vi "Sievert_auto_RLC-2.vi"() -> ()   [LabVIEW 2011]
uses:
  <vilib>/Utility/error.llb/DialogType.ctl
  <vilib>/DAQmx/write.llb/DAQmx Write (Digital Bool 1Line 1Point).vi
  <vilib>/DAQmx/create/channels.llb/DAQmx Create Channel (DO-Digital Output).vi
  <vilib>/DAQmx/miscellaneous.llb/DAQmx Fill In Error Info.vi
  <vilib>/Analysis/Matrix/Numeric/Conversions/Array To Matrix - RA.vi
  <vilib>/Analysis/Matrix/Numeric/Conversions/Matrix To Array - RM.vi
  <vilib>/Analysis/NI_AALPro.lvlib
  <vilib>/Analysis/Matrix/NI_Matrix.lvlib
  <vilib>/Analysis/NI_AALBase.lvlib
panel:
  out "Boolean 4":bool
  out "tempo carga":dbl[](array[numeric])
  out "PCh1":dbl[](array[numeric])
  out "output array 2":u32[](array[numeric])
  out "MEASURE C [F ]":dbl
  out "Automatico 2":dynamicdata(graph)
  out "termopar K 2":dbl format="%.3g"
  out "termopar K":string
  out "output NTC":dbl
  out "termopar K":dbl format="%.3g"
  out "path RLC_mean":path
  out "estagio 5":i32
  out "FIM":bool=TRUE
  out "limpo":i32
  in  "N fit":i32=5
  in  "ATM wait":u32
  in  "SET":i32
  in  "time subarray":dbl[](array[numeric])
  out "P cinetica mean 2":dbl format="%0.2f"
  out "T cinetica mean 3":dbl format="%0.2f"
  out "Time cinetica":dbl format="%0.2f"
  in  "T subarray 3":dbl[](array[numeric])
  in  "P T  index 2":i32
  in  "P subarray 2":dbl[](array[numeric])
  in  "Numeric":dbl=4.0
  in  "T subarray 2":dbl[](array[numeric])
  out "T cinetica mean 2":dbl format="%0.2f"
  out "P cinetica mean":dbl format="%0.2f"
  in  "P subarray":dbl[](array[numeric])
  in  "P T  index":i32
  out "T string":string
  out "P string":string
  out "path 2_cinetica":path
  out "Polynomial Coefficients 2":dbl[](array[numeric])
  out "Polynomial Coefficients":dbl[](array[numeric])
  in  "Count SET":i32=-1
  out "Set atual":i32
  out "mean pressure":dbl format="%.4p"
  out "Set number":i32
  in  "Tab Control":T1(tab)
  out "T":bool
  out "ZPf2":bool
  out "Pf2":bool
  out "Pit":bool
  out "ZPit":bool
  out "Camara":dbl(slide) scale=0.0..59.5 scale format="%#_3g"
  in  "Save manual":bool
  in  "Open Button":bool
  out "String 2":string
  in  "ATM":bool
  in  "Câmara":bool
  in  "Vácuo":bool
  in  "Entrada Gás":bool
  in  "Manual Ctrl":bool
  in  "stop":bool
  out "P-manual":dynamicdata(graph)
  in  "Clear":bool
  out "path":path
  in  "Nota":string
  in  "Sample name":string
  in  "File name":string
  out "Linear Model Graph":dbl[][](graph)
  out "Linear Model Graph 2":dbl[][](graph)
  in  "N to fit":i32=60
  out "N":i32
  out "Vácuo":bool
  out "Atm":bool
  out "Câmara":bool
  out "String_cinetica":string
  out "Vol Ref":dbl(slide) scale=0.0..60.0 scale format="%#_4f"
  out "Entrada gás":bool
  in  "Guardar\nCinetica":bool
  out "p fit":dbl format="%#_4g"
  out "T fit":dbl format="%#_4g"
  in  "Open Button 2":bool
  out "x >= y?":bool
  in  "seconds":dbl
  out "Elapsed Time (sec)":dbl format="%.1f"
  out "bar/N":dbl format="%#_4p"
  in  "correção NTC":dbl
  out "mean H2 sensor (V)":dbl format="%#_4p"
  out "Boolean 3":bool
  out "String 3":string
  out "T 2":bool
  out "ZPit 2":bool
  out "Pit 2":bool
  out "Pf2 2":bool
  out "ZPf2 2":bool
  out "Camara 2":dbl(slide) scale=0.0..20.0 scale format="%#_3g"
  out "Vácuo 2":bool
  out "Atm 2":bool
  out "Câmara 2":bool
  out "Vol Ref 3":dbl(slide) scale=0.0..25.0 scale format="%#_4f"
  out "Entrada gás 2":bool
  in  "Auto Ctrl":bool
  in  "Play Button":bool
  out "time stamp":timestamp format="%<%.2X>T"
  out "Time (sec)":dbl format="%.1f"
  in  "clear":bool
  out "Automatico":dynamicdata(graph)
  out "Linear P":T2(graph)
  out "Linear T":T2(graph)
  out "Contador":i32
  in  "STOP (bar/s)":dbl format="%#_5p"
  out "P (bar/s)":dbl format="%#_5p"
  out "bar/s":dbl format="%#_4p"
  out "P fit":dbl format="%#_4g"
  out "T fit":dbl format="%#_4g"
  out "x = y?":bool
  out "teste slope":i32
  in  "Set P auto":dbl
  in  "Step P":dbl=2.0
  in  "P_max":dbl=2.0
  in  "P_max camara":dbl=2.0
  out "Carga":bool=TRUE
  out "Descarga":bool
  out "String":string
  in  "P_min descarga":dbl
  in  "Boolean":bool
  in  "Array":dbl[](array[numeric])
  out "Boolean 2":bool
  out "Desc SET":i32
  in  "ZPf2 time":dbl=24.0
  in  "Ciclos":dbl
  out "Efetuados":dbl
  in  "patamar milliseconds to wait":u32=500
  in  "N fit patamar":i32=100
  in  "Step ZPit":dbl
  out "Read ZPit":bool
  in  "Estagio auto":i32
  out "mean H2 sensor":dbl format="%#_4p"
  in  "Ntest":i32=5
  in  "N fit 2":i32=100
  out "String 4":string
  in  "Combo Box":string(combo)
  in  "Refresh Button":bool
  in  "Close RLC 2":bool
  in  "RLC on/off":bool
  out "mean 16":dbl format="%.3p"
  out "mean 15":dbl format="%.3p"
  out "mean 14":dbl format="%.3p"
  out "mean 13":dbl format="%.3p"
  out "mean 12":dbl format="%.3p"
  out "mean 11":dbl format="%.3p"
  out "mean 10":dbl format="%.3p"
  out "mean 9":dbl format="%.3p"
  out "mean 8":dbl format="%.3p"
  out "mean 7":dbl format="%.3p"
  out "mean 6":dbl format="%.3p"
  out "mean 5":dbl format="%.3p"
  out "mean 4":dbl format="%.3p"
  out "mean 3":dbl format="%.3p"
  out "mean 2":dbl format="%.3p"
  out "mean":dbl format="%.3p"
  out "SET 2":dbl format="%#_3g"
  out "C-50-L":bool
  out "MEASURE B":dbl
  out "MEASURE A":dbl
  out "C-50-N":bool
  out "MEASURE B 2":dbl
  out "MEASURE A 2":dbl
  out "C-100-L":bool
  out "MEASURE B 3":dbl
  out "MEASURE A 3":dbl
  out "C-100-N":bool
  out "MEASURE B 4":dbl
  out "MEASURE A 4":dbl
  out "C-1K-L":bool
  out "MEASURE B 5":dbl
  out "MEASURE A 5":dbl
  out "C-1K-N":bool
  out "MEASURE B 6":dbl
  out "MEASURE A 6":dbl
  out "C-10K-L":bool
  out "MEASURE B 7":dbl
  out "MEASURE A 7":dbl
  out "C-10K-N":bool
  out "MEASURE B 8":dbl
  out "MEASURE A 8":dbl
  out "Z-50-L":bool
  out "MEASURE B 9":dbl
  out "MEASURE A 9":dbl
  out "Z-50-N":bool
  out "MEASURE B 10":dbl
  out "MEASURE A 10":dbl
  out "Z-100-L":bool
  out "MEASURE B 11":dbl
  out "MEASURE A 11":dbl
  out "Z-100-N":bool
  out "MEASURE B 12":dbl
  out "MEASURE A 12":dbl
  out "Z-1K-L":bool
  out "MEASURE B 13":dbl
  out "MEASURE A 13":dbl
  out "Z-1K-N":bool
  out "MEASURE B 14":dbl
  out "MEASURE A 14":dbl
  out "Z-10K-L":bool
  out "MEASURE B 15":dbl
  out "MEASURE A 15":dbl
  out "Z-10K-N":bool
  out "MEASURE B 16":dbl
  out "MEASURE A 16":dbl
  out "RLC300 - digimess":string
  in  "Time RLC":u32=5000
  in  "Ligar RLC":bool
  out "path RLC_completo":path
  out "Waveform Chart P 2":dbl[][](graph)
  out "Waveform Chart":dynamicdata(graph)
  in  "graph RLC":bool
  in  "Refresh Button 2":bool
  out "Waveform Chart 2":dynamicdata(graph)
  out "XY Graph 2":cluster{"Value":dbl[], "Value":dbl[]}[](graph)
  in  "t-sivert01(s)":dbl
  out "dP/dt (bar/s)":dbl format="%#_5p"
  in  "read - Sievert 01":bool
  # "P vol ref"
  # "P Câmara"
  # "P vol ref"
  # "P Câmara"
  # "C ( F )"
  # "R ( Ohm )"
  # "Z ( Ohm )"
  # "Phase ( deg)"
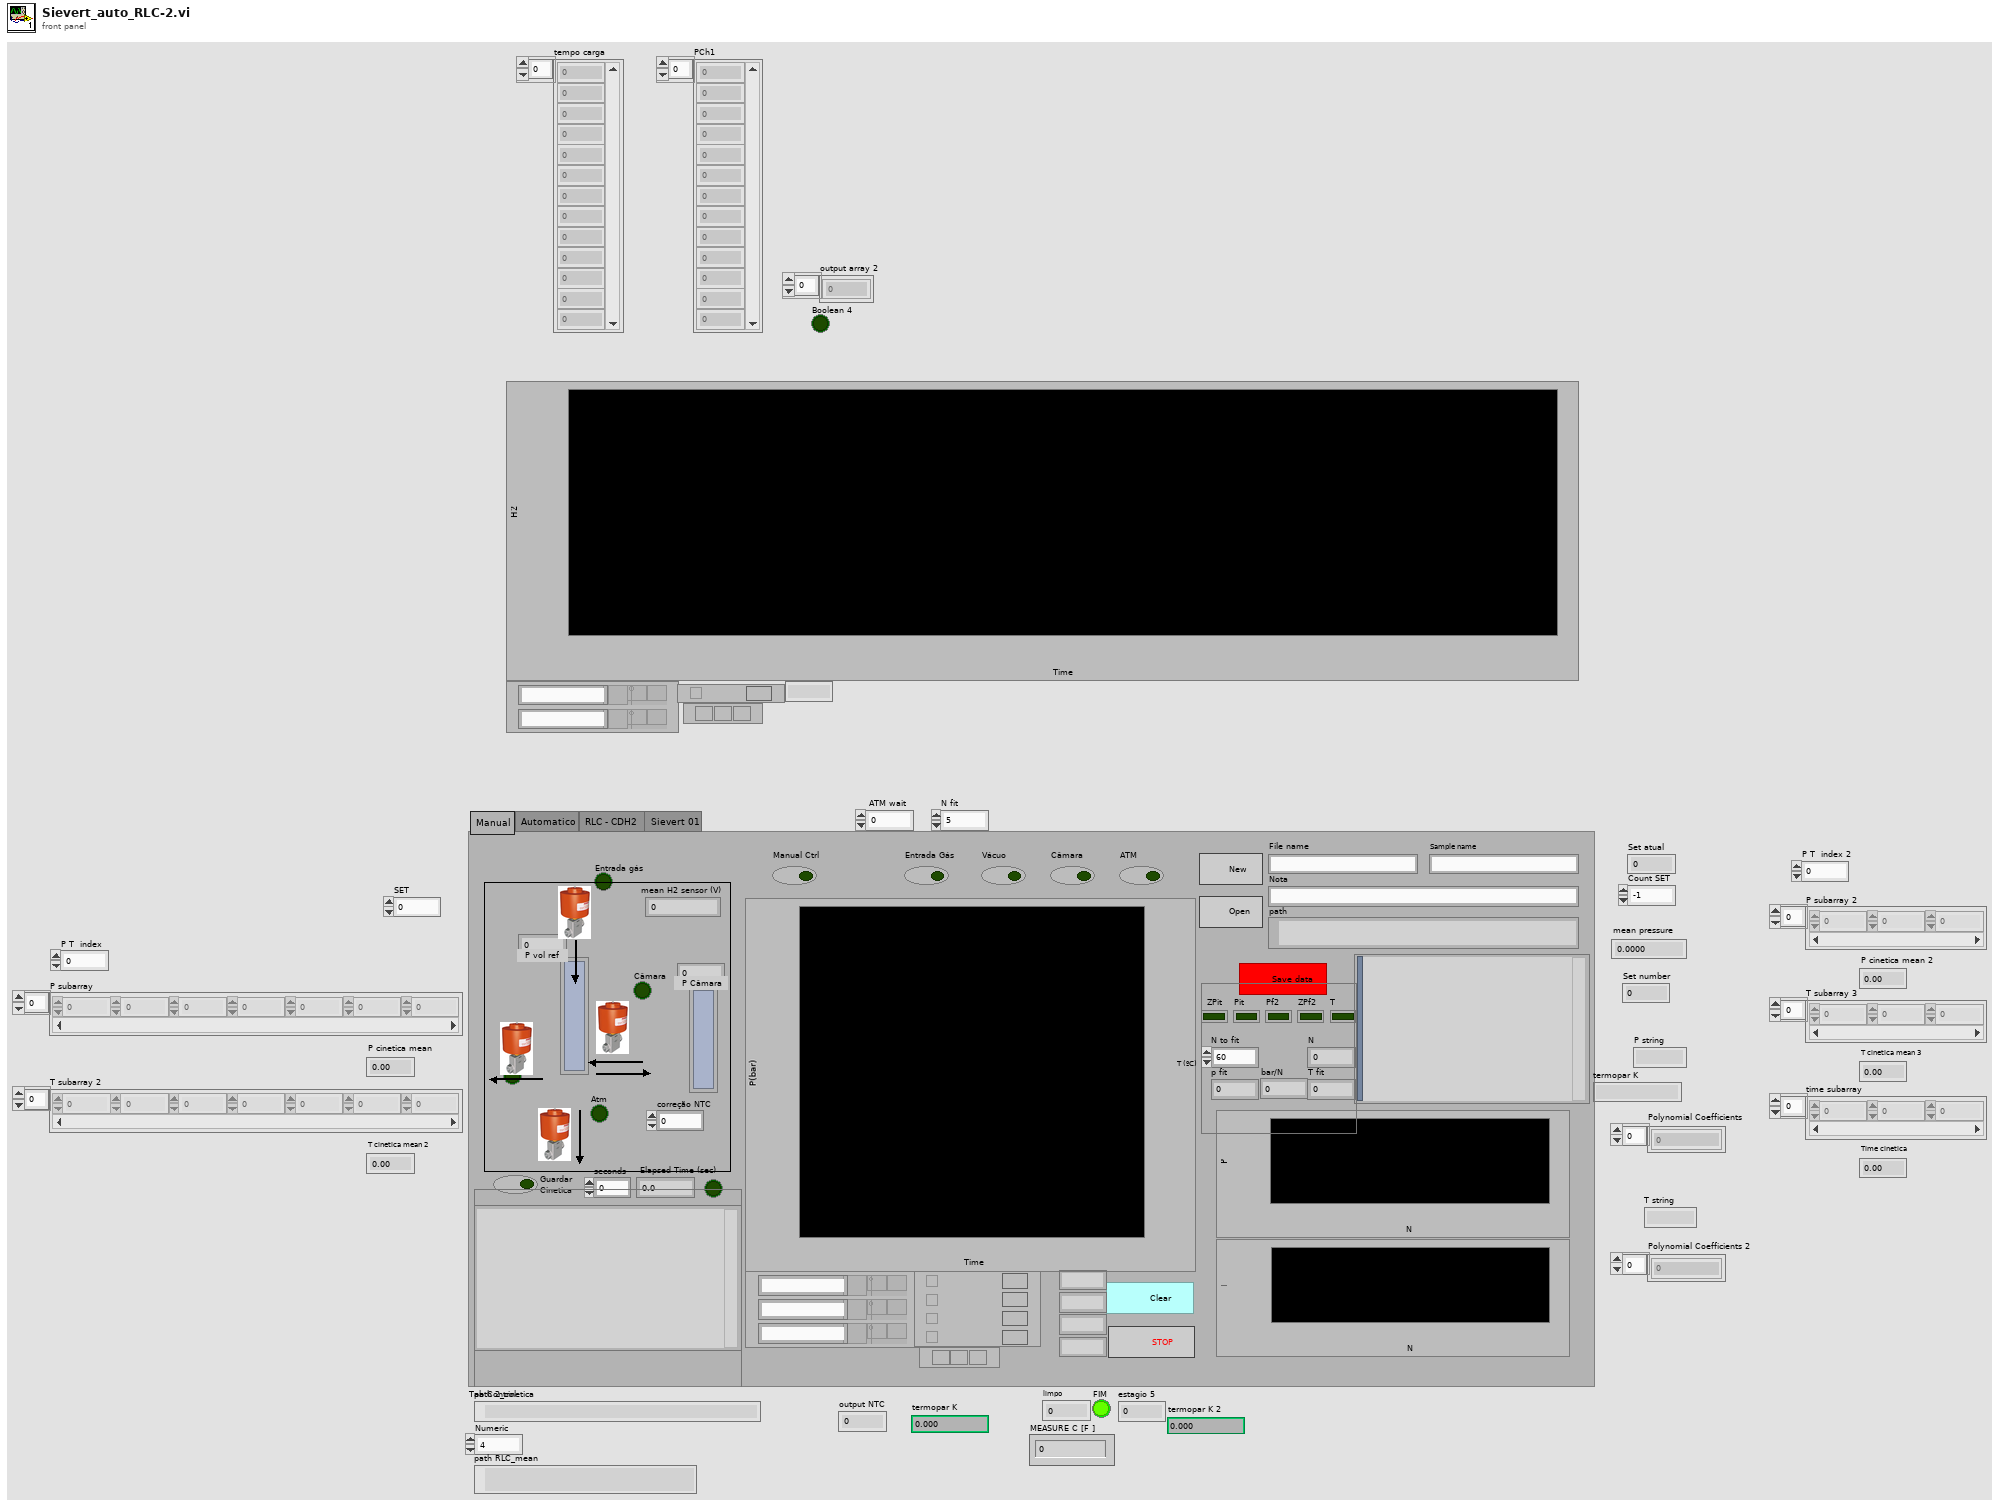
[diagram p1: front panel]
types:
  T1 = enum32{"Manual", "Automatico", "RLC - CDH2", "Sievert 01"}
  T2 = cluster{"Real 2D Array":dbl[], "Best Linear Fit":dbl[]}[]
  T3 = enum16{"open", "replace", "create", "open or create", "replace or create", "replace or create with confirmation"}
  T4 = cluster{"Value":dbl[], "Best Linear Fit":dbl[]}[]
  T5 = typedef "NI_Matrix.lvlib/RealMatrix.ctl" = dbl[][]
  T6 = cluster{"Real 2D Array":dbl[], "Real 2D Array":dbl[]}
  T7 = typedef "DialogType.ctl" = u16
  T8 = cluster{"Real 2D Array":dbl[], "Best Linear Fit":dbl[]}
  T9 = cluster{"Real 2D Array":dbl[], "Best Polynomial Fit":dbl[]}
  T10 = cluster{"Real 2D Array":dbl[], "Best Polynomial Fit":dbl[]}[]
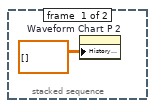
[diagram p5: hidden frame]
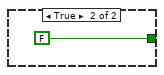
[diagram p10: hidden frame]
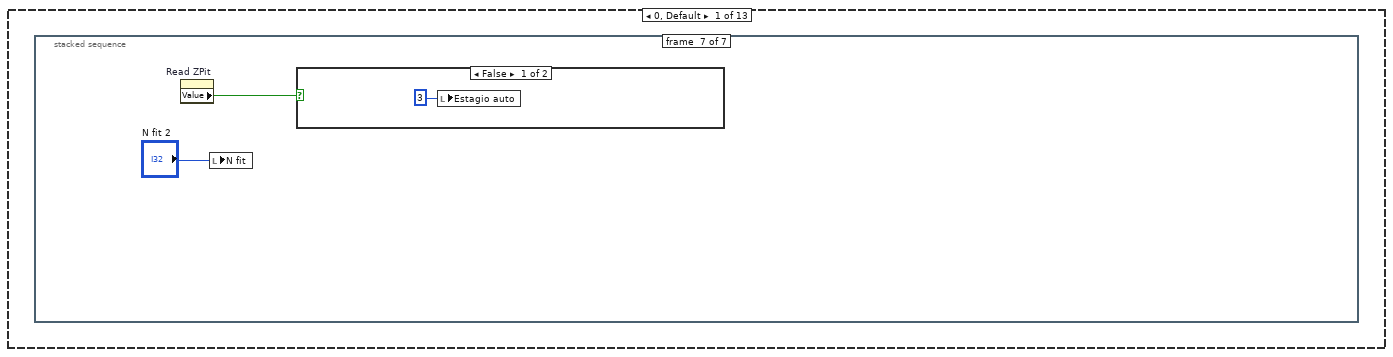
[diagram p15: hidden frame]
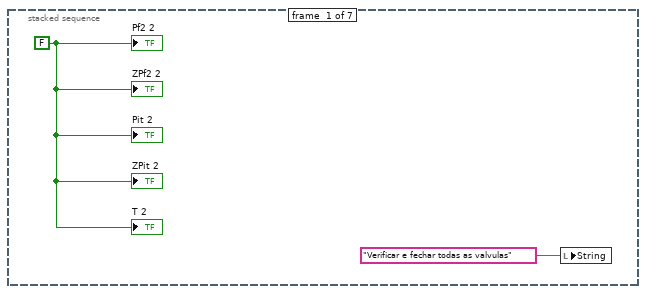
[diagram p16: hidden frame]
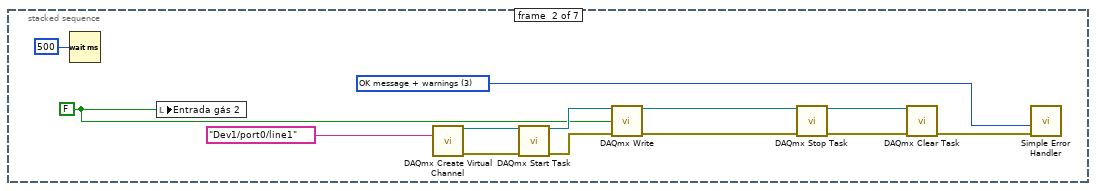
[diagram p17: hidden frame]
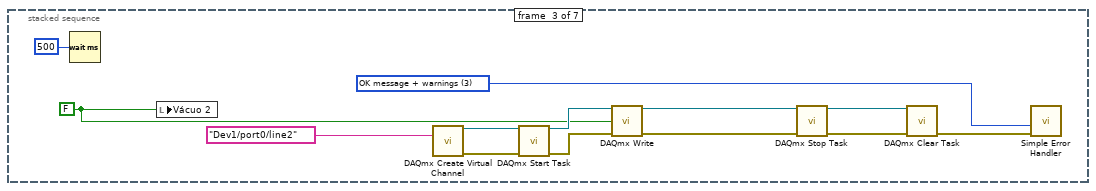
[diagram p18: hidden frame]
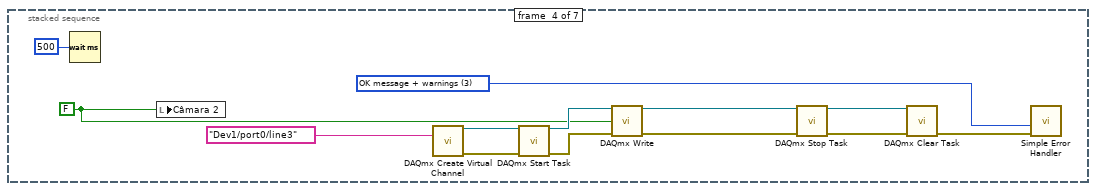
[diagram p19: hidden frame]
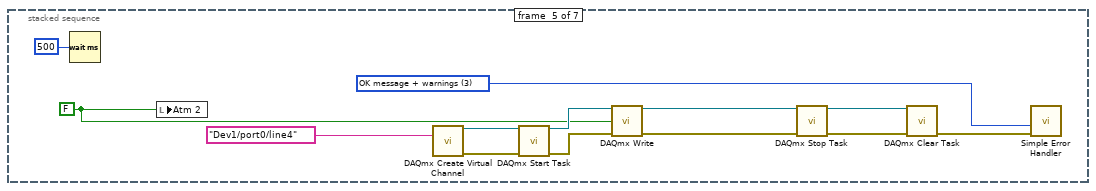
[diagram p20: hidden frame]
diagram:
  (unwired) dbl[] [0.5, 1.0, 2.0, 3.0, 4.0, 5.0, 6.0, 7.0, 8.0, 9.0, 10.0, 11.0, 12.0, 13.0, 14.0, 15.0, 16.0, 17.0, 18.0, 19.0, 20.0, 30.0, 40.0, 50.0, 60.0, 70.0] ("Array")
  n1 = local write "N to fit"(5 ("Numeric")) -> ()
  n2 = local write "correção NTC"(0.5 ("correção NTC")) -> ()
  n3 = local write "Step ZPit"(5.0 ("Step ZPit")) -> ()
  n4 = local write "Time RLC"(u32 5 ("Time RLC")) -> ()
  n5 = local write "Ciclos"(0.0 ("Ciclos")) -> ()
  n6 = local write "Desc SET"(0 ("Desc SET")) -> ()
  n7 = local write "Efetuados"(0.0 ("Efetuados")) -> ()
  n8 = local write "estagio 5"(0 ("estagio 5")) -> ()
  n9 = local write "teste slope"(0 ("teste slope")) -> ()
  n10 = local write "SET"(0 ("SET auto")) -> ()
  n11 = local write "limpo"(0 ("limpo")) -> ()
  n12 = local write "N fit"(5 ("N fit")) -> ()
  n13 = local write "ATM wait"(u32 4 ("ATM wait")) -> ()
  n14 = local write "Estagio auto"(0 ("Estagio auto")) -> ()
  n15 = local write "P T  index"(0 ("index")) -> ()
  n16 = local write "seconds"(2.0 ("seconds")) -> ()
  n17 = local write "Read ZPit"(TRUE ("Read ZPit")) -> ()
  n18 = local write "Descarga"(FALSE ("Descarga")) -> ()
  n19 = local write "Carga"(TRUE ("Carga")) -> ()
  n20 = local write "FIM"(FALSE ("FIM")) -> ()
  n21 = local write "P_max"(50.0 ("P_max")) -> ()
  n22 = local write "P_max camara"(25.0 ("P_max camara")) -> ()
  n23 = local write "Set P auto"(0.5 ("Set P auto")) -> ()
  n24 = local write "P_min descarga"(0.025 ("P_min descarga")) -> ()
  n25 = local write "P subarray"(dbl[] [0.0, 1.0] ("subarray")) -> ()
  n26 = local write "T subarray 2"(dbl[] [0.0, 1.0] ("subarray")) -> ()
  n27 = local write "Combo Box"("rlc_read_cCN.py" ("Combo Box")) -> ()
  n28 = local write "t-sivert01(s)"(10.0 ("t-sivert01(s)")) -> ()
  n29 = while {
    tunnel: path "C:/H2_Painel/painel_auto/RLC_CDH" ("Path") -> [w36]
    stop <- w48 stop-if-true
    n30 = property on="FIM" class="Bool (strict)"() -> ("Value"=w46:bool)  [unwired: 2 in, 2 out]
    n31 = property on="path" class="Path"() -> ("Value"=w43:path)  [unwired: 2 in, 2 out]
    n32 = case shown="True" "Ligar RLC" {
      tunnel: w36 -> [_ w223]
      frame False {
      }
      frame True {
        n33 = call "RLC_open.vi"("Path"=w223) -> ("String 2"=w224:string)  [unwired: 9 in, 1 out]
        n34 = local write "RLC300 - digimess"(w224) -> ()
      }
    }
    n35 = case shown="True" "Auto Ctrl" {
      tunnel: w36 -> [_ w229]
      tunnel: "RLC on/off" -> [_ w228]
      tunnel: [_ w227] -> w39
      frame False {
      }
      frame True {
        n36 = local write "P T  index 2"(0 ("P T  index")) -> ()
        n37 = for {
          N: "N fit" -> [w256]
          tunnel: w229 -> [w247]
          tunnel: w228 -> [w246]
          tunnel: [w245] -> w227
          i -> [w258]
          w262 = 0 ("polynomial order")
          w253 = 0 ("polynomial order")
          n38 = case shown="True" "clear" {
            frame False {
            }
            frame True {
              n39 = property on="Automatico 2" class="WFChart (strict)"("History Data"=dynamicdata[] []) -> ()  [unwired: 2 in, 2 out]
              n40 = property on="Linear P" class="XYGraph (strict)"("Value"=T2 [] ("Linear P")) -> ()  [unwired: 2 in, 2 out]
              n41 = property on="Linear T" class="XYGraph (strict)"("Value"=T2 [] ("Linear T")) -> ()  [unwired: 2 in, 2 out]
              n42 = property on="Automatico" class="WFChart (strict)"("History Data"=dynamicdata[] []) -> ()  [unwired: 2 in, 2 out]
            }
          }
          n43 = property on="path 2_cinetica" class="Path"() -> ("Value"=w250:path)  [unwired: 2 in, 2 out]
          n44 = call "Read P T.vi"("correção NTC"="correção NTC") -> ("Sievert01"=w237:dbl, "mean H2 sensor"=w242:dbl, "termopar K"=w239:dbl, "output NTC"=w240:dbl, "P Set 2 Output 2"=w241:dbl)  [unwired: 3 in, 7 out]
          "termopar K 2" <- w239
          "mean H2 sensor" <- w242
          n45 = Increment(x=w258) -> (x+1=w257:i32)
          n46 = Equal?(x=w257, y=w256) -> (x = y?=w259:bool)
          "x = y?" <- w259
          n47 = Merge Signals(w242) -> (→"Automatico 2":dynamicdata)
          n48 = Multiply(x=w241, y=10.0) -> (x*y=w252:dbl)
          n49 = Multiply(x=w237, y=10.0) -> (x*y=w236:dbl)
          n50 = case shown="True" "read - Sievert 01" {
            tunnel: w236 -> [_ w285]
            frame False {
            }
            frame True {
              n51 = Merge Signals(w285) -> (→"Waveform Chart 2":dynamicdata)
              n52 = flat-sequence {
                tunnel: w285 -> [w302]
                tunnel: [w300] -> w287
                frame #0 {
                  n53 = property on="Boolean 4" class="Bool (strict)"() -> ("Value"=w288:bool)  [unwired: 2 in, 2 out]
                  n54 = case shown="True" w288 {
                    frame False {
                    }
                    frame True {
                      n55 = local write "PCh1"(dbl[] [] ("PCh1")) -> ()
                      n56 = local write "tempo carga"(dbl[] [] ("tempo carga")) -> ()
                      n57 = local write "output array 2"(u32[] [] ("output array 2")) -> ()
                    }
                  }
                }
                frame #1 {
                  n58 = Tick Count (ms)() -> (millisecond timer value=w313:u32)
                  n59 = property on="output array 2" class="Arr (strict)"() -> ("Value"=w314:u32[])  [unwired: 2 in, 2 out]
                  n60 = Build Array(w313) -> (w307:u32[])
                  n61 = Insert Into Array(array=w314, new element=w307) -> (w308:u32[])  [unwired: 1 in]
                  "output array 2" <- w308
                  n62 = Array Max & Min(array=w308) -> (max value=w312:u32, min value=w311:u32)  [unwired: 2 out]
                  n63 = Subtract(x=w312, y=w311) -> (x-y=w309:u32)
                  n64 = Divide(x=w309, y=1000.0) -> (x/y=w299:dbl)
                  n65 = property on="PCh1" class="Arr (strict)"() -> ("Value"=w304:dbl[])  [unwired: 2 in, 2 out]
                  n66 = property on="tempo carga" class="Arr (strict)"() -> ("Value"=w305:dbl[])  [unwired: 2 in, 2 out]
                  n67 = Greater?(x=w299, y="t-sivert01(s)") -> (0:w300:bool)
                  n68 = Build Array(w299) -> (w306:dbl[])
                  n69 = Build Array(w302) -> (w303:dbl[])
                  n70 = Insert Into Array(array=w305, new element=w306) -> (w294:dbl[])  [unwired: 1 in]
                  "tempo carga" <- w294
                  n71 = Insert Into Array(array=w304, new element=w303) -> (w293:dbl[])  [unwired: 1 in]
                  "PCh1" <- w293
                  n72 = call <vilib>:"Linear Fit.vi"("Y"=w293, "X"=w294) -> ("Best Linear Fit"=w292:dbl[], "slope"=→"dP/dt (bar/s)":dbl)  [unwired: 9 in, 3 out]
                  n73 = Bundle("Value"=w294, "Value"=w293) -> (w297:cluster{"Value":dbl[], "Value":dbl[]})  [unwired: 1 in]
                  n74 = Bundle("Value"=w294, "Best Linear Fit"=w292) -> (w296:cluster{"Value":dbl[], "Best Linear Fit":dbl[]})  [unwired: 1 in]
                  n75 = Build Array(w297, w296) -> (→"XY Graph 2":T4)
                }
              }
              "Boolean 4" <- w287
            }
          }
          n76 = local write "Vol Ref 3"(w252) -> ()
          n77 = Merge Signals(w252, w240, w239, w236) -> (→"Automatico":dynamicdata)
          n78 = call "Elapsed Time2"("Reset"=w259) -> ("Elapsed Time (s)"=w273:dbl)  [unwired: 11 in, 7 out]
          "Time (sec)" <- w273
          n79 = stacked-sequence {
            tunnel: w252 -> [w1623 _]
            tunnel: w240 -> [w1609 _]
            tunnel: [w1590 _] -> w271
            tunnel: [w1606 _] -> w270
            tunnel: w273 -> [w1593 _]
            tunnel: [w1591 _] -> w267
            tunnel: [w1589 _] -> w249
            tunnel: [w1588 _] -> w248
            frame #0 {
              w1592 = 2 ("y")
              n80 = property on="P subarray 2" class="Arr (strict)"() -> ("Value"=w1625:dbl[])  [unwired: 2 in, 2 out]
              n81 = property on="T subarray 3" class="Arr (strict)"() -> ("Value"=w1615:dbl[])  [unwired: 2 in, 2 out]
              n82 = property on="time subarray" class="Arr (strict)"() -> ("Value"=w1602:dbl[])  [unwired: 2 in, 2 out]
              n83 = property on="P T  index 2" class="DigNum (strict)"() -> ("Value"=w1594:i32)  [unwired: 2 in, 2 out]
              n84 = Replace Array Subset(array=w1602, new element=w1593, index=w1594) -> (w1595:dbl[])
              n85 = Replace Array Subset(array=w1625, new element=w1623, index=w1594) -> (w1608:dbl[])
              n86 = Replace Array Subset(array=w1615, new element=w1609, index=w1594) -> (w1607:dbl[])
              n87 = call-poly <vilib>:"Array To Matrix.vi"("Real 1D Array"=w1595) -> ("Real Matrix (Column Vector)"=w1605:T5)
              n88 = call-poly <vilib>:"Array To Matrix.vi"("Real 1D Array"=w1608) -> ("Real Matrix (Column Vector)"=w1628:T5)
              n89 = call-poly <vilib>:"Array To Matrix.vi"("Real 1D Array"=w1607) -> ("Real Matrix (Column Vector)"=w1618:T5)
              n90 = Matrix Size(0:w1605) -> (1:w1604:i32, 2:w1603:i32)
              n91 = Matrix Size(0:w1628) -> (1:w1627:i32, 2:w1626:i32)
              n92 = Matrix Size(0:w1618) -> (1:w1617:i32, 2:w1616:i32)
              n93 = Increment(x=w1604) -> (x+1=w1596:i32)
              n94 = Increment(x=w1627) -> (x+1=w1619:i32)
              n95 = Increment(x=w1617) -> (x+1=w1610:i32)
              n96 = Subtract(x=w1596, y=w1592) -> (x-y=w1597:i32)
              n97 = Subtract(x=w1619, y=w1592) -> (x-y=w1620:i32)
              n98 = Subtract(x=w1610, y=w1592) -> (x-y=w1611:i32)
              n99 = Resize Matrix(1:w1603, 2:w1596, 4:w1605) -> (0:w1601:T5)
              n100 = Resize Matrix(1:w1626, 2:w1619, 4:w1628) -> (0:w1624:T5)
              n101 = Resize Matrix(1:w1616, 2:w1610, 4:w1618) -> (0:w1614:T5)
              n102 = call-poly <vilib>:"Matrix To Array.vi"("Real Matrix"=w1601) -> ("Real 2D Array"=w1599:dbl[][])
              n103 = call-poly <vilib>:"Matrix To Array.vi"("Real Matrix"=w1624) -> ("Real 2D Array"=w1622:dbl[][])
              n104 = call-poly <vilib>:"Matrix To Array.vi"("Real Matrix"=w1614) -> ("Real 2D Array"=w1613:dbl[][])
              n105 = Reshape Array(w1599, w1596) -> (w1598:dbl[])
              n106 = Reshape Array(w1622, w1619) -> (w1621:dbl[])
              n107 = Reshape Array(w1613, w1610) -> (w1612:dbl[])
              n108 = local write "time subarray"(w1598) -> ()
              n109 = local write "P subarray 2"(w1621) -> ()
              n110 = local write "T subarray 3"(w1612) -> ()
              n111 = Reshape Array(w1598, w1597) -> (w1591:dbl[])
              n112 = Reshape Array(w1621, w1620) -> (w1590:dbl[])
              n113 = Reshape Array(w1612, w1611) -> (w1606:dbl[])
              n114 = call <vilib>:"Mean.vi"("X"=w1591) -> ("mean"=→"Time cinetica":dbl)  [unwired: 1 out]
              n115 = call <vilib>:"Mean.vi"("X"=w1590) -> ("mean"=w1589:dbl)  [unwired: 1 out]
              "P cinetica mean 2" <- w1589
              n116 = call <vilib>:"Mean.vi"("X"=w1606) -> ("mean"=w1588:dbl)  [unwired: 1 out]
              "T cinetica mean 3" <- w1588
            }
            frame #1 {
              n117 = property on="P T  index 2" class="DigNum (strict)"() -> ("Value"=w1630:i32)  [unwired: 2 in, 2 out]
              n118 = Increment(x=w1630) -> (x+1=w1629:i32)
              n119 = local write "P T  index 2"(w1629) -> ()
            }
          }
          n120 = To Time Stamp(1:w273) -> (0:→"time stamp":timestamp)
          n121 = call <vilib>:"Linear Fit.vi"("Y"=w270, "X"=w267) -> ("Best Linear Fit"=w279:dbl[])  [unwired: 9 in, 4 out]
          n122 = Bundle("Real 2D Array"=w267, "Real 2D Array"=w270) -> (w277:T6)  [unwired: 1 in]
          n123 = Bundle("Real 2D Array"=w267, "Real 2D Array"=w271) -> (w276:T6)  [unwired: 1 in]
          n124 = call <vilib>:"General Polynomial Fit.vi"("Y"=w270, "polynomial order"=w253, "X"=w267) -> ("Best Polynomial Fit"=w268:dbl[], "Polynomial Coefficients"=w263:dbl[])  [unwired: 9 in, 2 out]
          n125 = call <vilib>:"General Polynomial Fit.vi"("Y"=w271, "polynomial order"=w253, "X"=w267) -> ("Best Polynomial Fit"=w269:dbl[], "Polynomial Coefficients"=w264:dbl[])  [unwired: 9 in, 2 out]
          n126 = call <vilib>:"Linear Fit.vi"("Y"=w271, "X"=w267) -> ("Best Linear Fit"=w274:dbl[], "slope"=w254:dbl)  [unwired: 9 in, 3 out]
          "bar/s" <- w254
          n127 = property on="path" class="Path"() -> ("Value"=w251:path)  [unwired: 2 in, 2 out]
          n128 = case shown="True" "Play Button" {
            tunnel: w251 -> [_ w323]
            tunnel: w252 -> [_ w322]
            tunnel: w250 -> [_ w321]
            tunnel: w249 -> [_ w320]
            tunnel: w248 -> [_ w319]
            tunnel: w247 -> [_ w318]
            tunnel: w246 -> [_ w317]
            tunnel: [_ w316] -> w245
            tunnel: w239 -> [_ w315]
            frame False {
            }
            frame True {
              n129 = case shown="12" "Estagio auto" {
                tunnel: w323 -> [_ _ _ w415 _ _ w568 _ w717 _ _ w1429 w1498]
                tunnel: w322 -> [_ w389 _ _ w464 w515 _ _ _ w1347 _ _ _]
                tunnel: w321 -> [_ _ _ _ _ _ _ w607 _ _ _ _ _]
                tunnel: w320 -> [_ _ _ _ _ _ _ w606 _ _ _ _ _]
                tunnel: w319 -> [_ _ _ _ _ _ _ w605 _ _ _ _ _]
                tunnel: w318 -> [_ _ _ _ _ _ _ _ w696 _ _ _ _]
                tunnel: w317 -> [_ _ _ _ _ _ _ _ w713 _ _ _ _]
                tunnel: [_ _ _ _ _ _ _ _ w695 _ _ _ _] -> w316
                tunnel: w315 -> [_ _ _ _ _ _ _ _ _ _ _ w1425 _]
                frame 0, Default {
                  n130 = stacked-sequence {
                    frame #0 {
                      w325 = FALSE ("Pit")
                      n131 = local write "String"("Verificar e fechar todas as valvulas" ("String")) -> ()
                      "ZPf2 2" <- w325
                      "Pf2 2" <- w325
                      "Pit 2" <- w325
                      "ZPit 2" <- w325
                      "T 2" <- w325
                    }
                    frame #1 {
                      w328 = FALSE ("Boolean 4")
                      w333 = T7 3 items=["no dialog", "OK message", "continue or stop message", "OK message + warnings", "continue/stop + warnings"] ("type of dialog (OK msg:1)")
                      n132 = Wait (ms)(milliseconds to wait=u32 500) -> ()  [unwired: 1 out]
                      n133 = local write "Entrada gás 2"(w328) -> ()
                      n134 = call-poly <vilib>:"DAQmx Create Virtual Channel.vi"("lines"=tag "Dev1/port0/line1") -> ("task out"=w331:refnum<k21>, "error out"=w332:errorcluster)  [unwired: 13 in]
                      n135 = call <vilib>:"DAQmx Start Task.vi"("task/channels in"=w331, "error in"=w332) -> ("task out"=w334:refnum<k21>, "error out"=w335:errorcluster)  [unwired: 12 in]
                      n136 = call-poly <vilib>:"DAQmx Write.vi"("task/channels in"=w334, "data"=w328, "error in"=w335) -> ("task out"=w339:refnum<k21>, "error out"=w336:errorcluster)  [unwired: 10 in, 1 out]
                      n137 = call <vilib>:"DAQmx Stop Task.vi"("task/channels in"=w339, "error in"=w336) -> ("task out"=w338:refnum<k21>, "error out"=w337:errorcluster)  [unwired: 12 in]
                      n138 = call <vilib>:"DAQmx Clear Task.vi"("task in"=w338, "error in"=w337) -> ("error out"=w330:errorcluster)  [unwired: 13 in]
                      n139 = call <vilib>:"Simple Error Handler.vi"("type of dialog (OK msg:1)"=w333, "error in (no error)"=w330) -> ()  [unwired: 3 in, 5 out]
                    }
                    frame #2 {
                      w341 = FALSE ("Boolean 4")
                      w346 = T7 3 items=["no dialog", "OK message", "continue or stop message", "OK message + warnings", "continue/stop + warnings"] ("type of dialog (OK msg:1)")
                      n140 = Wait (ms)(milliseconds to wait=u32 500) -> ()  [unwired: 1 out]
                      n141 = local write "Vácuo 2"(w341) -> ()
                      n142 = call-poly <vilib>:"DAQmx Create Virtual Channel.vi"("lines"=tag "Dev1/port0/line2") -> ("task out"=w344:refnum<k21>, "error out"=w345:errorcluster)  [unwired: 13 in]
                      n143 = call <vilib>:"DAQmx Start Task.vi"("task/channels in"=w344, "error in"=w345) -> ("task out"=w347:refnum<k21>, "error out"=w348:errorcluster)  [unwired: 12 in]
                      n144 = call-poly <vilib>:"DAQmx Write.vi"("task/channels in"=w347, "data"=w341, "error in"=w348) -> ("task out"=w352:refnum<k21>, "error out"=w349:errorcluster)  [unwired: 10 in, 1 out]
                      n145 = call <vilib>:"DAQmx Stop Task.vi"("task/channels in"=w352, "error in"=w349) -> ("task out"=w351:refnum<k21>, "error out"=w350:errorcluster)  [unwired: 12 in]
                      n146 = call <vilib>:"DAQmx Clear Task.vi"("task in"=w351, "error in"=w350) -> ("error out"=w343:errorcluster)  [unwired: 13 in]
                      n147 = call <vilib>:"Simple Error Handler.vi"("type of dialog (OK msg:1)"=w346, "error in (no error)"=w343) -> ()  [unwired: 3 in, 5 out]
                    }
                    frame #3 {
                      w354 = FALSE ("Boolean 4")
                      w359 = T7 3 items=["no dialog", "OK message", "continue or stop message", "OK message + warnings", "continue/stop + warnings"] ("type of dialog (OK msg:1)")
                      n148 = Wait (ms)(milliseconds to wait=u32 500) -> ()  [unwired: 1 out]
                      n149 = local write "Câmara 2"(w354) -> ()
                      n150 = call-poly <vilib>:"DAQmx Create Virtual Channel.vi"("lines"=tag "Dev1/port0/line3") -> ("task out"=w357:refnum<k21>, "error out"=w358:errorcluster)  [unwired: 13 in]
                      n151 = call <vilib>:"DAQmx Start Task.vi"("task/channels in"=w357, "error in"=w358) -> ("task out"=w360:refnum<k21>, "error out"=w361:errorcluster)  [unwired: 12 in]
                      n152 = call-poly <vilib>:"DAQmx Write.vi"("task/channels in"=w360, "data"=w354, "error in"=w361) -> ("task out"=w365:refnum<k21>, "error out"=w362:errorcluster)  [unwired: 10 in, 1 out]
                      n153 = call <vilib>:"DAQmx Stop Task.vi"("task/channels in"=w365, "error in"=w362) -> ("task out"=w364:refnum<k21>, "error out"=w363:errorcluster)  [unwired: 12 in]
                      n154 = call <vilib>:"DAQmx Clear Task.vi"("task in"=w364, "error in"=w363) -> ("error out"=w356:errorcluster)  [unwired: 13 in]
                      n155 = call <vilib>:"Simple Error Handler.vi"("type of dialog (OK msg:1)"=w359, "error in (no error)"=w356) -> ()  [unwired: 3 in, 5 out]
                    }
                    frame #4 {
                      w367 = FALSE ("Boolean 4")
                      w372 = T7 3 items=["no dialog", "OK message", "continue or stop message", "OK message + warnings", "continue/stop + warnings"] ("type of dialog (OK msg:1)")
                      n156 = Wait (ms)(milliseconds to wait=u32 500) -> ()  [unwired: 1 out]
                      n157 = local write "Atm 2"(w367) -> ()
                      n158 = call-poly <vilib>:"DAQmx Create Virtual Channel.vi"("lines"=tag "Dev1/port0/line4") -> ("task out"=w370:refnum<k21>, "error out"=w371:errorcluster)  [unwired: 13 in]
                      n159 = call <vilib>:"DAQmx Start Task.vi"("task/channels in"=w370, "error in"=w371) -> ("task out"=w373:refnum<k21>, "error out"=w374:errorcluster)  [unwired: 12 in]
                      n160 = call-poly <vilib>:"DAQmx Write.vi"("task/channels in"=w373, "data"=w367, "error in"=w374) -> ("task out"=w378:refnum<k21>, "error out"=w375:errorcluster)  [unwired: 10 in, 1 out]
                      n161 = call <vilib>:"DAQmx Stop Task.vi"("task/channels in"=w378, "error in"=w375) -> ("task out"=w377:refnum<k21>, "error out"=w376:errorcluster)  [unwired: 12 in]
                      n162 = call <vilib>:"DAQmx Clear Task.vi"("task in"=w377, "error in"=w376) -> ("error out"=w369:errorcluster)  [unwired: 13 in]
                      n163 = call <vilib>:"Simple Error Handler.vi"("type of dialog (OK msg:1)"=w372, "error in (no error)"=w369) -> ()  [unwired: 3 in, 5 out]
                    }
                    frame #5 {
                      n164 = Wait (ms)(milliseconds to wait=u32 500) -> ()  [unwired: 1 out]
                    }
                    frame #6 {
                      n165 = property on="Read ZPit" class="Bool (strict)"() -> ("Value"=w381:bool)  [unwired: 2 in, 2 out]
                      n166 = local write "N fit"("N fit 2") -> ()
                      n167 = case shown="False" w381 {
                        frame False {
                          n168 = local write "Estagio auto"(3 ("Estagio auto")) -> ()
                        }
                        frame True {
                          n169 = local write "Estagio auto"(1 ("Estagio auto")) -> ()
                        }
                      }
                    }
                  }
                }
                frame 1 {
                  n170 = Greater?(x=w389, y=1.0) -> (0:w388:bool)
                  n171 = case shown="True" w388 {
                    tunnel: [FALSE ("Boolean") TRUE ("Boolean")] -> w385
                    frame False {
                      w401 = TRUE ("Boolean")
                      n172 = local write "Vácuo 2"(w401) -> ()
                      n173 = call "Controle_vacuo.vi"("time (s) to wait vacuo"=u32 5, "Boolean"=w401) -> ("Vacuo"=w402:bool)  [unwired: 9 in]
                      n174 = local write "Vácuo 2"(w402) -> ()
                      n175 = local write "String"("Limpar volume referencia" ("String")) -> ()
                    }
                    frame True {
                      n176 = call "Controle_ATM.vi"("seconds to wait"="ATM wait") -> ("String 2"=w406:string, "Atm"=w405:bool)  [unwired: 9 in]
                      n177 = local write "Atm 2"(w405) -> ()
                      n178 = local write "String"(w406) -> ()
                    }
                  }
                  n179 = for {
                    N: 1 -> [_]
                    tunnel: [w391] -> w386
                    tunnel: w385 -> [w391]
                    n180 = Wait (ms)(milliseconds to wait=u32 500 ("x")) -> ()  [unwired: 1 out]
                  }
                  n181 = case shown="True" w386 {
                    frame False {
                      n182 = local write "Estagio auto"(2 ("Estagio auto")) -> ()
                    }
                    frame True {
                      w396 = TRUE ("Boolean")
                      n183 = local write "Estagio auto"(2 ("Estagio auto")) -> ()
                      n184 = local write "Vácuo 2"(w396) -> ()
                      n185 = call "Controle_vacuo.vi"("time (s) to wait vacuo"=u32 5, "Boolean"=w396) -> ("Vacuo"=w397:bool)  [unwired: 9 in]
                      n186 = local write "Vácuo 2"(w397) -> ()
                      n187 = local write "String"("Limpar volume referencia" ("String")) -> ()
                    }
                  }
                }
                frame 2 {
                  n188 = property on="Contador" class="DigNum (strict)"() -> ("Value"=w410:i32)  [unwired: 2 in, 2 out]
                  n189 = local write "String"("Ler ZPit" ("String")) -> ()
                  n190 = Increment(x=w410) -> (x+1=w409:i32)
                  n191 = property on="N fit 2" class="DigNum (strict)"() -> ("Value"=w407:i32)  [unwired: 2 in, 2 out]
                  n192 = Equal?(x=w409, y=w407) -> (x = y?=w408:bool)
                  n193 = case shown="True" w408 {
                    frame False {
                    }
                    frame True {
                      n194 = local write "Estagio auto"(3 ("Estagio auto")) -> ()
                    }
                  }
                }
                frame 3 {
                  w418 = "\t"
                  n195 = property on="SET" class="DigNum (strict)"() -> ("Value"=w414:i32)  [unwired: 2 in, 2 out]
                  n196 = property on="Read ZPit" class="Bool (strict)"() -> ("Value"=w413:bool)  [unwired: 2 in, 2 out]
                  n197 = case shown="False" w413 {
                    tunnel: ["  ==>" w425] -> w419
                    frame False {
                    }
                    frame True {
                      n198 = property on="P fit" class="DigNum (strict)"() -> ("Value"=w424:dbl)  [unwired: 2 in, 2 out]
                      n199 = Number To Fractional String(number=w424, precision (6)=i16 3) -> (F-format string=w425:string)  [unwired: 2 in]
                    }
                  }
                  n200 = Number To Decimal String(number=w414) -> (decimal integer string=w417:string)  [unwired: 1 in]
                  n201 = Concatenate Strings(w417, w418, w419, w418) -> (w416:string)
                  n202 = flat-sequence {
                    tunnel: [w429] -> w421
                    tunnel: [w428] -> w420
                    tunnel: w416 -> [w427]
                    tunnel: w415 -> [w426]
                    tunnel: w421 -> [w445]
                    tunnel: w420 -> [w444]
                    frame #0 {
                      n203 = Open/Create/Replace File(file path (use dialog)=w426, operation (0:open)=T3."open") -> (refnum out=w435:refnum<file>, error out=w436:errorcluster)  [unwired: 2 in, 3 out]
                      n204 = Set File Position(refnum=w435, from (0:start)=enum16{"start", "end", "current"}."end", error in=w436) -> (refnum out=w433:refnum<file>, error out=w432:errorcluster)  [unwired: 1 in]
                      n205 = Write to Text File(file (use dialog)=w433, text=w427, error in=w432) -> (refnum out=w437:refnum<file>, error out=w438:errorcluster)  [unwired: 2 out]
                      n206 = Close File(refnum=w437, error in=w438) -> (path=w429:path, error out=w430:errorcluster)
                      n207 = call <vilib>:"Simple Error Handler.vi"("error in (no error)"=w430) -> ("error out"=w428:errorcluster)  [unwired: 1 in, 7 out]
                    }
                    frame #1 {
                      w439 = 0 ("limpo")
                      n208 = local write "Estagio auto"(4 ("Estagio auto")) -> ()
                      n209 = local write "ZPit 2"(TRUE ("ZPit")) -> ()
                      n210 = Wait (ms)(milliseconds to wait=u32 500) -> ()  [unwired: 1 out]
                      n211 = local write "limpo"(w439) -> ()
                      n212 = Read from Text File(file (use dialog)=w445, count=-1 ("Count  3"), error in=w444) -> (refnum out=w446:refnum<file>, text=w450:string, error out=w447:errorcluster)  [unwired: 1 in, 1 out]
                      n213 = local write "String 3"(w450) -> ()
                      n214 = local write "estagio 5"(w439) -> ()
                      n215 = Close File(refnum=w446, error in=w447) -> (error out=w448:errorcluster)  [unwired: 1 out]
                      n216 = call <vilib>:"Simple Error Handler.vi"("error in (no error)"=w448) -> ()  [unwired: 1 in, 8 out]
                      n217 = local write "String"("abrir valvula entrada gas" ("String")) -> ()
                    }
                    frame #2 {
                      w451 = T7 3 items=["no dialog", "OK message", "continue or stop message", "OK message + warnings", "continue/stop + warnings"] ("type of dialog (OK msg:1)")
                      w457 = TRUE ("Boolean 4")
                      n218 = local write "Entrada gás 2"(w457) -> ()
                      n219 = call-poly <vilib>:"DAQmx Create Virtual Channel.vi"("lines"=tag "Dev1/port0/line1") -> ("task out"=w459:refnum<k21>, "error out"=w460:errorcluster)  [unwired: 13 in]
                      n220 = call <vilib>:"DAQmx Start Task.vi"("task/channels in"=w459, "error in"=w460) -> ("task out"=w461:refnum<k21>, "error out"=w462:errorcluster)  [unwired: 12 in]
                      n221 = call-poly <vilib>:"DAQmx Write.vi"("task/channels in"=w461, "data"=w457, "error in"=w462) -> ("task out"=w454:refnum<k21>, "error out"=w453:errorcluster)  [unwired: 10 in, 1 out]
                      n222 = call <vilib>:"DAQmx Stop Task.vi"("task/channels in"=w454, "error in"=w453) -> ("task out"=w455:refnum<k21>, "error out"=w456:errorcluster)  [unwired: 12 in]
                      n223 = call <vilib>:"DAQmx Clear Task.vi"("task in"=w455, "error in"=w456) -> ("error out"=w452:errorcluster)  [unwired: 13 in]
                      n224 = call <vilib>:"Simple Error Handler.vi"("type of dialog (OK msg:1)"=w451, "error in (no error)"=w452) -> ()  [unwired: 3 in, 5 out]
                    }
                  }
                }
                frame 4 {
                  n225 = Greater Or Equal?(x=w464, y="Set P auto") -> (x >= y?=w465:bool)
                  n226 = case shown="True" w465 {
                    tunnel: "Set P auto" -> [_ w480]
                    frame False {
                      w473 = T7 3 items=["no dialog", "OK message", "continue or stop message", "OK message + warnings", "continue/stop + warnings"] ("type of dialog (OK msg:1)")
                      w479 = TRUE ("data")
                      n227 = local write "Estagio auto"(5 ("Estagio auto")) -> ()
                      n228 = Wait (ms)(milliseconds to wait=u32 500) -> ()  [unwired: 1 out]
                      n229 = local write "Entrada gás 2"(w479) -> ()
                      n230 = call-poly <vilib>:"DAQmx Create Virtual Channel.vi"("lines"=tag "Dev1/port0/line1") -> ("task out"=w470:refnum<k21>, "error out"=w469:errorcluster)  [unwired: 13 in]
                      n231 = call <vilib>:"DAQmx Start Task.vi"("task/channels in"=w470, "error in"=w469) -> ("task out"=w468:refnum<k21>, "error out"=w467:errorcluster)  [unwired: 12 in]
                      n232 = call-poly <vilib>:"DAQmx Write.vi"("task/channels in"=w468, "data"=w479, "error in"=w467) -> ("task out"=w476:refnum<k21>, "error out"=w475:errorcluster)  [unwired: 10 in, 1 out]
                      n233 = call <vilib>:"DAQmx Stop Task.vi"("task/channels in"=w476, "error in"=w475) -> ("task out"=w478:refnum<k21>, "error out"=w477:errorcluster)  [unwired: 12 in]
                      n234 = call <vilib>:"DAQmx Clear Task.vi"("task in"=w478, "error in"=w477) -> ("error out"=w474:errorcluster)  [unwired: 13 in]
                      n235 = call <vilib>:"Simple Error Handler.vi"("type of dialog (OK msg:1)"=w473, "error in (no error)"=w474) -> ()  [unwired: 3 in, 5 out]
                    }
                    frame True {
                      n236 = flat-sequence {
                        tunnel: [w483] -> w481
                        tunnel: w480 -> [w483]
                        tunnel: [w498] -> w482
                        tunnel: w481 -> [w497]
                        tunnel: w482 -> [w512]
                        frame #0 {
                          w489 = T7 3 items=["no dialog", "OK message", "continue or stop message", "OK message + warnings", "continue/stop + warnings"] ("type of dialog (OK msg:1)")
                          w496 = FALSE ("data")
                          n237 = Wait (ms)(milliseconds to wait=u32 500) -> ()  [unwired: 1 out]
                          n238 = local write "Entrada gás 2"(w496) -> ()
                          n239 = call-poly <vilib>:"DAQmx Create Virtual Channel.vi"("lines"=tag "Dev1/port0/line1") -> ("task out"=w487:refnum<k21>, "error out"=w488:errorcluster)  [unwired: 13 in]
                          n240 = call <vilib>:"DAQmx Start Task.vi"("task/channels in"=w487, "error in"=w488) -> ("task out"=w485:refnum<k21>, "error out"=w484:errorcluster)  [unwired: 12 in]
                          n241 = call-poly <vilib>:"DAQmx Write.vi"("task/channels in"=w485, "data"=w496, "error in"=w484) -> ("task out"=w493:refnum<k21>, "error out"=w492:errorcluster)  [unwired: 10 in, 1 out]
                          n242 = call <vilib>:"DAQmx Stop Task.vi"("task/channels in"=w493, "error in"=w492) -> ("task out"=w495:refnum<k21>, "error out"=w494:errorcluster)  [unwired: 12 in]
                          n243 = call <vilib>:"DAQmx Clear Task.vi"("task in"=w495, "error in"=w494) -> ("error out"=w490:errorcluster)  [unwired: 13 in]
                          n244 = call <vilib>:"Simple Error Handler.vi"("type of dialog (OK msg:1)"=w489, "error in (no error)"=w490) -> ()  [unwired: 3 in, 5 out]
                        }
                        frame #1 {
                          n245 = stacked-sequence {
                            tunnel: [_ _ _ w509] -> w498
                            tunnel: w497 -> [_ _ w502 _]
                            frame #0 {
                              n246 = call "Controle_ATM.vi"("seconds to wait"=2.0) -> ("Atm"=w500:bool)  [unwired: 9 in, 1 out]
                              n247 = local write "Atm 2"(w500) -> ()
                            }
                            frame #1 {
                              n248 = Wait (ms)(milliseconds to wait=u32 1000) -> ()  [unwired: 1 out]
                            }
                            frame #2 {
                              n249 = Less Or Equal?(x=w502, y=1.5) -> (x <= y?=w504:bool)
                              n250 = case shown="True" w504 {
                                frame False {
                                n251 = call "Controle_ATM.vi"("seconds to wait"=2.0) -> ()  [unwired: 9 in, 2 out]
                                }
                                frame True {
                                w507 = TRUE ("Vácuo")
                                n252 = local write "Vácuo 2"(w507) -> ()
                                n253 = call "Controle_vacuo.vi"("time (s) to wait vacuo"=3.0, "Boolean"=w507) -> ("Vacuo"=w508:bool)  [unwired: 9 in]
                                n254 = local write "Vácuo 2"(w508) -> ()
                                }
                              }
                            }
                            frame #3 {
                              n255 = property on="limpo" class="DigNum (strict)"() -> ("Value"=w510:i32)  [unwired: 2 in, 2 out]
                              n256 = Wait (ms)(milliseconds to wait=u32 1000) -> ()  [unwired: 1 out]
                              n257 = Increment(x=w510) -> (x+1=w509:i32)
                            }
                          }
                        }
                        frame #2 {
                          "limpo" <- w512
                        }
                      }
                    }
                  }
                }
                frame 5 {
                  n258 = property on="Set P auto" class="DigNum (strict)"() -> ("Value"=w514:dbl)  [unwired: 2 in, 2 out]
                  n259 = Greater Or Equal?(x=w515, y=w514) -> (x >= y?=w513:bool)
                  n260 = case shown="True" w513 {
                    selector: w513 -> [_ w537]
                    frame False {
                      n261 = flat-sequence {
                        tunnel: [w517] -> w516
                        tunnel: w516 -> [w533]
                        frame #0 {
                          w520 = T7 3 items=["no dialog", "OK message", "continue or stop message", "OK message + warnings", "continue/stop + warnings"] ("type of dialog (OK msg:1)")
                          w530 = TRUE ("Boolean 4")
                          n262 = property on="estagio 5" class="DigNum (strict)"() -> ("Value"=w518:i32)  [unwired: 2 in, 2 out]
                          n263 = local write "Entrada gás 2"(w530) -> ()
                          n264 = Increment(x=w518) -> (x+1=w517:i32)
                          n265 = call-poly <vilib>:"DAQmx Create Virtual Channel.vi"("lines"=tag "Dev1/port0/line1") -> ("task out"=w524:refnum<k21>, "error out"=w523:errorcluster)  [unwired: 13 in]
                          n266 = call <vilib>:"DAQmx Start Task.vi"("task/channels in"=w524, "error in"=w523) -> ("task out"=w522:refnum<k21>, "error out"=w521:errorcluster)  [unwired: 12 in]
                          n267 = call-poly <vilib>:"DAQmx Write.vi"("task/channels in"=w522, "data"=w530, "error in"=w521) -> ("task out"=w527:refnum<k21>, "error out"=w526:errorcluster)  [unwired: 10 in, 1 out]
                          n268 = call <vilib>:"DAQmx Stop Task.vi"("task/channels in"=w527, "error in"=w526) -> ("task out"=w528:refnum<k21>, "error out"=w529:errorcluster)  [unwired: 12 in]
                          n269 = call <vilib>:"DAQmx Clear Task.vi"("task in"=w528, "error in"=w529) -> ("error out"=w519:errorcluster)  [unwired: 13 in]
                          n270 = call <vilib>:"Simple Error Handler.vi"("type of dialog (OK msg:1)"=w520, "error in (no error)"=w519) -> ()  [unwired: 3 in, 5 out]
                        }
                        frame #1 {
                          n271 = Less?(x=w533, y=6) -> (x < y?=w531:bool)
                          n272 = case shown="False" w531 {
                            frame False {
                              n273 = local write "Estagio auto"(5 ("Estagio auto")) -> ()
                            }
                            frame True {
                              n274 = local write "Estagio auto"(4 ("Estagio auto")) -> ()
                            }
                          }
                          "estagio 5" <- w533
                        }
                      }
                    }
                    frame True {
                      n275 = flat-sequence {
                        tunnel: w537 -> [w538]
                        tunnel: [w538] -> w536
                        tunnel: w536 -> [w554]
                        frame #0 {
                          w539 = FALSE ("Boolean 4")
                          w544 = T7 3 items=["no dialog", "OK message", "continue or stop message", "OK message + warnings", "continue/stop + warnings"] ("type of dialog (OK msg:1)")
                          n276 = local write "Entrada gás 2"(w539) -> ()
                          n277 = call-poly <vilib>:"DAQmx Create Virtual Channel.vi"("lines"=tag "Dev1/port0/line1") -> ("task out"=w542:refnum<k21>, "error out"=w543:errorcluster)  [unwired: 13 in]
                          n278 = call <vilib>:"DAQmx Start Task.vi"("task/channels in"=w542, "error in"=w543) -> ("task out"=w545:refnum<k21>, "error out"=w546:errorcluster)  [unwired: 12 in]
                          n279 = call-poly <vilib>:"DAQmx Write.vi"("task/channels in"=w545, "data"=w539, "error in"=w546) -> ("task out"=w550:refnum<k21>, "error out"=w547:errorcluster)  [unwired: 10 in, 1 out]
                          n280 = call <vilib>:"DAQmx Stop Task.vi"("task/channels in"=w550, "error in"=w547) -> ("task out"=w549:refnum<k21>, "error out"=w548:errorcluster)  [unwired: 12 in]
                          n281 = call <vilib>:"DAQmx Clear Task.vi"("task in"=w549, "error in"=w548) -> ("error out"=w541:errorcluster)  [unwired: 13 in]
                          n282 = call <vilib>:"Simple Error Handler.vi"("type of dialog (OK msg:1)"=w544, "error in (no error)"=w541) -> ()  [unwired: 3 in, 5 out]
                        }
                        frame #1 {
                          n283 = property on="estagio 5" class="DigNum (strict)"() -> ("Value"=w552:i32)  [unwired: 2 in, 2 out]
                          n284 = Greater?(x=w552, y=5) -> (0:w555:bool)
                          n285 = And(x=w554, y=w555) -> (x .and. y?=w553:bool)
                          n286 = case shown="True" w553 {
                            frame False {
                              n287 = local write "Estagio auto"(4 ("Estagio auto")) -> ()
                              n288 = Wait (ms)(milliseconds to wait=u32 500) -> ()  [unwired: 1 out]
                            }
                            frame True {
                              n289 = property on="Contador" class="DigNum (strict)"() -> ("Value"=w559:i32)  [unwired: 2 in, 2 out]
                              n290 = local write "String"("Ler Pit" ("String")) -> ()
                              n291 = Increment(x=w559) -> (x+1=w561:i32)
                              n292 = property on="N fit 2" class="DigNum (strict)"() -> ("Value"=w558:i32)  [unwired: 2 in, 2 out]
                              n293 = Equal?(x=w561, y=w558) -> (x = y?=w560:bool)
                              n294 = case shown="True" w560 {
                                frame False {
                                }
                                frame True {
                                n295 = local write "Estagio auto"(6 ("Estagio auto")) -> ()
                                }
                              }
                            }
                          }
                        }
                      }
                    }
                  }
                }
                frame 6 {
                  n296 = property on="Contador" class="DigNum (strict)"() -> ("Value"=w565:i32)  [unwired: 2 in, 2 out]
                  n297 = Increment(x=w565) -> (x+1=w567:i32)
                  n298 = property on="N fit 2" class="DigNum (strict)"() -> ("Value"=w564:i32)  [unwired: 2 in, 2 out]
                  n299 = Equal?(x=w567, y=w564) -> (x = y?=w566:bool)
                  n300 = case shown="True" w566 {
                    tunnel: w568 -> [_ w569]
                    frame False {
                    }
                    frame True {
                      n301 = property on="P fit" class="DigNum (strict)"() -> ("Value"=w570:dbl)  [unwired: 2 in, 2 out]
                      n302 = Number To Fractional String(number=w570, precision (6)=i16 3) -> (F-format string=w574:string)  [unwired: 2 in]
                      n303 = Concatenate Strings(w574, "\t") -> (w572:string)
                      n304 = flat-sequence {
                        tunnel: [w580] -> w576
                        tunnel: [w579] -> w575
                        tunnel: w572 -> [w578]
                        tunnel: w569 -> [w577]
                        tunnel: w576 -> [w596]
                        tunnel: w575 -> [w595]
                        frame #0 {
                          n305 = Open/Create/Replace File(file path (use dialog)=w577, operation (0:open)=T3."open") -> (refnum out=w586:refnum<file>, error out=w587:errorcluster)  [unwired: 2 in, 3 out]
                          n306 = Set File Position(refnum=w586, from (0:start)=enum16{"start", "end", "current"}."end", error in=w587) -> (refnum out=w584:refnum<file>, error out=w583:errorcluster)  [unwired: 1 in]
                          n307 = Write to Text File(file (use dialog)=w584, text=w578, error in=w583) -> (refnum out=w588:refnum<file>, error out=w589:errorcluster)  [unwired: 2 out]
                          n308 = Close File(refnum=w588, error in=w589) -> (path=w580:path, error out=w581:errorcluster)
                          n309 = call <vilib>:"Simple Error Handler.vi"("error in (no error)"=w581) -> ("error out"=w579:errorcluster)  [unwired: 1 in, 7 out]
                        }
                        frame #1 {
                          n310 = local write "Estagio auto"(7 ("Estagio auto")) -> ()
                          n311 = local write "teste slope"(0 ("teste slope")) -> ()
                          n312 = local write "Pit 2"(TRUE ("ZPit")) -> ()
                          n313 = Wait (ms)(milliseconds to wait=u32 500) -> ()  [unwired: 1 out]
                          n314 = Read from Text File(file (use dialog)=w596, count=-1 ("Count  3"), error in=w595) -> (refnum out=w597:refnum<file>, text=w601:string, error out=w598:errorcluster)  [unwired: 1 in, 1 out]
                          n315 = local write "String 3"(w601) -> ()
                          n316 = Close File(refnum=w597, error in=w598) -> (error out=w599:errorcluster)  [unwired: 1 out]
                          n317 = call <vilib>:"Simple Error Handler.vi"("error in (no error)"=w599) -> ()  [unwired: 1 in, 8 out]
                          n318 = local write "String"("abrir valvula entrada camara" ("String")) -> ()
                        }
                      }
                    }
                  }
                }
                frame 7 {
                  n319 = flat-sequence {
                    tunnel: w605 -> [w609]
                    tunnel: w606 -> [w610]
                    tunnel: w607 -> [w611]
                    tunnel: [w611] -> w604
                    tunnel: [w610] -> w603
                    tunnel: [w609] -> w602
                    tunnel: w604 -> [w615]
                    tunnel: w603 -> [w614]
                    tunnel: w602 -> [w613]
                    frame #0 {
                      n320 = local write "N fit"("N fit patamar") -> ()
                    }
                    frame #1 {
                      n321 = flat-sequence {
                        tunnel: w615 -> [w627]
                        tunnel: w614 -> [w626]
                        tunnel: w613 -> [w625]
                        frame #0 {
                          w640 = "\t"
                          w646 = i16 4 ("precision (6)")
                          n322 = Number To Fractional String(number=w626, precision (6)=w646) -> (F-format string=w641:string)  [unwired: 2 in]
                          n323 = Number To Fractional String(number=w625, precision (6)=w646) -> (F-format string=w639:string)  [unwired: 2 in]
                          n324 = Open/Create/Replace File(file path (use dialog)=w627, operation (0:open)=T3."open") -> (refnum out=w635:refnum<file>, error out=w628:errorcluster)  [unwired: 2 in, 3 out]
                          n325 = Get Date/Time String(date format (0)=enum16{"short", "long", "abbreviated"}."short", want seconds? (F)=TRUE) -> (date string=w643:string, time string=w642:string)  [unwired: 1 in]
                          n326 = Set File Position(refnum=w635, from (0:start)=enum16{"start", "end", "current"}."end", error in=w628) -> (refnum out=w633:refnum<file>, error out=w632:errorcluster)  [unwired: 1 in]
                          n327 = Concatenate Strings(w643, w640, w642, w640, w641, w640, w639, "\r\n") -> (w629:string)
                          n328 = Write to Text File(file (use dialog)=w633, text=w629, error in=w632) -> (refnum out=w636:refnum<file>, error out=w637:errorcluster)  [unwired: 2 out]
                          n329 = Close File(refnum=w636, error in=w637) -> (error out=w630:errorcluster)  [unwired: 1 out]
                          n330 = call <vilib>:"Simple Error Handler.vi"("error in (no error)"=w630) -> ()  [unwired: 1 in, 8 out]
                        }
                      }
                      n331 = property on="Contador" class="DigNum (strict)"() -> ("Value"=w623:i32)  [unwired: 2 in, 2 out]
                      n332 = Increment(x=w623) -> (x+1=w622:i32)
                      n333 = property on="N fit patamar" class="DigNum (strict)"() -> ("Value"=w612:i32)  [unwired: 2 in, 2 out]
                      n334 = Equal?(x=w622, y=w612) -> (x = y?=w624:bool)
                      n335 = case shown="True" w624 {
                        tunnel: [FALSE w651] -> w621
                        tunnel: [_ w650] -> w620
                        frame False {
                        }
                        frame True {
                          n336 = property on="P (bar/s)" class="DigNum (strict)"() -> ("Value"=w653:dbl)  [unwired: 2 in, 2 out]
                          n337 = Absolute Value(x=w653) -> (abs(x)=w652:dbl)
                          n338 = Less Or Equal?(x=w652, y="STOP (bar/s)") -> (x <= y?=w651:bool)
                          n339 = case shown="True" w651 {
                            tunnel: [_ w655] -> w650
                            frame False {
                            }
                            frame True {
                              n340 = property on="teste slope" class="DigNum (strict)"() -> ("Value"=w656:i32)  [unwired: 2 in, 2 out]
                              n341 = local write "Estagio auto"(7 ("Estagio auto")) -> ()
                              n342 = Increment(x=w656) -> (x+1=w655:i32)
                              "teste slope" <- w655
                            }
                          }
                        }
                      }
                      n343 = Greater Or Equal?(x=w620, y="Ntest") -> (x >= y?=w618:bool)
                      n344 = And(x=w624, y=w618) -> (x .and. y?=w617:bool)
                      n345 = case shown="True" w617 {
                        frame False {
                        }
                        frame True {
                          n346 = flat-sequence {
                            frame #0 {
                              n347 = property on="N fit 2" class="DigNum (strict)"() -> ("Value"=w686:i32)  [unwired: 2 in, 2 out]
                              n348 = Wait (ms)(milliseconds to wait=u32 500) -> ()  [unwired: 1 out]
                              n349 = local write "N fit"(w686) -> ()
                            }
                            frame #1 {
                              n350 = local write "Estagio auto"(8 ("Estagio auto")) -> ()
                            }
                          }
                        }
                      }
                      n351 = case shown="True" w617 {
                        tunnel: [TRUE ("Boolean") FALSE ("Boolean")] -> w616
                        frame False {
                        }
                        frame True {
                        }
                      }
                      n352 = case shown="True" w621 {
                        tunnel: w616 -> [_ w672]
                        frame False {
                          w670 = T7 3 items=["no dialog", "OK message", "continue or stop message", "OK message + warnings", "continue/stop + warnings"] ("type of dialog (OK msg:1)")
                          w666 = TRUE ("Boolean")
                          n353 = case shown="True" w666 {
                            frame False {
                            }
                            frame True {
                              n354 = property on="Vol Ref 3" class="Slide (strict)"() -> ("Value"=w671:dbl)  [unwired: 2 in, 2 out]
                              n355 = local write "Camara 2"(w671) -> ()
                            }
                          }
                          n356 = local write "Câmara 2"(w666) -> ()
                          n357 = call-poly <vilib>:"DAQmx Create Virtual Channel.vi"("lines"=tag "Dev1/port0/line3") -> ("task out"=w659:refnum<k21>, "error out"=w660:errorcluster)  [unwired: 13 in]
                          n358 = Wait (ms)(milliseconds to wait="patamar milliseconds to wait") -> ()  [unwired: 1 out]
                          n359 = call <vilib>:"DAQmx Start Task.vi"("task/channels in"=w659, "error in"=w660) -> ("task out"=w661:refnum<k21>, "error out"=w662:errorcluster)  [unwired: 12 in]
                          n360 = call-poly <vilib>:"DAQmx Write.vi"("task/channels in"=w661, "data"=w666, "error in"=w662) -> ("task out"=w667:refnum<k21>, "error out"=w668:errorcluster)  [unwired: 10 in, 1 out]
                          n361 = call <vilib>:"DAQmx Stop Task.vi"("task/channels in"=w667, "error in"=w668) -> ("task out"=w664:refnum<k21>, "error out"=w663:errorcluster)  [unwired: 12 in]
                          n362 = call <vilib>:"DAQmx Clear Task.vi"("task in"=w664, "error in"=w663) -> ("error out"=w669:errorcluster)  [unwired: 13 in]
                          n363 = call <vilib>:"Simple Error Handler.vi"("type of dialog (OK msg:1)"=w670, "error in (no error)"=w669) -> ()  [unwired: 3 in, 5 out]
                        }
                        frame True {
                          n364 = flat-sequence {
                            tunnel: w672 -> [w673]
                            frame #0 {
                              w675 = T7 3 items=["no dialog", "OK message", "continue or stop message", "OK message + warnings", "continue/stop + warnings"] ("type of dialog (OK msg:1)")
                              n365 = local write "Câmara 2"(w673) -> ()
                              n366 = call-poly <vilib>:"DAQmx Create Virtual Channel.vi"("lines"=tag "Dev1/port0/line3") -> ("task out"=w684:refnum<k21>, "error out"=w683:errorcluster)  [unwired: 13 in]
                              n367 = call <vilib>:"DAQmx Start Task.vi"("task/channels in"=w684, "error in"=w683) -> ("task out"=w682:refnum<k21>, "error out"=w681:errorcluster)  [unwired: 12 in]
                              n368 = call-poly <vilib>:"DAQmx Write.vi"("task/channels in"=w682, "data"=w673, "error in"=w681) -> ("task out"=w677:refnum<k21>, "error out"=w676:errorcluster)  [unwired: 10 in, 1 out]
                              n369 = call <vilib>:"DAQmx Stop Task.vi"("task/channels in"=w677, "error in"=w676) -> ("task out"=w679:refnum<k21>, "error out"=w680:errorcluster)  [unwired: 12 in]
                              n370 = call <vilib>:"DAQmx Clear Task.vi"("task in"=w679, "error in"=w680) -> ("error out"=w674:errorcluster)  [unwired: 13 in]
                              n371 = call <vilib>:"Simple Error Handler.vi"("type of dialog (OK msg:1)"=w675, "error in (no error)"=w674) -> ()  [unwired: 3 in, 5 out]
                            }
                            frame #1 {
                              n372 = Wait (ms)(milliseconds to wait=u32 2000) -> ()  [unwired: 1 out]
                            }
                          }
                        }
                      }
                    }
                  }
                }
                frame 8 {
                  n373 = property on="Contador" class="DigNum (strict)"() -> ("Value"=w715:i32)  [unwired: 2 in, 2 out]
                  n374 = Increment(x=w715) -> (x+1=w716:i32)
                  n375 = property on="N fit 2" class="DigNum (strict)"() -> ("Value"=w689:i32)  [unwired: 2 in, 2 out]
                  n376 = Equal?(x=w716, y=w689) -> (x = y?=w714:bool)
                  n377 = case shown="False" w713 {
                    tunnel: [FALSE ("Save manual") w1310] -> w693
                    tunnel: w714 -> [_ w1310]
                    frame False {
                    }
                    frame True {
                    }
                  }
                  n378 = case shown="False" w714 {
                    tunnel: w717 -> [_ w1311]
                    frame False {
                    }
                    frame True {
                      n379 = property on="P fit" class="DigNum (strict)"() -> ("Value"=w1312:dbl)  [unwired: 2 in, 2 out]
                      n380 = Number To Fractional String(number=w1312, precision (6)=i16 3) -> (F-format string=w1316:string)  [unwired: 2 in]
                      n381 = Concatenate Strings(w1316, "\t") -> (w1314:string)
                      n382 = flat-sequence {
                        tunnel: [w1323] -> w1318
                        tunnel: [w1322] -> w1317
                        tunnel: w1314 -> [w1321]
                        tunnel: w1311 -> [w1320]
                        tunnel: w1318 -> [w1338]
                        tunnel: w1317 -> [w1337]
                        frame #0 {
                          n383 = Wait (ms)(milliseconds to wait=u32 500) -> ()  [unwired: 1 out]
                          n384 = Open/Create/Replace File(file path (use dialog)=w1320, operation (0:open)=T3."open") -> (refnum out=w1329:refnum<file>, error out=w1330:errorcluster)  [unwired: 2 in, 3 out]
                          n385 = Set File Position(refnum=w1329, from (0:start)=enum16{"start", "end", "current"}."end", error in=w1330) -> (refnum out=w1327:refnum<file>, error out=w1326:errorcluster)  [unwired: 1 in]
                          n386 = Write to Text File(file (use dialog)=w1327, text=w1321, error in=w1326) -> (refnum out=w1331:refnum<file>, error out=w1332:errorcluster)  [unwired: 2 out]
                          n387 = Close File(refnum=w1331, error in=w1332) -> (path=w1323:path, error out=w1324:errorcluster)
                          n388 = call <vilib>:"Simple Error Handler.vi"("error in (no error)"=w1324) -> ("error out"=w1322:errorcluster)  [unwired: 1 in, 7 out]
                        }
                        frame #1 {
                          n389 = local write "Estagio auto"(9 ("Estagio auto")) -> ()
                          n390 = local write "Pf2 2"(TRUE ("ZPit")) -> ()
                          n391 = Wait (ms)(milliseconds to wait=u32 500) -> ()  [unwired: 1 out]
                          n392 = Read from Text File(file (use dialog)=w1338, count=-1 ("Count  3"), error in=w1337) -> (refnum out=w1339:refnum<file>, text=w1343:string, error out=w1340:errorcluster)  [unwired: 1 in, 1 out]
                          n393 = local write "String 3"(w1343) -> ()
                          n394 = Close File(refnum=w1339, error in=w1340) -> (error out=w1341:errorcluster)  [unwired: 1 out]
                          n395 = local write "String"("abrir valvula vacuo" ("String")) -> ()
                          n396 = call <vilib>:"Simple Error Handler.vi"("error in (no error)"=w1341) -> ()  [unwired: 1 in, 8 out]
                        }
                      }
                    }
                  }
                  n397 = flat-sequence {
                    tunnel: w693 -> [w719]
                    tunnel: w696 -> [w720]
                    tunnel: [w720] -> w691
                    tunnel: [w719] -> w690
                    tunnel: [w722] -> w712
                    tunnel: [w724] -> w711
                    tunnel: [w725] -> w710
                    tunnel: [w726] -> w709
                    tunnel: [w727] -> w708
                    tunnel: [w728] -> w707
                    tunnel: [w729] -> w706
                    tunnel: [w730] -> w705
                    tunnel: [w731] -> w704
                    tunnel: [w732] -> w703
                    tunnel: [w733] -> w702
                    tunnel: [w734] -> w701
                    tunnel: [w735] -> w700
                    tunnel: [w736] -> w699
                    tunnel: [w737] -> w698
                    tunnel: [w723] -> w697
                    tunnel: [w721] -> w694
                    tunnel: w691 -> [w739]
                    tunnel: w690 -> [w738]
                    tunnel: w712 -> [w1260]
                    tunnel: w711 -> [w1259]
                    tunnel: w710 -> [w1258]
                    tunnel: w709 -> [w1257]
                    tunnel: w708 -> [w1256]
                    tunnel: w707 -> [w1255]
                    tunnel: w706 -> [w1254]
                    tunnel: w705 -> [w1253]
                    tunnel: w704 -> [w1252]
                    tunnel: w703 -> [w1251]
                    tunnel: w702 -> [w1250]
                    tunnel: w701 -> [w1249]
                    tunnel: w700 -> [w1248]
                    tunnel: w699 -> [w1247]
                    tunnel: w698 -> [w1246]
                    tunnel: w697 -> [w1245]
                    tunnel: [w1243] -> w695
                    tunnel: w694 -> [w1243]
                    tunnel: [TRUE ("graph RLC")] -> w692
                    frame #0 {
                      n398 = local write "graph RLC"(FALSE) -> ()
                    }
                    frame #1 {
                      n399 = case shown="False" w738 {
                        tunnel: [FALSE w776] -> w721
                        tunnel: w739 -> [_ w758]
                        tunnel: [_ w756] -> w722
                        tunnel: [_ w755] -> w723
                        tunnel: [_ w754] -> w724
                        tunnel: [_ w753] -> w725
                        tunnel: [_ w752] -> w726
                        tunnel: [_ w751] -> w727
                        tunnel: [_ w750] -> w728
                        tunnel: [_ w749] -> w729
                        tunnel: [_ w748] -> w730
                        tunnel: [_ w747] -> w731
                        tunnel: [_ w746] -> w732
                        tunnel: [_ w745] -> w733
                        tunnel: [_ w744] -> w734
                        tunnel: [_ w743] -> w735
                        tunnel: [_ w742] -> w736
                        tunnel: [_ w741] -> w737
                        frame False {
                        }
                        frame True {
                          n400 = property on="path RLC_completo" class="Path"() -> ("Value"=w757:path)  [unwired: 2 in, 2 out]
                          n401 = for {
                            N: 5 -> [_]
                            tunnel: TRUE -> [w799]
                            tunnel: FALSE -> [w798]
                            tunnel: [w797] -> w776
                            tunnel: [w796] -> w774 mode=indexing
                            tunnel: [w795] -> w773 mode=indexing
                            tunnel: [w794] -> w772 mode=indexing
                            tunnel: [w793] -> w771 mode=indexing
                            tunnel: [w792] -> w770 mode=indexing
                            tunnel: [w791] -> w769 mode=indexing
                            tunnel: [w790] -> w768 mode=indexing
                            tunnel: [w789] -> w767 mode=indexing
                            tunnel: [w788] -> w766 mode=indexing
                            tunnel: [w787] -> w765 mode=indexing
                            tunnel: [w786] -> w764 mode=indexing
                            tunnel: [w785] -> w763 mode=indexing
                            tunnel: [w784] -> w762 mode=indexing
                            tunnel: [w783] -> w761 mode=indexing
                            tunnel: [w782] -> w760 mode=indexing
                            tunnel: [w781] -> w759 mode=indexing
                            tunnel: w758 -> [w780]
                            tunnel: w757 -> [w779]
                            n402 = stacked-sequence {
                              tunnel: w799 -> [_ w847 w873 w900 w925 w952 w977 w1004 w1030 w1055 w1081 w1107 w1133 w1159 w1185 w1211 w1238 _]
                              tunnel: w798 -> [w821 _ _ _ _ _ _ _ _ _ _ _ _ _ _ _ _ w1242]
                              tunnel: [_ _ _ _ _ _ _ _ _ _ _ _ _ _ _ _ _ TRUE] -> w797
                              tunnel: [_ w827 _ _ _ _ _ _ _ _ _ _ _ _ _ _ _ _] -> w796
                              tunnel: [_ _ w853 _ _ _ _ _ _ _ _ _ _ _ _ _ _ _] -> w795
                              tunnel: [_ _ _ w879 _ _ _ _ _ _ _ _ _ _ _ _ _ _] -> w794
                              tunnel: [_ _ _ _ w905 _ _ _ _ _ _ _ _ _ _ _ _ _] -> w793
                              tunnel: [_ _ _ _ _ w931 _ _ _ _ _ _ _ _ _ _ _ _] -> w792
                              tunnel: [_ _ _ _ _ _ w957 _ _ _ _ _ _ _ _ _ _ _] -> w791
                              tunnel: [_ _ _ _ _ _ _ w983 _ _ _ _ _ _ _ _ _ _] -> w790
                              tunnel: [_ _ _ _ _ _ _ _ w1009 _ _ _ _ _ _ _ _ _] -> w789
                              tunnel: [_ _ _ _ _ _ _ _ _ w1035 _ _ _ _ _ _ _ _] -> w788
                              tunnel: [_ _ _ _ _ _ _ _ _ _ w1061 _ _ _ _ _ _ _] -> w787
                              tunnel: [_ _ _ _ _ _ _ _ _ _ _ w1087 _ _ _ _ _ _] -> w786
                              tunnel: [_ _ _ _ _ _ _ _ _ _ _ _ w1113 _ _ _ _ _] -> w785
                              tunnel: [_ _ _ _ _ _ _ _ _ _ _ _ _ w1139 _ _ _ _] -> w784
                              tunnel: [_ _ _ _ _ _ _ _ _ _ _ _ _ _ w1165 _ _ _] -> w783
                              tunnel: [_ _ _ _ _ _ _ _ _ _ _ _ _ _ _ w1191 _ _] -> w782
                              tunnel: [_ _ _ _ _ _ _ _ _ _ _ _ _ _ _ _ w1217 _] -> w781
                              tunnel: w780 -> [_ w826 w852 w878 w904 w930 w956 w982 w1008 w1034 w1060 w1086 w1112 w1138 w1164 w1190 w1216 _]
                              tunnel: w779 -> [w800 w822 w850 w876 w902 w928 w954 w980 w1006 w1032 w1058 w1084 w1110 w1136 w1162 w1188 w1214 _]
                              frame #0 {
                                w801 = "\t"
                                n403 = local write "C-50-L"(w821) -> ()
                                n404 = local write "C-50-N"(w821) -> ()
                                n405 = local write "Z-50-L"(w821) -> ()
                                n406 = local write "C-1K-N"(w821) -> ()
                                n407 = local write "C-1K-L"(w821) -> ()
                                n408 = local write "Z-50-N"(w821) -> ()
                                n409 = local write "Z-1K-N"(w821) -> ()
                                n410 = local write "Z-1K-L"(w821) -> ()
                                n411 = local write "C-10K-L"(w821) -> ()
                                n412 = local write "C-100-N"(w821) -> ()
                                n413 = local write "C-10K-N"(w821) -> ()
                                n414 = local write "Z-100-L"(w821) -> ()
                                n415 = local write "Z-10K-L"(w821) -> ()
                                n416 = local write "Z-100-N"(w821) -> ()
                                n417 = local write "Z-10K-N"(w821) -> ()
                                n418 = local write "C-100-L"(w821) -> ()
                                n419 = Open/Create/Replace File(file path (use dialog)=w800, operation (0:open)=T3."open") -> (refnum out=w815:refnum<file>, error out=w814:errorcluster)  [unwired: 2 in, 3 out]
                                n420 = Get Date/Time String(date format (0)=enum16{"short", "long", "abbreviated"}."short", want seconds? (F)=TRUE) -> (date string=w807:string, time string=w806:string)  [unwired: 1 in]
                                n421 = feedback #1() -> (w805:dbl)  [unwired: 1 in]
                                "SET 2" <- w805
                                n422 = Set File Position(refnum=w815, from (0:start)=enum16{"start", "end", "current"}."end", error in=w814) -> (refnum out=w817:refnum<file>, error out=w818:errorcluster)  [unwired: 1 in]
                                n423 = Number To Fractional String(number=w805, precision (6)=i16 2) -> (F-format string=w804:string)  [unwired: 2 in]
                                n424 = Add(x=w805, y=0.2) -> (x+y=w811:dbl)
                                n425 = feedback-in #1(w811) -> ()
                                n426 = Concatenate Strings(w804, w801, w807, w801, w806, w801) -> (w803:string)
                                n427 = Write to Text File(file (use dialog)=w817, text=w803, error in=w818) -> (refnum out=w813:refnum<file>, error out=w812:errorcluster)  [unwired: 1 in, 1 out]
                                n428 = Close File(refnum=w813, error in=w812) -> (error out=w820:errorcluster)  [unwired: 1 out]
                                n429 = call <vilib>:"Simple Error Handler.vi"("error in (no error)"=w820) -> ()  [unwired: 1 in, 8 out]
                              }
                              frame #1 {
                                w828 = "\t"
                                w846 = i16 4 ("width (-)")
                                n430 = Open/Create/Replace File(file path (use dialog)=w822, operation (0:open)=T3."open") -> (refnum out=w837:refnum<file>, error out=w836:errorcluster)  [unwired: 2 in, 3 out]
                                n431 = Multiply(x="Time RLC", y=u32 1000) -> (x*y=w825:u32)
                                n432 = Wait (ms)(milliseconds to wait=w825) -> ()  [unwired: 1 out]
                                n433 = Set File Position(refnum=w837, from (0:start)=enum16{"start", "end", "current"}."end", error in=w836) -> (refnum out=w839:refnum<file>, error out=w840:errorcluster)  [unwired: 1 in]
                                n434 = call "RLC_read.vi"("Path"=w826, "String"="cmd /c rlc_read_cAL.py") -> ("MEASURE A"=w827:dbl, "MEASURE V [V]"=w844:dbl, "concatenated string"=w848:string, "MEASURE B"=w845:dbl, "MEASURE I [A]"=w843:dbl)  [unwired: 1 out]
                                "MEASURE A" <- w827
                                "MEASURE B" <- w845
                                n435 = Number To Engineering String(2:w846, 4:w843) -> (0:w829:string)  [unwired: 2 in]
                                n436 = local write "RLC300 - digimess"(w848) -> ()
                                n437 = Number To Engineering String(2:w846, 4:w844) -> (0:w830:string)  [unwired: 2 in]
                                n438 = Number To Engineering String(2:w846, 4:w827) -> (0:w832:string)  [unwired: 2 in]
                                n439 = Number To Engineering String(2:w846, 4:w845) -> (0:w831:string)  [unwired: 2 in]
                                n440 = Concatenate Strings(w832, w828, w831, w828, w830, w828, w829, w828) -> (w833:string)
                                n441 = Write to Text File(file (use dialog)=w839, text=w833, error in=w840) -> (refnum out=w835:refnum<file>, error out=w834:errorcluster)  [unwired: 1 in, 1 out]
                                n442 = Close File(refnum=w835, error in=w834) -> (error out=w842:errorcluster)  [unwired: 1 out]
                                n443 = call <vilib>:"Simple Error Handler.vi"("error in (no error)"=w842) -> ()  [unwired: 1 in, 8 out]
                                "C-50-L" <- w847
                              }
                              frame #2 {
                                w857 = "\t"
                                w872 = i16 4 ("width (-)")
                                n444 = property on="Time RLC" class="DigNum (strict)"() -> ("Value"=w851:u32)  [unwired: 2 in, 2 out]
                                n445 = Wait (ms)(milliseconds to wait=w851) -> ()  [unwired: 1 out]
                                n446 = Open/Create/Replace File(file path (use dialog)=w850, operation (0:open)=T3."open") -> (refnum out=w866:refnum<file>, error out=w865:errorcluster)  [unwired: 2 in, 3 out]
                                n447 = Set File Position(refnum=w866, from (0:start)=enum16{"start", "end", "current"}."end", error in=w865) -> (refnum out=w868:refnum<file>, error out=w869:errorcluster)  [unwired: 1 in]
                                n448 = call "RLC_read.vi"("Path"=w852, "String"="cmd /c rlc_read_cAN.py") -> ("MEASURE A"=w853:dbl, "MEASURE V [V]"=w855:dbl, "concatenated string"=w875:string, "MEASURE B"=w856:dbl, "MEASURE I [A]"=w854:dbl)  [unwired: 1 out]
                                "MEASURE A 2" <- w853
                                "MEASURE B 2" <- w856
                                n449 = Number To Engineering String(2:w872, 4:w854) -> (0:w858:string)  [unwired: 2 in]
                                n450 = local write "RLC300 - digimess"(w875) -> ()
                                n451 = Number To Engineering String(2:w872, 4:w855) -> (0:w859:string)  [unwired: 2 in]
                                n452 = Number To Engineering String(2:w872, 4:w853) -> (0:w861:string)  [unwired: 2 in]
                                n453 = Number To Engineering String(2:w872, 4:w856) -> (0:w860:string)  [unwired: 2 in]
                                n454 = Concatenate Strings(w861, w857, w860, w857, w859, w857, w858, w857) -> (w862:string)
                                n455 = Write to Text File(file (use dialog)=w868, text=w862, error in=w869) -> (refnum out=w864:refnum<file>, error out=w863:errorcluster)  [unwired: 1 in, 1 out]
                                n456 = Close File(refnum=w864, error in=w863) -> (error out=w871:errorcluster)  [unwired: 1 out]
                                n457 = call <vilib>:"Simple Error Handler.vi"("error in (no error)"=w871) -> ()  [unwired: 1 in, 8 out]
                                "C-50-N" <- w873
                              }
                              frame #3 {
                                w883 = "\t"
                                w898 = i16 4 ("width (-)")
                                n458 = property on="Time RLC" class="DigNum (strict)"() -> ("Value"=w877:u32)  [unwired: 2 in, 2 out]
                                n459 = Wait (ms)(milliseconds to wait=w877) -> ()  [unwired: 1 out]
                                n460 = Open/Create/Replace File(file path (use dialog)=w876, operation (0:open)=T3."open") -> (refnum out=w892:refnum<file>, error out=w891:errorcluster)  [unwired: 2 in, 3 out]
                                n461 = Set File Position(refnum=w892, from (0:start)=enum16{"start", "end", "current"}."end", error in=w891) -> (refnum out=w894:refnum<file>, error out=w895:errorcluster)  [unwired: 1 in]
                                n462 = call "RLC_read.vi"("Path"=w878, "String"="cmd /c rlc_read_cBL.py") -> ("MEASURE A"=w879:dbl, "MEASURE V [V]"=w881:dbl, "concatenated string"=w901:string, "MEASURE B"=w882:dbl, "MEASURE I [A]"=w880:dbl)  [unwired: 1 out]
                                "MEASURE A 3" <- w879
                                "MEASURE B 3" <- w882
                                n463 = Number To Engineering String(2:w898, 4:w880) -> (0:w884:string)  [unwired: 2 in]
                                n464 = local write "RLC300 - digimess"(w901) -> ()
                                n465 = Number To Engineering String(2:w898, 4:w881) -> (0:w885:string)  [unwired: 2 in]
                                n466 = Number To Engineering String(2:w898, 4:w879) -> (0:w887:string)  [unwired: 2 in]
                                n467 = Number To Engineering String(2:w898, 4:w882) -> (0:w886:string)  [unwired: 2 in]
                                n468 = Concatenate Strings(w887, w883, w886, w883, w885, w883, w884, w883) -> (w888:string)
                                n469 = Write to Text File(file (use dialog)=w894, text=w888, error in=w895) -> (refnum out=w890:refnum<file>, error out=w889:errorcluster)  [unwired: 1 in, 1 out]
                                n470 = Close File(refnum=w890, error in=w889) -> (error out=w897:errorcluster)  [unwired: 1 out]
                                n471 = call <vilib>:"Simple Error Handler.vi"("error in (no error)"=w897) -> ()  [unwired: 1 in, 8 out]
                                "C-100-L" <- w900
                              }
                              frame #4 {
                                w909 = "\t"
                                w924 = i16 4 ("width (-)")
                                n472 = property on="Time RLC" class="DigNum (strict)"() -> ("Value"=w903:u32)  [unwired: 2 in, 2 out]
                                n473 = Wait (ms)(milliseconds to wait=w903) -> ()  [unwired: 1 out]
                                n474 = Open/Create/Replace File(file path (use dialog)=w902, operation (0:open)=T3."open") -> (refnum out=w918:refnum<file>, error out=w917:errorcluster)  [unwired: 2 in, 3 out]
                                n475 = Set File Position(refnum=w918, from (0:start)=enum16{"start", "end", "current"}."end", error in=w917) -> (refnum out=w920:refnum<file>, error out=w921:errorcluster)  [unwired: 1 in]
                                n476 = call "RLC_read.vi"("Path"=w904, "String"="cmd /c rlc_read_cBN.py") -> ("MEASURE A"=w905:dbl, "MEASURE V [V]"=w907:dbl, "concatenated string"=w927:string, "MEASURE B"=w908:dbl, "MEASURE I [A]"=w906:dbl)  [unwired: 1 out]
                                "MEASURE A 4" <- w905
                                "MEASURE B 4" <- w908
                                n477 = Number To Engineering String(2:w924, 4:w906) -> (0:w910:string)  [unwired: 2 in]
                                n478 = local write "RLC300 - digimess"(w927) -> ()
                                n479 = Number To Engineering String(2:w924, 4:w907) -> (0:w911:string)  [unwired: 2 in]
                                n480 = Number To Engineering String(2:w924, 4:w905) -> (0:w913:string)  [unwired: 2 in]
                                n481 = Number To Engineering String(2:w924, 4:w908) -> (0:w912:string)  [unwired: 2 in]
                                n482 = Concatenate Strings(w913, w909, w912, w909, w911, w909, w910, w909) -> (w914:string)
                                n483 = Write to Text File(file (use dialog)=w920, text=w914, error in=w921) -> (refnum out=w916:refnum<file>, error out=w915:errorcluster)  [unwired: 1 in, 1 out]
                                n484 = Close File(refnum=w916, error in=w915) -> (error out=w923:errorcluster)  [unwired: 1 out]
                                n485 = call <vilib>:"Simple Error Handler.vi"("error in (no error)"=w923) -> ()  [unwired: 1 in, 8 out]
                                "C-100-N" <- w925
                              }
                              frame #5 {
                                w950 = "\t"
                                w935 = i16 4 ("width (-)")
                                n486 = property on="Time RLC" class="DigNum (strict)"() -> ("Value"=w929:u32)  [unwired: 2 in, 2 out]
                                n487 = Wait (ms)(milliseconds to wait=w929) -> ()  [unwired: 1 out]
                                n488 = Open/Create/Replace File(file path (use dialog)=w928, operation (0:open)=T3."open") -> (refnum out=w941:refnum<file>, error out=w942:errorcluster)  [unwired: 2 in, 3 out]
                                n489 = Set File Position(refnum=w941, from (0:start)=enum16{"start", "end", "current"}."end", error in=w942) -> (refnum out=w939:refnum<file>, error out=w938:errorcluster)  [unwired: 1 in]
                                n490 = call "RLC_read.vi"("Path"=w930, "String"="cmd /c rlc_read_cCL.py") -> ("MEASURE A"=w931:dbl, "MEASURE V [V]"=w933:dbl, "concatenated string"=w953:string, "MEASURE B"=w934:dbl, "MEASURE I [A]"=w932:dbl)  [unwired: 1 out]
                                "MEASURE A 5" <- w931
                                "MEASURE B 5" <- w934
                                n491 = Number To Engineering String(2:w935, 4:w932) -> (0:w949:string)  [unwired: 2 in]
                                n492 = local write "RLC300 - digimess"(w953) -> ()
                                n493 = Number To Engineering String(2:w935, 4:w933) -> (0:w948:string)  [unwired: 2 in]
                                n494 = Number To Engineering String(2:w935, 4:w931) -> (0:w946:string)  [unwired: 2 in]
                                n495 = Number To Engineering String(2:w935, 4:w934) -> (0:w947:string)  [unwired: 2 in]
                                n496 = Concatenate Strings(w946, w950, w947, w950, w948, w950, w949, w950) -> (w945:string)
                                n497 = Write to Text File(file (use dialog)=w939, text=w945, error in=w938) -> (refnum out=w943:refnum<file>, error out=w944:errorcluster)  [unwired: 1 in, 1 out]
                                n498 = Close File(refnum=w943, error in=w944) -> (error out=w936:errorcluster)  [unwired: 1 out]
                                n499 = call <vilib>:"Simple Error Handler.vi"("error in (no error)"=w936) -> ()  [unwired: 1 in, 8 out]
                                "C-1K-L" <- w952
                              }
                              frame #6 {
                                w976 = "\t"
                                w961 = i16 4 ("width (-)")
                                n500 = property on="Time RLC" class="DigNum (strict)"() -> ("Value"=w955:u32)  [unwired: 2 in, 2 out]
                                n501 = Wait (ms)(milliseconds to wait=w955) -> ()  [unwired: 1 out]
                                n502 = Open/Create/Replace File(file path (use dialog)=w954, operation (0:open)=T3."open") -> (refnum out=w967:refnum<file>, error out=w968:errorcluster)  [unwired: 2 in, 3 out]
                                n503 = Set File Position(refnum=w967, from (0:start)=enum16{"start", "end", "current"}."end", error in=w968) -> (refnum out=w965:refnum<file>, error out=w964:errorcluster)  [unwired: 1 in]
                                n504 = call "RLC_read.vi"("Path"=w956, "String"="cmd /c rlc_read_cCN.py") -> ("MEASURE A"=w957:dbl, "MEASURE V [V]"=w959:dbl, "concatenated string"=w979:string, "MEASURE B"=w960:dbl, "MEASURE I [A]"=w958:dbl)  [unwired: 1 out]
                                "MEASURE A 6" <- w957
                                "MEASURE B 6" <- w960
                                n505 = Number To Engineering String(2:w961, 4:w958) -> (0:w975:string)  [unwired: 2 in]
                                n506 = local write "RLC300 - digimess"(w979) -> ()
                                n507 = Number To Engineering String(2:w961, 4:w959) -> (0:w974:string)  [unwired: 2 in]
                                n508 = Number To Engineering String(2:w961, 4:w957) -> (0:w972:string)  [unwired: 2 in]
                                n509 = Number To Engineering String(2:w961, 4:w960) -> (0:w973:string)  [unwired: 2 in]
                                n510 = Concatenate Strings(w972, w976, w973, w976, w974, w976, w975, w976) -> (w971:string)
                                n511 = Write to Text File(file (use dialog)=w965, text=w971, error in=w964) -> (refnum out=w969:refnum<file>, error out=w970:errorcluster)  [unwired: 1 in, 1 out]
                                n512 = Close File(refnum=w969, error in=w970) -> (error out=w962:errorcluster)  [unwired: 1 out]
                                n513 = call <vilib>:"Simple Error Handler.vi"("error in (no error)"=w962) -> ()  [unwired: 1 in, 8 out]
                                "C-1K-N" <- w977
                              }
                              frame #7 {
                                w987 = "\t"
                                w1002 = i16 4 ("width (-)")
                                n514 = property on="Time RLC" class="DigNum (strict)"() -> ("Value"=w981:u32)  [unwired: 2 in, 2 out]
                                n515 = Wait (ms)(milliseconds to wait=w981) -> ()  [unwired: 1 out]
                                n516 = Open/Create/Replace File(file path (use dialog)=w980, operation (0:open)=T3."open") -> (refnum out=w996:refnum<file>, error out=w995:errorcluster)  [unwired: 2 in, 3 out]
                                n517 = Set File Position(refnum=w996, from (0:start)=enum16{"start", "end", "current"}."end", error in=w995) -> (refnum out=w998:refnum<file>, error out=w999:errorcluster)  [unwired: 1 in]
                                n518 = call "RLC_read.vi"("Path"=w982, "String"="cmd /c rlc_read_cDL.py") -> ("MEASURE A"=w983:dbl, "MEASURE V [V]"=w985:dbl, "concatenated string"=w1005:string, "MEASURE B"=w986:dbl, "MEASURE I [A]"=w984:dbl)  [unwired: 1 out]
                                "MEASURE A 7" <- w983
                                "MEASURE B 7" <- w986
                                n519 = Number To Engineering String(2:w1002, 4:w984) -> (0:w988:string)  [unwired: 2 in]
                                n520 = local write "RLC300 - digimess"(w1005) -> ()
                                n521 = Number To Engineering String(2:w1002, 4:w985) -> (0:w989:string)  [unwired: 2 in]
                                n522 = Number To Engineering String(2:w1002, 4:w983) -> (0:w991:string)  [unwired: 2 in]
                                n523 = Number To Engineering String(2:w1002, 4:w986) -> (0:w990:string)  [unwired: 2 in]
                                n524 = Concatenate Strings(w991, w987, w990, w987, w989, w987, w988, w987) -> (w992:string)
                                n525 = Write to Text File(file (use dialog)=w998, text=w992, error in=w999) -> (refnum out=w994:refnum<file>, error out=w993:errorcluster)  [unwired: 1 in, 1 out]
                                n526 = Close File(refnum=w994, error in=w993) -> (error out=w1001:errorcluster)  [unwired: 1 out]
                                n527 = call <vilib>:"Simple Error Handler.vi"("error in (no error)"=w1001) -> ()  [unwired: 1 in, 8 out]
                                "C-10K-L" <- w1004
                              }
                              frame #8 {
                                w1013 = "\t"
                                w1028 = i16 4 ("width (-)")
                                n528 = property on="Time RLC" class="DigNum (strict)"() -> ("Value"=w1007:u32)  [unwired: 2 in, 2 out]
                                n529 = Wait (ms)(milliseconds to wait=w1007) -> ()  [unwired: 1 out]
                                n530 = Open/Create/Replace File(file path (use dialog)=w1006, operation (0:open)=T3."open") -> (refnum out=w1022:refnum<file>, error out=w1021:errorcluster)  [unwired: 2 in, 3 out]
                                n531 = Set File Position(refnum=w1022, from (0:start)=enum16{"start", "end", "current"}."end", error in=w1021) -> (refnum out=w1024:refnum<file>, error out=w1025:errorcluster)  [unwired: 1 in]
                                n532 = call "RLC_read.vi"("Path"=w1008, "String"="cmd /c rlc_read_cDN.py") -> ("MEASURE A"=w1009:dbl, "MEASURE V [V]"=w1011:dbl, "concatenated string"=w1031:string, "MEASURE B"=w1012:dbl, "MEASURE I [A]"=w1010:dbl)  [unwired: 1 out]
                                "MEASURE A 8" <- w1009
                                "MEASURE B 8" <- w1012
                                n533 = Number To Engineering String(2:w1028, 4:w1010) -> (0:w1014:string)  [unwired: 2 in]
                                n534 = local write "RLC300 - digimess"(w1031) -> ()
                                n535 = Number To Engineering String(2:w1028, 4:w1011) -> (0:w1015:string)  [unwired: 2 in]
                                n536 = Number To Engineering String(2:w1028, 4:w1009) -> (0:w1017:string)  [unwired: 2 in]
                                n537 = Number To Engineering String(2:w1028, 4:w1012) -> (0:w1016:string)  [unwired: 2 in]
                                n538 = Concatenate Strings(w1017, w1013, w1016, w1013, w1015, w1013, w1014, w1013) -> (w1018:string)
                                n539 = Write to Text File(file (use dialog)=w1024, text=w1018, error in=w1025) -> (refnum out=w1020:refnum<file>, error out=w1019:errorcluster)  [unwired: 1 in, 1 out]
                                n540 = Close File(refnum=w1020, error in=w1019) -> (error out=w1027:errorcluster)  [unwired: 1 out]
                                n541 = call <vilib>:"Simple Error Handler.vi"("error in (no error)"=w1027) -> ()  [unwired: 1 in, 8 out]
                                "C-10K-N" <- w1030
                              }
                              frame #9 {
                                w1039 = "\t"
                                w1054 = i16 4 ("width (-)")
                                n542 = property on="Time RLC" class="DigNum (strict)"() -> ("Value"=w1033:u32)  [unwired: 2 in, 2 out]
                                n543 = Wait (ms)(milliseconds to wait=w1033) -> ()  [unwired: 1 out]
                                n544 = Open/Create/Replace File(file path (use dialog)=w1032, operation (0:open)=T3."open") -> (refnum out=w1048:refnum<file>, error out=w1047:errorcluster)  [unwired: 2 in, 3 out]
                                n545 = Set File Position(refnum=w1048, from (0:start)=enum16{"start", "end", "current"}."end", error in=w1047) -> (refnum out=w1050:refnum<file>, error out=w1051:errorcluster)  [unwired: 1 in]
                                n546 = call "RLC_read.vi"("Path"=w1034, "String"="cmd /c rlc_read_ZAL.py") -> ("MEASURE A"=w1035:dbl, "MEASURE V [V]"=w1037:dbl, "concatenated string"=w1056:string, "MEASURE B"=w1038:dbl, "MEASURE I [A]"=w1036:dbl)  [unwired: 1 out]
                                "MEASURE A 9" <- w1035
                                "MEASURE B 9" <- w1038
                                n547 = Number To Engineering String(2:w1054, 4:w1036) -> (0:w1040:string)  [unwired: 2 in]
                                n548 = local write "RLC300 - digimess"(w1056) -> ()
                                n549 = Number To Engineering String(2:w1054, 4:w1037) -> (0:w1041:string)  [unwired: 2 in]
                                n550 = Number To Engineering String(2:w1054, 4:w1035) -> (0:w1043:string)  [unwired: 2 in]
                                n551 = Number To Engineering String(2:w1054, 4:w1038) -> (0:w1042:string)  [unwired: 2 in]
                                n552 = Concatenate Strings(w1043, w1039, w1042, w1039, w1041, w1039, w1040, w1039) -> (w1044:string)
                                n553 = Write to Text File(file (use dialog)=w1050, text=w1044, error in=w1051) -> (refnum out=w1046:refnum<file>, error out=w1045:errorcluster)  [unwired: 1 in, 1 out]
                                n554 = Close File(refnum=w1046, error in=w1045) -> (error out=w1053:errorcluster)  [unwired: 1 out]
                                n555 = call <vilib>:"Simple Error Handler.vi"("error in (no error)"=w1053) -> ()  [unwired: 1 in, 8 out]
                                "Z-50-L" <- w1055
                              }
                              frame #10 {
                                w1065 = "\t"
                                w1080 = i16 4 ("width (-)")
                                n556 = property on="Time RLC" class="DigNum (strict)"() -> ("Value"=w1059:u32)  [unwired: 2 in, 2 out]
                                n557 = Wait (ms)(milliseconds to wait=w1059) -> ()  [unwired: 1 out]
                                n558 = Open/Create/Replace File(file path (use dialog)=w1058, operation (0:open)=T3."open") -> (refnum out=w1074:refnum<file>, error out=w1073:errorcluster)  [unwired: 2 in, 3 out]
                                n559 = Set File Position(refnum=w1074, from (0:start)=enum16{"start", "end", "current"}."end", error in=w1073) -> (refnum out=w1076:refnum<file>, error out=w1077:errorcluster)  [unwired: 1 in]
                                n560 = call "RLC_read.vi"("Path"=w1060, "String"="cmd /c rlc_read_ZAN.py") -> ("MEASURE A"=w1061:dbl, "MEASURE V [V]"=w1063:dbl, "concatenated string"=w1082:string, "MEASURE B"=w1064:dbl, "MEASURE I [A]"=w1062:dbl)  [unwired: 1 out]
                                "MEASURE A 10" <- w1061
                                "MEASURE B 10" <- w1064
                                n561 = Number To Engineering String(2:w1080, 4:w1062) -> (0:w1066:string)  [unwired: 2 in]
                                n562 = local write "RLC300 - digimess"(w1082) -> ()
                                n563 = Number To Engineering String(2:w1080, 4:w1063) -> (0:w1067:string)  [unwired: 2 in]
                                n564 = Number To Engineering String(2:w1080, 4:w1061) -> (0:w1069:string)  [unwired: 2 in]
                                n565 = Number To Engineering String(2:w1080, 4:w1064) -> (0:w1068:string)  [unwired: 2 in]
                                n566 = Concatenate Strings(w1069, w1065, w1068, w1065, w1067, w1065, w1066, w1065) -> (w1070:string)
                                n567 = Write to Text File(file (use dialog)=w1076, text=w1070, error in=w1077) -> (refnum out=w1072:refnum<file>, error out=w1071:errorcluster)  [unwired: 1 in, 1 out]
                                n568 = Close File(refnum=w1072, error in=w1071) -> (error out=w1079:errorcluster)  [unwired: 1 out]
                                n569 = call <vilib>:"Simple Error Handler.vi"("error in (no error)"=w1079) -> ()  [unwired: 1 in, 8 out]
                                "Z-50-N" <- w1081
                              }
                              frame #11 {
                                w1091 = "\t"
                                w1106 = i16 4 ("width (-)")
                                n570 = property on="Time RLC" class="DigNum (strict)"() -> ("Value"=w1085:u32)  [unwired: 2 in, 2 out]
                                n571 = Wait (ms)(milliseconds to wait=w1085) -> ()  [unwired: 1 out]
                                n572 = Open/Create/Replace File(file path (use dialog)=w1084, operation (0:open)=T3."open") -> (refnum out=w1100:refnum<file>, error out=w1099:errorcluster)  [unwired: 2 in, 3 out]
                                n573 = Set File Position(refnum=w1100, from (0:start)=enum16{"start", "end", "current"}."end", error in=w1099) -> (refnum out=w1102:refnum<file>, error out=w1103:errorcluster)  [unwired: 1 in]
                                n574 = call "RLC_read.vi"("Path"=w1086, "String"="cmd /c rlc_read_ZBL.py") -> ("MEASURE A"=w1087:dbl, "MEASURE V [V]"=w1089:dbl, "concatenated string"=w1108:string, "MEASURE B"=w1090:dbl, "MEASURE I [A]"=w1088:dbl)  [unwired: 1 out]
                                "MEASURE A 11" <- w1087
                                "MEASURE B 11" <- w1090
                                n575 = Number To Engineering String(2:w1106, 4:w1088) -> (0:w1092:string)  [unwired: 2 in]
                                n576 = local write "RLC300 - digimess"(w1108) -> ()
                                n577 = Number To Engineering String(2:w1106, 4:w1089) -> (0:w1093:string)  [unwired: 2 in]
                                n578 = Number To Engineering String(2:w1106, 4:w1087) -> (0:w1095:string)  [unwired: 2 in]
                                n579 = Number To Engineering String(2:w1106, 4:w1090) -> (0:w1094:string)  [unwired: 2 in]
                                n580 = Concatenate Strings(w1095, w1091, w1094, w1091, w1093, w1091, w1092, w1091) -> (w1096:string)
                                n581 = Write to Text File(file (use dialog)=w1102, text=w1096, error in=w1103) -> (refnum out=w1098:refnum<file>, error out=w1097:errorcluster)  [unwired: 1 in, 1 out]
                                n582 = Close File(refnum=w1098, error in=w1097) -> (error out=w1105:errorcluster)  [unwired: 1 out]
                                n583 = call <vilib>:"Simple Error Handler.vi"("error in (no error)"=w1105) -> ()  [unwired: 1 in, 8 out]
                                "Z-100-L" <- w1107
                              }
                              frame #12 {
                                w1117 = "\t"
                                w1132 = i16 4 ("width (-)")
                                n584 = property on="Time RLC" class="DigNum (strict)"() -> ("Value"=w1111:u32)  [unwired: 2 in, 2 out]
                                n585 = Wait (ms)(milliseconds to wait=w1111) -> ()  [unwired: 1 out]
                                n586 = Open/Create/Replace File(file path (use dialog)=w1110, operation (0:open)=T3."open") -> (refnum out=w1126:refnum<file>, error out=w1125:errorcluster)  [unwired: 2 in, 3 out]
                                n587 = Set File Position(refnum=w1126, from (0:start)=enum16{"start", "end", "current"}."end", error in=w1125) -> (refnum out=w1128:refnum<file>, error out=w1129:errorcluster)  [unwired: 1 in]
                                n588 = call "RLC_read.vi"("Path"=w1112, "String"="cmd /c rlc_read_ZBN.py") -> ("MEASURE A"=w1113:dbl, "MEASURE V [V]"=w1115:dbl, "concatenated string"=w1134:string, "MEASURE B"=w1116:dbl, "MEASURE I [A]"=w1114:dbl)  [unwired: 1 out]
                                "MEASURE A 12" <- w1113
                                "MEASURE B 12" <- w1116
                                n589 = Number To Engineering String(2:w1132, 4:w1114) -> (0:w1118:string)  [unwired: 2 in]
                                n590 = local write "RLC300 - digimess"(w1134) -> ()
                                n591 = Number To Engineering String(2:w1132, 4:w1115) -> (0:w1119:string)  [unwired: 2 in]
                                n592 = Number To Engineering String(2:w1132, 4:w1113) -> (0:w1121:string)  [unwired: 2 in]
                                n593 = Number To Engineering String(2:w1132, 4:w1116) -> (0:w1120:string)  [unwired: 2 in]
                                n594 = Concatenate Strings(w1121, w1117, w1120, w1117, w1119, w1117, w1118, w1117) -> (w1122:string)
                                n595 = Write to Text File(file (use dialog)=w1128, text=w1122, error in=w1129) -> (refnum out=w1124:refnum<file>, error out=w1123:errorcluster)  [unwired: 1 in, 1 out]
                                n596 = Close File(refnum=w1124, error in=w1123) -> (error out=w1131:errorcluster)  [unwired: 1 out]
                                n597 = call <vilib>:"Simple Error Handler.vi"("error in (no error)"=w1131) -> ()  [unwired: 1 in, 8 out]
                                "Z-100-N" <- w1133
                              }
                              frame #13 {
                                w1143 = "\t"
                                w1158 = i16 4 ("width (-)")
                                n598 = property on="Time RLC" class="DigNum (strict)"() -> ("Value"=w1137:u32)  [unwired: 2 in, 2 out]
                                n599 = Wait (ms)(milliseconds to wait=w1137) -> ()  [unwired: 1 out]
                                n600 = Open/Create/Replace File(file path (use dialog)=w1136, operation (0:open)=T3."open") -> (refnum out=w1152:refnum<file>, error out=w1151:errorcluster)  [unwired: 2 in, 3 out]
                                n601 = Set File Position(refnum=w1152, from (0:start)=enum16{"start", "end", "current"}."end", error in=w1151) -> (refnum out=w1154:refnum<file>, error out=w1155:errorcluster)  [unwired: 1 in]
                                n602 = call "RLC_read.vi"("Path"=w1138, "String"="cmd /c rlc_read_ZCL.py") -> ("MEASURE A"=w1139:dbl, "MEASURE V [V]"=w1141:dbl, "concatenated string"=w1160:string, "MEASURE B"=w1142:dbl, "MEASURE I [A]"=w1140:dbl)  [unwired: 1 out]
                                "MEASURE A 13" <- w1139
                                "MEASURE B 13" <- w1142
                                n603 = Number To Engineering String(2:w1158, 4:w1140) -> (0:w1144:string)  [unwired: 2 in]
                                n604 = local write "RLC300 - digimess"(w1160) -> ()
                                n605 = Number To Engineering String(2:w1158, 4:w1141) -> (0:w1145:string)  [unwired: 2 in]
                                n606 = Number To Engineering String(2:w1158, 4:w1139) -> (0:w1147:string)  [unwired: 2 in]
                                n607 = Number To Engineering String(2:w1158, 4:w1142) -> (0:w1146:string)  [unwired: 2 in]
                                n608 = Concatenate Strings(w1147, w1143, w1146, w1143, w1145, w1143, w1144, w1143) -> (w1148:string)
                                n609 = Write to Text File(file (use dialog)=w1154, text=w1148, error in=w1155) -> (refnum out=w1150:refnum<file>, error out=w1149:errorcluster)  [unwired: 1 in, 1 out]
                                n610 = Close File(refnum=w1150, error in=w1149) -> (error out=w1157:errorcluster)  [unwired: 1 out]
                                n611 = call <vilib>:"Simple Error Handler.vi"("error in (no error)"=w1157) -> ()  [unwired: 1 in, 8 out]
                                "Z-1K-L" <- w1159
                              }
                              frame #14 {
                                w1169 = "\t"
                                w1184 = i16 4 ("width (-)")
                                n612 = property on="Time RLC" class="DigNum (strict)"() -> ("Value"=w1163:u32)  [unwired: 2 in, 2 out]
                                n613 = Wait (ms)(milliseconds to wait=w1163) -> ()  [unwired: 1 out]
                                n614 = Open/Create/Replace File(file path (use dialog)=w1162, operation (0:open)=T3."open") -> (refnum out=w1178:refnum<file>, error out=w1177:errorcluster)  [unwired: 2 in, 3 out]
                                n615 = Set File Position(refnum=w1178, from (0:start)=enum16{"start", "end", "current"}."end", error in=w1177) -> (refnum out=w1180:refnum<file>, error out=w1181:errorcluster)  [unwired: 1 in]
                                n616 = call "RLC_read.vi"("Path"=w1164, "String"="cmd /c rlc_read_ZCN.py") -> ("MEASURE A"=w1165:dbl, "MEASURE V [V]"=w1167:dbl, "concatenated string"=w1186:string, "MEASURE B"=w1168:dbl, "MEASURE I [A]"=w1166:dbl)  [unwired: 1 out]
                                "MEASURE A 14" <- w1165
                                "MEASURE B 14" <- w1168
                                n617 = Number To Engineering String(2:w1184, 4:w1166) -> (0:w1170:string)  [unwired: 2 in]
                                n618 = local write "RLC300 - digimess"(w1186) -> ()
                                n619 = Number To Engineering String(2:w1184, 4:w1167) -> (0:w1171:string)  [unwired: 2 in]
                                n620 = Number To Engineering String(2:w1184, 4:w1165) -> (0:w1173:string)  [unwired: 2 in]
                                n621 = Number To Engineering String(2:w1184, 4:w1168) -> (0:w1172:string)  [unwired: 2 in]
                                n622 = Concatenate Strings(w1173, w1169, w1172, w1169, w1171, w1169, w1170, w1169) -> (w1174:string)
                                n623 = Write to Text File(file (use dialog)=w1180, text=w1174, error in=w1181) -> (refnum out=w1176:refnum<file>, error out=w1175:errorcluster)  [unwired: 1 in, 1 out]
                                n624 = Close File(refnum=w1176, error in=w1175) -> (error out=w1183:errorcluster)  [unwired: 1 out]
                                n625 = call <vilib>:"Simple Error Handler.vi"("error in (no error)"=w1183) -> ()  [unwired: 1 in, 8 out]
                                "Z-1K-N" <- w1185
                              }
                              frame #15 {
                                w1195 = "\t"
                                w1210 = i16 4 ("width (-)")
                                n626 = property on="Time RLC" class="DigNum (strict)"() -> ("Value"=w1189:u32)  [unwired: 2 in, 2 out]
                                n627 = Wait (ms)(milliseconds to wait=w1189) -> ()  [unwired: 1 out]
                                n628 = Open/Create/Replace File(file path (use dialog)=w1188, operation (0:open)=T3."open") -> (refnum out=w1204:refnum<file>, error out=w1203:errorcluster)  [unwired: 2 in, 3 out]
                                n629 = Set File Position(refnum=w1204, from (0:start)=enum16{"start", "end", "current"}."end", error in=w1203) -> (refnum out=w1206:refnum<file>, error out=w1207:errorcluster)  [unwired: 1 in]
                                n630 = call "RLC_read.vi"("Path"=w1190, "String"="cmd /c rlc_read_ZDL.py") -> ("MEASURE A"=w1191:dbl, "MEASURE V [V]"=w1193:dbl, "concatenated string"=w1212:string, "MEASURE B"=w1194:dbl, "MEASURE I [A]"=w1192:dbl)  [unwired: 1 out]
                                "MEASURE A 15" <- w1191
                                "MEASURE B 15" <- w1194
                                n631 = Number To Engineering String(2:w1210, 4:w1192) -> (0:w1196:string)  [unwired: 2 in]
                                n632 = local write "RLC300 - digimess"(w1212) -> ()
                                n633 = Number To Engineering String(2:w1210, 4:w1193) -> (0:w1197:string)  [unwired: 2 in]
                                n634 = Number To Engineering String(2:w1210, 4:w1191) -> (0:w1199:string)  [unwired: 2 in]
                                n635 = Number To Engineering String(2:w1210, 4:w1194) -> (0:w1198:string)  [unwired: 2 in]
                                n636 = Concatenate Strings(w1199, w1195, w1198, w1195, w1197, w1195, w1196, w1195) -> (w1200:string)
                                n637 = Write to Text File(file (use dialog)=w1206, text=w1200, error in=w1207) -> (refnum out=w1202:refnum<file>, error out=w1201:errorcluster)  [unwired: 1 in, 1 out]
                                n638 = Close File(refnum=w1202, error in=w1201) -> (error out=w1209:errorcluster)  [unwired: 1 out]
                                n639 = call <vilib>:"Simple Error Handler.vi"("error in (no error)"=w1209) -> ()  [unwired: 1 in, 8 out]
                                "Z-10K-L" <- w1211
                              }
                              frame #16 {
                                w1222 = "\t"
                                w1237 = i16 4 ("width (-)")
                                n640 = property on="Time RLC" class="DigNum (strict)"() -> ("Value"=w1215:u32)  [unwired: 2 in, 2 out]
                                n641 = Wait (ms)(milliseconds to wait=w1215) -> ()  [unwired: 1 out]
                                n642 = Open/Create/Replace File(file path (use dialog)=w1214, operation (0:open)=T3."open") -> (refnum out=w1231:refnum<file>, error out=w1230:errorcluster)  [unwired: 2 in, 3 out]
                                n643 = Set File Position(refnum=w1231, from (0:start)=enum16{"start", "end", "current"}."end", error in=w1230) -> (refnum out=w1233:refnum<file>, error out=w1234:errorcluster)  [unwired: 1 in]
                                n644 = call "RLC_read.vi"("Path"=w1216, "String"="cmd /c rlc_read_ZDN.py") -> ("MEASURE A"=w1217:dbl, "MEASURE V [V]"=w1220:dbl, "concatenated string"=w1239:string, "MEASURE B"=w1221:dbl, "MEASURE I [A]"=w1219:dbl)  [unwired: 1 out]
                                "MEASURE A 16" <- w1217
                                "MEASURE B 16" <- w1221
                                n645 = Number To Engineering String(2:w1237, 4:w1219) -> (0:w1223:string)  [unwired: 2 in]
                                n646 = local write "RLC300 - digimess"(w1239) -> ()
                                n647 = Number To Engineering String(2:w1237, 4:w1220) -> (0:w1224:string)  [unwired: 2 in]
                                n648 = Number To Engineering String(2:w1237, 4:w1217) -> (0:w1226:string)  [unwired: 2 in]
                                n649 = Number To Engineering String(2:w1237, 4:w1221) -> (0:w1225:string)  [unwired: 2 in]
                                n650 = Concatenate Strings(w1226, w1222, w1225, w1222, w1224, w1222, w1223, w1222, "\r\n") -> (w1227:string)
                                n651 = Write to Text File(file (use dialog)=w1233, text=w1227, error in=w1234) -> (refnum out=w1229:refnum<file>, error out=w1228:errorcluster)  [unwired: 1 in, 1 out]
                                n652 = Close File(refnum=w1229, error in=w1228) -> (error out=w1236:errorcluster)  [unwired: 1 out]
                                n653 = call <vilib>:"Simple Error Handler.vi"("error in (no error)"=w1236) -> ()  [unwired: 1 in, 8 out]
                                "Z-10K-N" <- w1238
                              }
                              frame #17 {
                                n654 = local write "Z-50-L"(w1242) -> ()
                                n655 = local write "Z-1K-L"(w1242) -> ()
                                n656 = local write "Z-1K-N"(w1242) -> ()
                                n657 = local write "C-50-N"(w1242) -> ()
                                n658 = local write "C-50-L"(w1242) -> ()
                                n659 = local write "Z-50-N"(w1242) -> ()
                                n660 = local write "C-1K-N"(w1242) -> ()
                                n661 = local write "C-1K-L"(w1242) -> ()
                                n662 = local write "Z-100-L"(w1242) -> ()
                                n663 = local write "Z-100-N"(w1242) -> ()
                                n664 = local write "Z-10K-L"(w1242) -> ()
                                n665 = local write "Z-10K-N"(w1242) -> ()
                                n666 = local write "C-10K-N"(w1242) -> ()
                                n667 = local write "C-10K-L"(w1242) -> ()
                                n668 = local write "C-100-N"(w1242) -> ()
                                n669 = local write "C-100-L"(w1242) -> ()
                              }
                            }
                          }
                          n670 = call <vilib>:"Mean.vi"("X"=w773) -> ("mean"=w755:dbl)  [unwired: 1 out]
                          "mean 2" <- w755
                          n671 = call <vilib>:"Mean.vi"("X"=w772) -> ("mean"=w754:dbl)  [unwired: 1 out]
                          "mean 3" <- w754
                          n672 = call <vilib>:"Mean.vi"("X"=w771) -> ("mean"=w753:dbl)  [unwired: 1 out]
                          "mean 4" <- w753
                          n673 = call <vilib>:"Mean.vi"("X"=w770) -> ("mean"=w752:dbl)  [unwired: 1 out]
                          "mean 5" <- w752
                          n674 = call <vilib>:"Mean.vi"("X"=w769) -> ("mean"=w751:dbl)  [unwired: 1 out]
                          "mean 6" <- w751
                          n675 = call <vilib>:"Mean.vi"("X"=w768) -> ("mean"=w750:dbl)  [unwired: 1 out]
                          "mean 7" <- w750
                          n676 = call <vilib>:"Mean.vi"("X"=w767) -> ("mean"=w749:dbl)  [unwired: 1 out]
                          "mean 8" <- w749
                          n677 = call <vilib>:"Mean.vi"("X"=w766) -> ("mean"=w748:dbl)  [unwired: 1 out]
                          "mean 9" <- w748
                          n678 = call <vilib>:"Mean.vi"("X"=w765) -> ("mean"=w747:dbl)  [unwired: 1 out]
                          "mean 10" <- w747
                          n679 = call <vilib>:"Mean.vi"("X"=w764) -> ("mean"=w746:dbl)  [unwired: 1 out]
                          "mean 11" <- w746
                          n680 = call <vilib>:"Mean.vi"("X"=w763) -> ("mean"=w745:dbl)  [unwired: 1 out]
                          "mean 12" <- w745
                          n681 = call <vilib>:"Mean.vi"("X"=w762) -> ("mean"=w744:dbl)  [unwired: 1 out]
                          "mean 13" <- w744
                          n682 = call <vilib>:"Mean.vi"("X"=w761) -> ("mean"=w743:dbl)  [unwired: 1 out]
                          "mean 14" <- w743
                          n683 = call <vilib>:"Mean.vi"("X"=w760) -> ("mean"=w742:dbl)  [unwired: 1 out]
                          "mean 15" <- w742
                          n684 = call <vilib>:"Mean.vi"("X"=w774) -> ("mean"=w756:dbl)  [unwired: 1 out]
                          "mean" <- w756
                          n685 = call <vilib>:"Mean.vi"("X"=w759) -> ("mean"=w741:dbl)  [unwired: 1 out]
                          "mean 16" <- w741
                        }
                      }
                    }
                    frame #2 {
                      n686 = case shown="True" w1243 {
                        tunnel: w1260 -> [_ w1276]
                        tunnel: w1259 -> [_ w1275]
                        tunnel: w1258 -> [_ w1274]
                        tunnel: w1257 -> [_ w1273]
                        tunnel: w1256 -> [_ w1272]
                        tunnel: w1255 -> [_ w1271]
                        tunnel: w1254 -> [_ w1270]
                        tunnel: w1253 -> [_ w1269]
                        tunnel: w1252 -> [_ w1268]
                        tunnel: w1251 -> [_ w1267]
                        tunnel: w1250 -> [_ w1266]
                        tunnel: w1249 -> [_ w1265]
                        tunnel: w1248 -> [_ w1264]
                        tunnel: w1247 -> [_ w1263]
                        tunnel: w1246 -> [_ w1262]
                        tunnel: w1245 -> [_ w1261]
                        frame False {
                        }
                        frame True {
                          w1290 = "\t"
                          w1307 = i16 4 ("precision (6)")
                          n687 = property on="SET" class="DigNum (strict)"() -> ("Value"=w1308:i32)  [unwired: 2 in, 2 out]
                          n688 = Number To Engineering String(2:w1307, 4:w1261) -> (0:w1304:string)  [unwired: 2 in]
                          n689 = Number To Engineering String(2:w1307, 4:w1275) -> (0:w1303:string)  [unwired: 2 in]
                          n690 = Number To Engineering String(2:w1307, 4:w1274) -> (0:w1302:string)  [unwired: 2 in]
                          n691 = Number To Engineering String(2:w1307, 4:w1273) -> (0:w1301:string)  [unwired: 2 in]
                          n692 = Number To Engineering String(2:w1307, 4:w1272) -> (0:w1300:string)  [unwired: 2 in]
                          n693 = Number To Engineering String(2:w1307, 4:w1271) -> (0:w1299:string)  [unwired: 2 in]
                          n694 = Number To Engineering String(2:w1307, 4:w1270) -> (0:w1298:string)  [unwired: 2 in]
                          n695 = Number To Engineering String(2:w1307, 4:w1269) -> (0:w1297:string)  [unwired: 2 in]
                          n696 = Number To Engineering String(2:w1307, 4:w1268) -> (0:w1296:string)  [unwired: 2 in]
                          n697 = Number To Engineering String(2:w1307, 4:w1267) -> (0:w1295:string)  [unwired: 2 in]
                          n698 = Number To Engineering String(2:w1307, 4:w1266) -> (0:w1294:string)  [unwired: 2 in]
                          n699 = Number To Engineering String(2:w1307, 4:w1265) -> (0:w1293:string)  [unwired: 2 in]
                          n700 = Number To Engineering String(2:w1307, 4:w1264) -> (0:w1292:string)  [unwired: 2 in]
                          n701 = Number To Engineering String(2:w1307, 4:w1263) -> (0:w1291:string)  [unwired: 2 in]
                          n702 = Number To Engineering String(2:w1307, 4:w1276) -> (0:w1305:string)  [unwired: 2 in]
                          n703 = Number To Engineering String(2:w1307, 4:w1262) -> (0:w1289:string)  [unwired: 2 in]
                          n704 = Number To Decimal String(number=w1308) -> (decimal integer string=w1306:string)  [unwired: 1 in]
                          n705 = property on="path RLC_mean" class="Path"() -> ("Value"=w1277:path)  [unwired: 2 in, 2 out]
                          n706 = Open/Create/Replace File(file path (use dialog)=w1277, operation (0:open)=T3."open") -> (refnum out=w1282:refnum<file>, error out=w1281:errorcluster)  [unwired: 2 in, 3 out]
                          n707 = Concatenate Strings(w1306, w1290, w1305, w1290, w1304, w1290, w1303, w1290, w1302, w1290, w1301, w1290, w1300, w1290, w1299, w1290, w1298, w1290, w1297, w1290, w1296, w1290, w1295, w1290, w1294, w1290, w1293, w1290, w1292, w1290, w1291, w1290, w1289, "\r\n") -> (w1278:string)
                          n708 = Set File Position(refnum=w1282, from (0:start)=enum16{"start", "end", "current"}."end", error in=w1281) -> (refnum out=w1284:refnum<file>, error out=w1285:errorcluster)  [unwired: 1 in]
                          n709 = Write to Text File(file (use dialog)=w1284, text=w1278, error in=w1285) -> (refnum out=w1280:refnum<file>, error out=w1279:errorcluster)  [unwired: 1 in, 1 out]
                          n710 = Close File(refnum=w1280, error in=w1279) -> (error out=w1287:errorcluster)  [unwired: 1 out]
                          n711 = call <vilib>:"Simple Error Handler.vi"("error in (no error)"=w1287) -> ()  [unwired: 1 in, 8 out]
                        }
                      }
                    }
                  }
                  n712 = local write "graph RLC"(w692) -> ()
                }
                frame 9 {
                  n713 = flat-sequence {
                    tunnel: w1347 -> [w1358]
                    tunnel: [w1358] -> w1346
                    tunnel: [w1352] -> w1345
                    tunnel: [w1351] -> w1344
                    tunnel: w1346 -> [w1383]
                    tunnel: w1345 -> [_]
                    tunnel: w1344 -> [w1380]
                    frame #0 {
                      n714 = property on="SET" class="DigNum (strict)"() -> ("Value"=w1356:i32)  [unwired: 2 in, 2 out]
                      n715 = Increment(x=w1356) -> (x+1=w1351:i32)
                      n716 = property on="P_max camara" class="DigNum (strict)"() -> ("Value"=w1349:dbl)  [unwired: 2 in, 2 out]
                      n717 = local write "SET"(w1351) -> ()
                      n718 = property on="Camara 2" class="Slide (strict)"() -> ("Value"=w1350:dbl)  [unwired: 2 in, 2 out]
                      n719 = case shown="False" "Boolean" {
                        selector: "Boolean" -> [w1364 w1369]
                        tunnel: [w1366 w1373] -> w1353
                        tunnel: w1351 -> [w1367 _]
                        frame False {
                          n720 = local write "Boolean 2"(w1364) -> ()
                          n721 = Index Array(array="Array", index=w1367) -> (element=w1366:dbl)
                          n722 = Not(x=w1364) -> (.not. x?=→"Boolean 3":bool)
                        }
                        frame True {
                          n723 = property on="Set P auto" class="DigNum (strict)"() -> ("Value"=w1371:dbl)  [unwired: 2 in, 2 out]
                          n724 = Add(x="Step P", y=w1371) -> (x+y=w1373:dbl)
                          n725 = Not(x=w1369) -> (.not. x?=w1370:bool)
                          n726 = local write "Boolean 3"(w1370) -> ()
                          "Boolean 2" <- w1369
                        }
                      }
                      n727 = Greater?(x=w1350, y=w1349) -> (0:w1348:bool)
                      n728 = case shown="True" w1348 {
                        frame False {
                        }
                        frame True {
                          n729 = property on="Desc SET" class="DigNum (strict)"() -> ("Value"=w1360:i32)  [unwired: 2 in, 2 out]
                          n730 = local write "Descarga"(TRUE ("Descarga")) -> ()
                          n731 = Increment(x=w1360) -> (x+1=w1359:i32)
                          n732 = local write "Desc SET"(w1359) -> ()
                        }
                      }
                      n733 = Greater?(x=w1353, y="P_max") -> (0:w1355:bool)
                      n734 = case shown="True" w1355 {
                        tunnel: [w1362 w1363] -> w1352
                        tunnel: "P_max" -> [_ w1363]
                        tunnel: w1353 -> [w1362 _]
                        frame False {
                        }
                        frame True {
                        }
                      }
                      n735 = local write "Set P auto"(w1352) -> ()
                    }
                    frame #1 {
                      n736 = property on="Desc SET" class="DigNum (strict)"() -> ("Value"=w1375:i32)  [unwired: 2 in, 2 out]
                      n737 = Quotient & Remainder(x=w1380, y="Step ZPit") -> (x-y*floor(x/y)=w1381:dbl)  [unwired: 1 out]
                      n738 = Greater Than 0?(x=w1375) -> (x > 0?=w1377:bool)
                      n739 = Equal To 0?(x=w1381) -> (x = 0?=w1379:bool)
                      "Read ZPit" <- w1379
                      n740 = property on="Descarga" class="Bool (strict)"() -> ("Value"=w1374:bool)  [unwired: 2 in, 2 out]
                      n741 = And(x=w1377, y=w1374) -> (x .and. y?=w1376:bool)
                      n742 = case shown="True" w1376 {
                        tunnel: w1379 -> [w1384 _]
                        tunnel: [w1384 w1385] -> w1378
                        frame False {
                        }
                        frame True {
                          w1385 = TRUE
                          n743 = local write "Read ZPit"(w1385) -> ()
                        }
                      }
                      n744 = case shown="True" w1378 {
                        tunnel: w1383 -> [_ w1387]
                        frame False {
                          n745 = local write "Estagio auto"(11 ("Estagio auto")) -> ()
                        }
                        frame True {
                          n746 = Greater?(x=w1387, y=1.0) -> (0:w1392:bool)
                          n747 = case shown="True" w1392 {
                            tunnel: [FALSE ("Boolean") TRUE ("Boolean")] -> w1390
                            frame False {
                              w1412 = TRUE ("Boolean")
                              n748 = local write "Vácuo 2"(w1412) -> ()
                              n749 = Multiply(x="ZPf2 time", y=0.0741) -> (x*y=w1407:dbl)
                              n750 = local write "String"("Limpar volume referencia" ("String")) -> ()
                              n751 = Add(x=w1407, y=1.9801) -> (x+y=w1405:dbl)
                              n752 = call "Controle_vacuo.vi"("time (s) to wait vacuo"=w1405, "Boolean"=w1412) -> ("Vacuo"=w1413:bool)  [unwired: 9 in]
                              n753 = local write "Vácuo 2"(w1413) -> ()
                            }
                            frame True {
                              n754 = property on="ATM wait" class="DigNum (strict)"() -> ("Value"=w1414:u32)  [unwired: 2 in, 2 out]
                              n755 = call "Controle_ATM.vi"("seconds to wait"=w1414) -> ("String 2"=w1417:string, "Atm"=w1416:bool)  [unwired: 9 in]
                              n756 = local write "Atm 2"(w1416) -> ()
                              n757 = local write "String"(w1417) -> ()
                            }
                          }
                          n758 = for {
                            N: 1 -> [_]
                            tunnel: [w1394] -> w1389
                            tunnel: w1390 -> [w1394]
                            n759 = Wait (ms)(milliseconds to wait=u32 500 ("x")) -> ()  [unwired: 1 out]
                          }
                          n760 = case shown="True" w1389 {
                            frame False {
                              n761 = local write "Estagio auto"(10 ("Estagio auto")) -> ()
                            }
                            frame True {
                              w1403 = TRUE ("Boolean")
                              n762 = property on="ZPf2 time" class="DigNum (strict)"() -> ("Value"=w1397:dbl)  [unwired: 2 in, 2 out]
                              n763 = local write "Estagio auto"(10 ("Estagio auto")) -> ()
                              n764 = Multiply(x=w1397, y=0.0741) -> (x*y=w1399:dbl)
                              n765 = local write "Vácuo 2"(w1403) -> ()
                              n766 = local write "String"("Limpar volume referencia" ("String")) -> ()
                              n767 = Add(x=w1399, y=1.9801) -> (x+y=w1396:dbl)
                              n768 = call "Controle_vacuo.vi"("time (s) to wait vacuo"=w1396, "Boolean"=w1403) -> ("Vacuo"=w1404:bool)  [unwired: 9 in]
                              n769 = local write "Vácuo 2"(w1404) -> ()
                            }
                          }
                        }
                      }
                    }
                  }
                }
                frame 10 {
                  n770 = property on="Contador" class="DigNum (strict)"() -> ("Value"=w1419:i32)  [unwired: 2 in, 2 out]
                  n771 = Increment(x=w1419) -> (x+1=w1421:i32)
                  n772 = property on="N fit 2" class="DigNum (strict)"() -> ("Value"=w1418:i32)  [unwired: 2 in, 2 out]
                  n773 = local write "String"("Ler ZPf2 e T" ("String")) -> ()
                  n774 = Equal?(x=w1421, y=w1418) -> (x = y?=w1420:bool)
                  n775 = case shown="True" w1420 {
                    frame False {
                    }
                    frame True {
                      n776 = local write "Estagio auto"(11 ("Estagio auto")) -> ()
                    }
                  }
                }
                frame 11 {
                  n777 = property on="Contador" class="DigNum (strict)"() -> ("Value"=w1427:i32)  [unwired: 2 in, 2 out]
                  n778 = Increment(x=w1427) -> (x+1=w1428:i32)
                  n779 = property on="N fit 2" class="DigNum (strict)"() -> ("Value"=w1424:i32)  [unwired: 2 in, 2 out]
                  n780 = Equal?(x=w1428, y=w1424) -> (x = y?=w1426:bool)
                  n781 = case shown="True" w1426 {
                    tunnel: w1429 -> [_ w1440]
                    tunnel: w1425 -> [_ w1430]
                    frame False {
                    }
                    frame True {
                      w1431 = i16 3 ("precision (6)")
                      w1434 = "\t"
                      n782 = property on="Read ZPit" class="Bool (strict)"() -> ("Value"=w1435:bool)  [unwired: 2 in, 2 out]
                      n783 = property on="T fit" class="DigNum (strict)"() -> ("Value"=w1436:dbl)  [unwired: 2 in, 2 out]
                      n784 = case shown="False" w1435 {
                        tunnel: ["  ==>" w1446] -> w1439
                        tunnel: w1431 -> [_ w1445]
                        frame False {
                        }
                        frame True {
                          n785 = property on="P fit" class="DigNum (strict)"() -> ("Value"=w1444:dbl)  [unwired: 2 in, 2 out]
                          n786 = Number To Fractional String(number=w1444, precision (6)=w1445) -> (F-format string=w1446:string)  [unwired: 2 in]
                        }
                      }
                      n787 = Number To Fractional String(number=w1436, precision (6)=w1431) -> (F-format string=w1438:string)  [unwired: 2 in]
                      n788 = Number To Fractional String(number=w1430, precision (6)=w1431) -> (F-format string=w1433:string)  [unwired: 2 in]
                      n789 = Concatenate Strings(w1439, w1434, w1438, w1434, w1433, "\r\n") -> (w1437:string)
                      n790 = flat-sequence {
                        tunnel: [w1450] -> w1442
                        tunnel: [w1449] -> w1441
                        tunnel: w1437 -> [w1448]
                        tunnel: w1440 -> [w1447]
                        tunnel: w1442 -> [w1464]
                        tunnel: w1441 -> [w1463]
                        frame #0 {
                          n791 = Open/Create/Replace File(file path (use dialog)=w1447, operation (0:open)=T3."open") -> (refnum out=w1456:refnum<file>, error out=w1457:errorcluster)  [unwired: 2 in, 3 out]
                          n792 = Set File Position(refnum=w1456, from (0:start)=enum16{"start", "end", "current"}."end", error in=w1457) -> (refnum out=w1454:refnum<file>, error out=w1453:errorcluster)  [unwired: 1 in]
                          n793 = Write to Text File(file (use dialog)=w1454, text=w1448, error in=w1453) -> (refnum out=w1458:refnum<file>, error out=w1459:errorcluster)  [unwired: 2 out]
                          n794 = Close File(refnum=w1458, error in=w1459) -> (path=w1450:path, error out=w1451:errorcluster)
                          n795 = call <vilib>:"Simple Error Handler.vi"("error in (no error)"=w1451) -> ("error out"=w1449:errorcluster)  [unwired: 1 in, 7 out]
                        }
                        frame #1 {
                          w1460 = TRUE ("ZPit")
                          n796 = Wait (ms)(milliseconds to wait=u32 500) -> ()  [unwired: 1 out]
                          n797 = local write "T 2"(w1460) -> ()
                          n798 = local write "ZPf2 2"(w1460) -> ()
                          n799 = Read from Text File(file (use dialog)=w1464, count=-1 ("Count  3"), error in=w1463) -> (refnum out=w1465:refnum<file>, text=w1469:string, error out=w1466:errorcluster)  [unwired: 1 in, 1 out]
                          n800 = local write "String 3"(w1469) -> ()
                          n801 = Close File(refnum=w1465, error in=w1466) -> (error out=w1467:errorcluster)  [unwired: 1 out]
                          n802 = local write "String"("abrir valvula entrada gas" ("String")) -> ()
                          n803 = call <vilib>:"Simple Error Handler.vi"("error in (no error)"=w1467) -> ()  [unwired: 1 in, 8 out]
                        }
                        frame #2 {
                          n804 = property on="Desc SET" class="DigNum (strict)"() -> ("Value"=w1471:i32)  [unwired: 2 in, 2 out]
                          n805 = Greater Than 0?(x=w1471) -> (x > 0?=w1470:bool)
                          n806 = property on="Camara 2" class="Slide (strict)"() -> ("Value"=w1478:dbl)  [unwired: 2 in, 2 out]
                          n807 = Greater?(x=w1478, y="P_max camara") -> (0:w1476:bool)
                          n808 = property on="Carga" class="Bool (strict)"() -> ("Value"=w1475:bool)  [unwired: 2 in, 2 out]
                          n809 = And(x=w1476, y=w1475) -> (x .and. y?=w1473:bool)
                          n810 = case shown="False" w1470 {
                            tunnel: w1473 -> [w1479 _]
                            tunnel: [w1479 TRUE] -> w1472
                            frame False {
                            }
                            frame True {
                            }
                          }
                          n811 = case shown="True" w1472 {
                            tunnel: [5 ("N fit") w1485] -> w1474
                            frame False {
                              n812 = local write "Estagio auto"(0 ("Estagio auto")) -> ()
                              "Carga" <- TRUE
                              "Descarga" <- FALSE
                            }
                            frame True {
                              n813 = local write "teste slope"(0 ("teste slope")) -> ()
                              n814 = local write "Carga"(FALSE ("Carga")) -> ()
                              n815 = local write "Descarga"(TRUE ("Descarga")) -> ()
                              n816 = local write "Estagio auto"(12 ("Estagio auto")) -> ()
                              n817 = property on="N fit 2" class="DigNum (strict)"() -> ("Value"=w1485:i32)  [unwired: 2 in, 2 out]
                            }
                          }
                          n818 = local write "N fit"(w1474) -> ()
                        }
                      }
                    }
                  }
                }
                frame 12 {
                  w1495 = "\t"
                  n819 = property on="SET" class="DigNum (strict)"() -> ("Value"=w1499:i32)  [unwired: 2 in, 2 out]
                  n820 = Number To Decimal String(number=w1499) -> (decimal integer string=w1502:string)  [unwired: 1 in]
                  n821 = Number To Fractional String(number=0.0, precision (6)=i16 3) -> (F-format string=w1496:string)  [unwired: 2 in]
                  n822 = Concatenate Strings(w1502, w1495, w1496, w1495, w1496, w1495) -> (w1501:string)
                  n823 = flat-sequence {
                    tunnel: w1498 -> [w1507]
                    tunnel: w1501 -> [w1508]
                    tunnel: [w1508] -> w1494
                    tunnel: [w1507] -> w1493
                    tunnel: [w1512] -> w1504
                    tunnel: [w1511] -> w1503
                    tunnel: w1494 -> [w1510]
                    tunnel: w1493 -> [w1509]
                    tunnel: [w1509] -> w1492
                    tunnel: w1504 -> [w1528]
                    tunnel: w1503 -> [w1527]
                    tunnel: w1492 -> [w1522]
                    tunnel: [w1522] -> w1491
                    tunnel: w1491 -> [w1536]
                    tunnel: [w1535] -> w1490
                    tunnel: w1490 -> [w1573]
                    frame #0 {
                      w1506 = FALSE ("ZPit 2")
                      n824 = Wait (ms)(milliseconds to wait=u32 1000) -> ()  [unwired: 1 out]
                      n825 = local write "ZPit 2"(w1506) -> ()
                      n826 = local write "Pit 2"(w1506) -> ()
                      n827 = local write "Pf2 2"(w1506) -> ()
                      n828 = local write "ZPf2 2"(w1506) -> ()
                      n829 = local write "T 2"(w1506) -> ()
                    }
                    frame #1 {
                      n830 = Open/Create/Replace File(file path (use dialog)=w1509, operation (0:open)=T3."open") -> (refnum out=w1518:refnum<file>, error out=w1519:errorcluster)  [unwired: 2 in, 3 out]
                      n831 = Set File Position(refnum=w1518, from (0:start)=enum16{"start", "end", "current"}."end", error in=w1519) -> (refnum out=w1516:refnum<file>, error out=w1515:errorcluster)  [unwired: 1 in]
                      n832 = Write to Text File(file (use dialog)=w1516, text=w1510, error in=w1515) -> (refnum out=w1520:refnum<file>, error out=w1521:errorcluster)  [unwired: 2 out]
                      n833 = Close File(refnum=w1520, error in=w1521) -> (path=w1512:path, error out=w1513:errorcluster)
                      n834 = call <vilib>:"Simple Error Handler.vi"("error in (no error)"=w1513) -> ("error out"=w1511:errorcluster)  [unwired: 1 in, 7 out]
                    }
                    frame #2 {
                      w1523 = TRUE ("ZPit")
                      n835 = local write "Estagio auto"(7 ("Estagio auto")) -> ()
                      n836 = Wait (ms)(milliseconds to wait=u32 500) -> ()  [unwired: 1 out]
                      n837 = local write "ZPit 2"(w1523) -> ()
                      n838 = local write "Pit 2"(w1523) -> ()
                      n839 = Read from Text File(file (use dialog)=w1528, count=-1 ("Count  3"), error in=w1527) -> (refnum out=w1529:refnum<file>, text=w1533:string, error out=w1530:errorcluster)  [unwired: 1 in, 1 out]
                      n840 = local write "String 3"(w1533) -> ()
                      n841 = Close File(refnum=w1529, error in=w1530) -> (error out=w1531:errorcluster)  [unwired: 1 out]
                      n842 = call <vilib>:"Simple Error Handler.vi"("error in (no error)"=w1531) -> ()  [unwired: 1 in, 8 out]
                      n843 = local write "String"("abrir valvula camara" ("String")) -> ()
                    }
                    frame #3 {
                      n844 = property on="Camara 2" class="Slide (strict)"() -> ("Value"=w1539:dbl)  [unwired: 2 in, 2 out]
                      n845 = Less?(x=w1539, y="P_min descarga") -> (x < y?=w1534:bool)
                      n846 = property on="Efetuados" class="DigNum (strict)"() -> ("Value"=w1537:dbl)  [unwired: 2 in, 2 out]
                      n847 = case shown="True" w1534 {
                        tunnel: w1537 -> [_ w1568]
                        tunnel: w1536 -> [_ w1557]
                        tunnel: [TRUE ("data") FALSE ("data")] -> w1535
                        tunnel: w1534 -> [_ w1546]
                        frame False {
                          n848 = property on="Desc SET" class="DigNum (strict)"() -> ("Value"=w1541:i32)  [unwired: 2 in, 2 out]
                          n849 = Increment(x=w1541) -> (x+1=→"Desc SET":i32)
                        }
                        frame True {
                          w1555 = "\r\n"
                          n850 = Increment(x=w1568) -> (x+1=w1543:dbl)
                          "Efetuados" <- w1543
                          n851 = local write "Estagio auto"(0 ("Estagio auto")) -> ()
                          n852 = local write "SET"(0 ("SET")) -> ()
                          n853 = local write "Desc SET"(0 ("Desc SET")) -> ()
                          n854 = local write "Descarga"(FALSE ("Descarga")) -> ()
                          n855 = local write "Carga"(TRUE ("Carga")) -> ()
                          n856 = local write "Set P auto"(0.5 ("Set P auto")) -> ()
                          n857 = Open/Create/Replace File(file path (use dialog)=w1557, operation (0:open)=T3."open") -> (refnum out=w1563:refnum<file>, error out=w1564:errorcluster)  [unwired: 2 in, 3 out]
                          n858 = Less Or Equal?(x="Ciclos", y=w1543) -> (x <= y?=w1544:bool)
                          n859 = And(x=w1546, y=w1544) -> (x .and. y?=w1547:bool)
                          n860 = Set File Position(refnum=w1563, from (0:start)=enum16{"start", "end", "current"}."end", error in=w1564) -> (refnum out=w1561:refnum<file>, error out=w1560:errorcluster)  [unwired: 1 in]
                          n861 = case shown="False" w1547 {
                            frame False {
                              n862 = local write "FIM"(FALSE ("FIM")) -> ()
                            }
                            frame True {
                              w1572 = 1 ("N fit")
                              n863 = local write "Auto Ctrl"(FALSE ("Auto Ctrl")) -> ()
                              n864 = local write "N fit"(w1572) -> ()
                              n865 = local write "N to fit"(w1572) -> ()
                              "FIM" <- TRUE ("stop")
                            }
                          }
                          n866 = Concatenate Strings(w1555, ">>>>>>>>>>>>>>" ("string"), w1555, w1555) -> (w1554:string)
                          n867 = Write to Text File(file (use dialog)=w1561, text=w1554, error in=w1560) -> (refnum out=w1565:refnum<file>, error out=w1566:errorcluster)  [unwired: 2 out]
                          n868 = Close File(refnum=w1565, error in=w1566) -> (error out=w1558:errorcluster)  [unwired: 1 out]
                          n869 = call <vilib>:"Simple Error Handler.vi"("error in (no error)"=w1558) -> ()  [unwired: 1 in, 8 out]
                        }
                      }
                    }
                    frame #4 {
                      w1575 = T7 3 items=["no dialog", "OK message", "continue or stop message", "OK message + warnings", "continue/stop + warnings"] ("type of dialog (OK msg:1)")
                      n870 = local write "Câmara 2"(w1573) -> ()
                      n871 = call-poly <vilib>:"DAQmx Create Virtual Channel.vi"("lines"=tag "Dev1/port0/line3") -> ("task out"=w1584:refnum<k21>, "error out"=w1583:errorcluster)  [unwired: 13 in]
                      n872 = call <vilib>:"DAQmx Start Task.vi"("task/channels in"=w1584, "error in"=w1583) -> ("task out"=w1582:refnum<k21>, "error out"=w1581:errorcluster)  [unwired: 12 in]
                      n873 = call-poly <vilib>:"DAQmx Write.vi"("task/channels in"=w1582, "data"=w1573, "error in"=w1581) -> ("task out"=w1577:refnum<k21>, "error out"=w1576:errorcluster)  [unwired: 10 in, 1 out]
                      n874 = call <vilib>:"DAQmx Stop Task.vi"("task/channels in"=w1577, "error in"=w1576) -> ("task out"=w1579:refnum<k21>, "error out"=w1580:errorcluster)  [unwired: 12 in]
                      n875 = call <vilib>:"DAQmx Clear Task.vi"("task in"=w1579, "error in"=w1580) -> ("error out"=w1574:errorcluster)  [unwired: 13 in]
                      n876 = call <vilib>:"Simple Error Handler.vi"("type of dialog (OK msg:1)"=w1575, "error in (no error)"=w1574) -> ()  [unwired: 3 in, 5 out]
                    }
                  }
                }
              }
            }
          }
          n877 = Index Array(array=w264, index=w262) -> (element=w261:dbl)
          n878 = Index Array(array=w263, index=w262) -> (element=w260:dbl)
          n879 = Bundle("Real 2D Array"=w267, "Best Linear Fit"=w279) -> (w278:T8)  [unwired: 1 in]
          n880 = Bundle("Real 2D Array"=w267, "Best Polynomial Fit"=w268) -> (w265:T9)  [unwired: 1 in]
          n881 = Bundle("Real 2D Array"=w267, "Best Polynomial Fit"=w269) -> (w266:T9)  [unwired: 1 in]
          n882 = case shown="True" w259 {
            tunnel: w261 -> [_ w1587]
            tunnel: w260 -> [_ w1586]
            tunnel: w254 -> [_ w1585]
            frame False {
            }
            frame True {
              "P fit" <- w1587
              "T fit" <- w1586
              "P (bar/s)" <- w1585
            }
          }
          n883 = Build Array(w277, w278, w265) -> (→"Linear T":T10)
          n884 = Bundle("Real 2D Array"=w267, "Best Linear Fit"=w274) -> (w275:T8)  [unwired: 1 in]
          n885 = Build Array(w276, w275, w266) -> (→"Linear P":T10)
          "Contador" <- w258
        }
        n886 = local write "P subarray 2"(dbl[] [0.0, 1.0] ("subarray")) -> ()
        n887 = local write "T subarray 3"(dbl[] [0.0, 1.0] ("subarray")) -> ()
        n888 = local write "time subarray"(dbl[] [0.0, 1.0] ("subarray")) -> ()
      }
    }
    n889 = case shown="False" "Auto Ctrl" {
      tunnel: [TRUE ("Auto Ctrl") FALSE ("Auto Ctrl")] -> w49
      frame False {
      }
      frame True {
      }
    }
    n890 = Exclusive Or(1:w46, 2:"stop") -> (0:w48:bool)
    n891 = case shown="True" "Ligar RLC" {
      tunnel: w43 -> [_ w168]
      frame False {
      }
      frame True {
        w176 = "\t"
        w197 = "\t"
        w180 = "\r"
        w173 = "\r\n"
        w213 = "\r"
        w203 = "\t"
        n892 = Strip Path(path=w168) -> (stripped path=w169:path, name=w172:string)
        n893 = Get Date/Time String(date format (0)=enum16{"short", "long", "abbreviated"}."short", want seconds? (F)=TRUE) -> (date string=w220:string, time string=w219:string)  [unwired: 1 in]
        n894 = Concatenate Strings("SET" ("Nota 4"), w176, "DATE" ("Nota 4"), w176, "TIME" ("Nota 4"), w176, w197, "P (BAR)" ("Nota 4"), w197, "T (ºC)" ("Nota 4"), w197, "C-50-L" ("Nota 4"), w197, "C-50-N" ("Nota 4"), w197, "C-100-L" ("Nota 4"), w197, "C-100-N" ("Nota 4"), w197, "C-1K-L" ("Nota 4"), w197, "C-1K-N" ("Nota 4"), w197, "C-10K-L" ("Nota 4"), w197, "C-10K-N" ("Nota 4"), w197, "Z-50-L" ("Nota 4"), w197, "Z-50-N" ("Nota 4"), w197, "Z-100-L" ("Nota 4"), w197, "Z-100-N" ("Nota 4"), w197, "Z-1K-L" ("Nota 4"), w197, "Z-1K-N" ("Nota 4"), w197, "Z-10K-L" ("Nota 4"), w197, "Z-10K-N" ("Nota 4")) -> (w181:string)
        n895 = Concatenate Strings(w220, w203, w219) -> (w215:string)
        n896 = Concatenate Strings(w172, "_RLC_CDH completo" ("string")) -> (w170:string)
        n897 = Concatenate Strings("Sievert RLC - CDH:" ("string"), w203, w173, w173) -> (w201:string)
        n898 = Concatenate Strings("Data Table" ("string"), w180, "==========" ("string"), w180, w181, w180) -> (w214:string)
        n899 = File Dialog(6:".txt" ("pattern label"), 9:w170, 11:w169) -> (0:w211:errorcluster, 3:w212:path)  [unwired: 2 in, 4 out]
        n900 = Open/Create/Replace File(file path (use dialog)=w212, error in=w211, operation (0:open)=T3."replace or create with confirmation", access (0:read/write)=enum16{"read/write", "read-only", "write-only"}."read/write") -> (refnum out=w208:refnum<file>, error out=w207:errorcluster)  [unwired: 3 out]
        n901 = Concatenate Strings(w215, w213, w213, w201, w213, w213, "Nota 01: MEDIDAS COM RLC 300 - MULTILEITURA" ("Nota 4"), w213, w213, w214) -> (w218:string)
        n902 = Write to Text File(file (use dialog)=w208, text=w218, error in=w207) -> (refnum out=w206:refnum<file>, error out=w204:errorcluster)  [unwired: 1 in, 1 out]
        n903 = Close File(refnum=w206, error in=w204) -> (path=w200:path)  [unwired: 1 out]
        n904 = local write "path RLC_completo"(w200) -> ()
      }
    }
    n905 = case shown="True" "Ligar RLC" {
      tunnel: w43 -> [_ w111]
      frame False {
      }
      frame True {
        w120 = "\t"
        w141 = "\t"
        w124 = "\r"
        w117 = "\r\n"
        w156 = "\r"
        w146 = "\t"
        n906 = Strip Path(path=w111) -> (stripped path=w113:path, name=w116:string)
        n907 = Get Date/Time String(date format (0)=enum16{"short", "long", "abbreviated"}."short", want seconds? (F)=TRUE) -> (date string=w163:string, time string=w162:string)  [unwired: 1 in]
        n908 = Concatenate Strings("SET" ("Nota 4"), w120, "DATE" ("Nota 4"), w120, "TIME" ("Nota 4"), w120, w141, "P (BAR)" ("Nota 4"), w141, "T (ºC)" ("Nota 4"), w141, "C-50-L" ("Nota 4"), w141, "C-50-N" ("Nota 4"), w141, "C-100-L" ("Nota 4"), w141, "C-100-N" ("Nota 4"), w141, "C-1K-L" ("Nota 4"), w141, "C-1K-N" ("Nota 4"), w141, "C-10K-L" ("Nota 4"), w141, "C-10K-N" ("Nota 4"), w141, "Z-50-L" ("Nota 4"), w141, "Z-50-N" ("Nota 4"), w141, "Z-100-L" ("Nota 4"), w141, "Z-100-N" ("Nota 4"), w141, "Z-1K-L" ("Nota 4"), w141, "Z-1K-N" ("Nota 4"), w141, "Z-10K-L" ("Nota 4"), w141, "Z-10K-N" ("Nota 4")) -> (w125:string)
        n909 = Concatenate Strings(w163, w146, w162) -> (w158:string)
        n910 = Concatenate Strings(w116, "_RLC_CDH mean" ("string")) -> (w114:string)
        n911 = Concatenate Strings("Sievert RLC - CDH:" ("string"), w146, w117, w117) -> (w144:string)
        n912 = Concatenate Strings("Data Table" ("string"), w124, "==========" ("string"), w124, w125, w124) -> (w157:string)
        n913 = File Dialog(6:".txt" ("pattern label"), 9:w114, 11:w113) -> (0:w154:errorcluster, 3:w155:path)  [unwired: 2 in, 4 out]
        n914 = Open/Create/Replace File(file path (use dialog)=w155, error in=w154, operation (0:open)=T3."replace or create with confirmation", access (0:read/write)=enum16{"read/write", "read-only", "write-only"}."read/write") -> (refnum out=w151:refnum<file>, error out=w150:errorcluster)  [unwired: 3 out]
        n915 = Concatenate Strings(w158, w156, w156, w144, w156, w156, "Nota 01: MEDIDAS COM RLC 300 - MULTILEITURA" ("Nota 4"), w156, w156, w157) -> (w161:string)
        n916 = Write to Text File(file (use dialog)=w151, text=w161, error in=w150) -> (refnum out=w149:refnum<file>, error out=w147:errorcluster)  [unwired: 1 in, 1 out]
        n917 = Close File(refnum=w149, error in=w147) -> (path=w112:path)  [unwired: 1 out]
        n918 = local write "path RLC_mean"(w112) -> ()
      }
    }
    n919 = case shown="True" "RLC on/off" {
      tunnel: w36 -> [_ w54]
      frame False {
      }
      frame True {
        n920 = call "RLC READ DINAMICO.vi"("Boolean"="graph RLC", "Path"=w54, "String"="Combo Box") -> ("MEASURE R [Ohm ]"=w58:dbl, "MEASURE C [F ]"=w57:dbl)  [unwired: 7 in]
        "MEASURE C [F ]" <- w57
        n921 = Merge Signals(w57, w58) -> (→"Waveform Chart":dynamicdata)
        "String 4" <- "Combo Box"
      }
    }
    n922 = case shown="True" "Manual Ctrl" {
      tunnel: w36 -> [_ w1669]
      tunnel: "RLC on/off" -> [_ w1668]
      tunnel: [FALSE w1671] -> w38
      frame False {
      }
      frame True {
        w1683 = 0 ("polynomial order")
        n923 = for {
          N: "N to fit" -> [_]
          tunnel: [w2356] -> w1658 mode=indexing
          tunnel: [w2361] -> w1676 mode=indexing
          tunnel: [w2361] -> w1662 mode=indexing
          tunnel: [w2349] -> w1667 mode=indexing
          i -> [w2361]
          n924 = case shown="False" "Clear" {
            frame False {
            }
            frame True {
              n925 = property on="P-manual" class="WFChart (strict)"("History Data"=dynamicdata[] []) -> ()  [unwired: 2 in, 2 out]
            }
          }
          n926 = case shown="True" "Câmara" {
            frame False {
            }
            frame True {
              n927 = property on="Vol Ref" class="Slide (strict)"() -> ("Value"=w2408:dbl)  [unwired: 2 in, 2 out]
              n928 = local write "Camara"(w2408) -> ()
            }
          }
          n929 = case shown="True" "Guardar\nCinetica" {
            frame False {
            }
            frame True {
              n930 = feedback #2() -> (w2363:bool)  [unwired: 1 in]
              "x >= y?" <- w2363
              n931 = call "Elapsed Time"("Reset"=w2363) -> ("Elapsed Time (s)"=w2365:dbl)  [unwired: 11 in, 7 out]
              "Elapsed Time (sec)" <- w2365
              n932 = case shown="True" w2363 {
                frame False {
                }
                frame True {
                  n933 = flat-sequence {
                    tunnel: [w2380] -> w2368
                    tunnel: [w2379] -> w2367
                    tunnel: w2368 -> [w2398]
                    tunnel: w2367 -> [w2397]
                    frame #0 {
                      w2373 = "\t"
                      w2370 = i16 4 ("precision (6)")
                      n934 = property on="MEASURE C [F ]" class="DigNum (strict)"() -> ("Value"=w2369:dbl)  [unwired: 2 in, 2 out]
                      n935 = property on="termopar K" class="DigNum (strict)"() -> ("Value"=w2374:dbl)  [unwired: 2 in, 2 out]
                      n936 = Number To Fractional String(number=w2374, precision (6)=w2370) -> (F-format string=w2375:string)  [unwired: 2 in]
                      n937 = property on="P cinetica mean" class="DigNum (strict)"() -> ("Value"=w2377:dbl)  [unwired: 2 in, 2 out]
                      n938 = property on="T cinetica mean 2" class="DigNum (strict)"() -> ("Value"=w2376:dbl)  [unwired: 2 in, 2 out]
                      n939 = property on="path 2_cinetica" class="Path"() -> ("Value"=w2378:path)  [unwired: 2 in, 2 out]
                      n940 = Get Date/Time String(date format (0)=enum16{"short", "long", "abbreviated"}."short", want seconds? (F)=TRUE) -> (date string=w2394:string, time string=w2393:string)  [unwired: 1 in]
                      n941 = Number To Exponential String(number=w2369, precision (6)=w2370) -> (E-format string=w2372:string)  [unwired: 2 in]
                      n942 = Number To Fractional String(number=w2377, precision (6)=w2370) -> (F-format string=w2392:string)  [unwired: 2 in]
                      n943 = Number To Fractional String(number=w2376, precision (6)=w2370) -> (F-format string=w2391:string)  [unwired: 2 in]
                      n944 = Open/Create/Replace File(file path (use dialog)=w2378, operation (0:open)=T3."open") -> (refnum out=w2387:refnum<file>, error out=w2388:errorcluster)  [unwired: 2 in, 3 out]
                      n945 = Concatenate Strings(w2394, w2373, w2393, w2373, w2392, w2373, w2391, w2373, w2375, w2373, w2372, "\r\n") -> (w2381:string)
                      n946 = Set File Position(refnum=w2387, from (0:start)=enum16{"start", "end", "current"}."end", error in=w2388) -> (refnum out=w2385:refnum<file>, error out=w2384:errorcluster)  [unwired: 1 in]
                      n947 = Write to Text File(file (use dialog)=w2385, text=w2381, error in=w2384) -> (refnum out=w2389:refnum<file>, error out=w2390:errorcluster)  [unwired: 2 out]
                      n948 = Close File(refnum=w2389, error in=w2390) -> (path=w2380:path, error out=w2382:errorcluster)
                      n949 = call <vilib>:"Simple Error Handler.vi"("error in (no error)"=w2382) -> ("error out"=w2379:errorcluster)  [unwired: 1 in, 7 out]
                    }
                    frame #1 {
                      n950 = Read from Text File(file (use dialog)=w2398, count=-1 ("Count  3"), error in=w2397) -> (refnum out=w2399:refnum<file>, text=w2403:string, error out=w2400:errorcluster)  [unwired: 1 in, 1 out]
                      n951 = local write "String_cinetica"(w2403) -> ()
                      n952 = Close File(refnum=w2399, error in=w2400) -> (error out=w2401:errorcluster)  [unwired: 1 out]
                      n953 = call <vilib>:"Simple Error Handler.vi"("error in (no error)"=w2401) -> ()  [unwired: 1 in, 8 out]
                    }
                    frame #2 {
                      n954 = local write "P T  index"(0 ("P T  index")) -> ()
                      n955 = local write "T subarray 2"(dbl[] [0.0, 1.0] ("subarray")) -> ()
                      n956 = local write "P subarray"(dbl[] [0.0, 1.0] ("subarray")) -> ()
                    }
                  }
                }
              }
              n957 = Greater Or Equal?(x=w2365, y="seconds") -> (x >= y?=w2366:bool)
              n958 = feedback-in #2(w2366) -> ()
            }
          }
          n959 = property on="correção NTC" class="DigNum (strict)"() -> ("Value"=w2352:dbl)  [unwired: 2 in, 2 out]
          n960 = call "Read P T.vi"("correção NTC"=w2352) -> ("Sievert01"=w2345:dbl, "mean H2 sensor"=→"mean H2 sensor (V)":dbl, "termopar K"=w2350:dbl, "output NTC"=w2349:dbl, "P Set 2 Output 2"=w2348:dbl)  [unwired: 3 in, 7 out]
          "termopar K" <- w2350
          "output NTC" <- w2349
          n961 = stacked-sequence {
            tunnel: "Entrada Gás" -> [w2439 _ _ _]
            tunnel: "Vácuo" -> [_ w2451 _ _]
            tunnel: "Câmara" -> [_ _ w2463 _]
            tunnel: "ATM" -> [_ _ _ w2475]
            frame #0 {
              w2444 = T7 3 items=["no dialog", "OK message", "continue or stop message", "OK message + warnings", "continue/stop + warnings"] ("type of dialog (OK msg:1)")
              n962 = property on="Entrada gás" class="Bool (strict)"("Value"=w2439) -> ()  [unwired: 2 in, 2 out]
              n963 = call-poly <vilib>:"DAQmx Create Virtual Channel.vi"("lines"=tag "Dev1/port0/line1") -> ("task out"=w2442:refnum<k21>, "error out"=w2443:errorcluster)  [unwired: 13 in]
              n964 = call <vilib>:"DAQmx Start Task.vi"("task/channels in"=w2442, "error in"=w2443) -> ("task out"=w2445:refnum<k21>, "error out"=w2446:errorcluster)  [unwired: 12 in]
              n965 = call-poly <vilib>:"DAQmx Write.vi"("task/channels in"=w2445, "data"=w2439, "error in"=w2446) -> ("task out"=w2450:refnum<k21>, "error out"=w2447:errorcluster)  [unwired: 10 in, 1 out]
              n966 = call <vilib>:"DAQmx Stop Task.vi"("task/channels in"=w2450, "error in"=w2447) -> ("task out"=w2449:refnum<k21>, "error out"=w2448:errorcluster)  [unwired: 12 in]
              n967 = call <vilib>:"DAQmx Clear Task.vi"("task in"=w2449, "error in"=w2448) -> ("error out"=w2441:errorcluster)  [unwired: 13 in]
              n968 = call <vilib>:"Simple Error Handler.vi"("type of dialog (OK msg:1)"=w2444, "error in (no error)"=w2441) -> ()  [unwired: 3 in, 5 out]
            }
            frame #1 {
              w2456 = T7 3 items=["no dialog", "OK message", "continue or stop message", "OK message + warnings", "continue/stop + warnings"] ("type of dialog (OK msg:1)")
              n969 = property on="Vácuo" class="Bool (strict)"("Value"=w2451) -> ()  [unwired: 2 in, 2 out]
              n970 = call-poly <vilib>:"DAQmx Create Virtual Channel.vi"("lines"=tag "Dev1/port0/line2") -> ("task out"=w2454:refnum<k21>, "error out"=w2455:errorcluster)  [unwired: 13 in]
              n971 = call <vilib>:"DAQmx Start Task.vi"("task/channels in"=w2454, "error in"=w2455) -> ("task out"=w2457:refnum<k21>, "error out"=w2458:errorcluster)  [unwired: 12 in]
              n972 = call-poly <vilib>:"DAQmx Write.vi"("task/channels in"=w2457, "data"=w2451, "error in"=w2458) -> ("task out"=w2462:refnum<k21>, "error out"=w2459:errorcluster)  [unwired: 10 in, 1 out]
              n973 = call <vilib>:"DAQmx Stop Task.vi"("task/channels in"=w2462, "error in"=w2459) -> ("task out"=w2461:refnum<k21>, "error out"=w2460:errorcluster)  [unwired: 12 in]
              n974 = call <vilib>:"DAQmx Clear Task.vi"("task in"=w2461, "error in"=w2460) -> ("error out"=w2453:errorcluster)  [unwired: 13 in]
              n975 = call <vilib>:"Simple Error Handler.vi"("type of dialog (OK msg:1)"=w2456, "error in (no error)"=w2453) -> ()  [unwired: 3 in, 5 out]
            }
            frame #2 {
              w2468 = T7 3 items=["no dialog", "OK message", "continue or stop message", "OK message + warnings", "continue/stop + warnings"] ("type of dialog (OK msg:1)")
              n976 = property on="Câmara" class="Bool (strict)"("Value"=w2463) -> ()  [unwired: 2 in, 2 out]
              n977 = call-poly <vilib>:"DAQmx Create Virtual Channel.vi"("lines"=tag "Dev1/port0/line3") -> ("task out"=w2466:refnum<k21>, "error out"=w2467:errorcluster)  [unwired: 13 in]
              n978 = call <vilib>:"DAQmx Start Task.vi"("task/channels in"=w2466, "error in"=w2467) -> ("task out"=w2469:refnum<k21>, "error out"=w2470:errorcluster)  [unwired: 12 in]
              n979 = call-poly <vilib>:"DAQmx Write.vi"("task/channels in"=w2469, "data"=w2463, "error in"=w2470) -> ("task out"=w2474:refnum<k21>, "error out"=w2471:errorcluster)  [unwired: 10 in, 1 out]
              n980 = call <vilib>:"DAQmx Stop Task.vi"("task/channels in"=w2474, "error in"=w2471) -> ("task out"=w2473:refnum<k21>, "error out"=w2472:errorcluster)  [unwired: 12 in]
              n981 = call <vilib>:"DAQmx Clear Task.vi"("task in"=w2473, "error in"=w2472) -> ("error out"=w2465:errorcluster)  [unwired: 13 in]
              n982 = call <vilib>:"Simple Error Handler.vi"("type of dialog (OK msg:1)"=w2468, "error in (no error)"=w2465) -> ()  [unwired: 3 in, 5 out]
            }
            frame #3 {
              w2480 = T7 3 items=["no dialog", "OK message", "continue or stop message", "OK message + warnings", "continue/stop + warnings"] ("type of dialog (OK msg:1)")
              n983 = property on="Atm" class="Bool (strict)"("Value"=w2475) -> ()  [unwired: 2 in, 2 out]
              n984 = call-poly <vilib>:"DAQmx Create Virtual Channel.vi"("lines"=tag "Dev1/port0/line4") -> ("task out"=w2478:refnum<k21>, "error out"=w2479:errorcluster)  [unwired: 13 in]
              n985 = call <vilib>:"DAQmx Start Task.vi"("task/channels in"=w2478, "error in"=w2479) -> ("task out"=w2481:refnum<k21>, "error out"=w2482:errorcluster)  [unwired: 12 in]
              n986 = call-poly <vilib>:"DAQmx Write.vi"("task/channels in"=w2481, "data"=w2475, "error in"=w2482) -> ("task out"=w2486:refnum<k21>, "error out"=w2483:errorcluster)  [unwired: 10 in, 1 out]
              n987 = call <vilib>:"DAQmx Stop Task.vi"("task/channels in"=w2486, "error in"=w2483) -> ("task out"=w2485:refnum<k21>, "error out"=w2484:errorcluster)  [unwired: 12 in]
              n988 = call <vilib>:"DAQmx Clear Task.vi"("task in"=w2485, "error in"=w2484) -> ("error out"=w2477:errorcluster)  [unwired: 13 in]
              n989 = call <vilib>:"Simple Error Handler.vi"("type of dialog (OK msg:1)"=w2480, "error in (no error)"=w2477) -> ()  [unwired: 3 in, 5 out]
            }
          }
          n990 = Multiply(x=w2348, y=10.0) -> (x*y=w2356:dbl)
          n991 = local write "Vol Ref"(w2356) -> ()
          n992 = Multiply(x=w2345, y=10.0) -> (x*y=w2346:dbl)
          n993 = stacked-sequence {
            tunnel: w2356 -> [w2431 _]
            tunnel: w2349 -> [w2410 _]
            frame #0 {
              w2409 = 2 ("y")
              n994 = property on="P subarray" class="Arr (strict)"() -> ("Value"=w2433:dbl[])  [unwired: 2 in, 2 out]
              n995 = property on="P T  index" class="DigNum (strict)"() -> ("Value"=w2411:i32)  [unwired: 2 in, 2 out]
              n996 = Replace Array Subset(array=w2433, new element=w2431, index=w2411) -> (w2429:dbl[])
              n997 = property on="T subarray 2" class="Arr (strict)"() -> ("Value"=w2420:dbl[])  [unwired: 2 in, 2 out]
              n998 = Replace Array Subset(array=w2420, new element=w2410, index=w2411) -> (w2417:dbl[])
              n999 = call-poly <vilib>:"Array To Matrix.vi"("Real 1D Array"=w2429) -> ("Real Matrix (Column Vector)"=w2436:T5)
              n1000 = Matrix Size(0:w2436) -> (1:w2435:i32, 2:w2434:i32)
              n1001 = call-poly <vilib>:"Array To Matrix.vi"("Real 1D Array"=w2417) -> ("Real Matrix (Column Vector)"=w2423:T5)
              n1002 = Matrix Size(0:w2423) -> (1:w2422:i32, 2:w2421:i32)
              n1003 = Increment(x=w2435) -> (x+1=w2424:i32)
              n1004 = Subtract(x=w2424, y=w2409) -> (x-y=w2425:i32)
              n1005 = Resize Matrix(1:w2434, 2:w2424, 4:w2436) -> (0:w2432:T5)
              n1006 = Increment(x=w2422) -> (x+1=w2412:i32)
              n1007 = Subtract(x=w2412, y=w2409) -> (x-y=w2413:i32)
              n1008 = Resize Matrix(1:w2421, 2:w2412, 4:w2423) -> (0:w2419:T5)
              n1009 = call-poly <vilib>:"Matrix To Array.vi"("Real Matrix"=w2432) -> ("Real 2D Array"=w2427:dbl[][])
              n1010 = call-poly <vilib>:"Matrix To Array.vi"("Real Matrix"=w2419) -> ("Real 2D Array"=w2415:dbl[][])
              n1011 = Reshape Array(w2427, w2424) -> (w2426:dbl[])
              n1012 = Reshape Array(w2415, w2412) -> (w2414:dbl[])
              n1013 = local write "P subarray"(w2426) -> ()
              n1014 = Reshape Array(w2426, w2425) -> (w2428:dbl[])
              n1015 = local write "T subarray 2"(w2414) -> ()
              n1016 = call <vilib>:"Mean.vi"("X"=w2428) -> ("mean"=→"P cinetica mean":dbl)  [unwired: 1 out]
              n1017 = Reshape Array(w2414, w2413) -> (w2416:dbl[])
              n1018 = call <vilib>:"Mean.vi"("X"=w2416) -> ("mean"=→"T cinetica mean 2":dbl)  [unwired: 1 out]
            }
            frame #1 {
              n1019 = property on="P T  index" class="DigNum (strict)"() -> ("Value"=w2438:i32)  [unwired: 2 in, 2 out]
              n1020 = Increment(x=w2438) -> (x+1=w2437:i32)
              n1021 = local write "P T  index"(w2437) -> ()
            }
          }
          n1022 = Merge Signals(w2356, w2349, w2350, w2346) -> (→"P-manual":dynamicdata)
          "N" <- w2361
        }
        n1023 = case shown="True" "Save manual" {
          selector: "Save manual" -> [_ w2285]
          frame False {
          }
          frame True {
            n1024 = feedback #3() -> (w2281:dbl)  [unwired: 1 in]
            n1025 = Equal To 0?(x=w2281) -> (x = 0?=w2287:bool)
            n1026 = stacked-sequence {
              tunnel: w2287 -> [_ w2303 _]
              tunnel: [_ w2302 _] -> w2283
              frame #0 {
                w2296 = i16 3 ("precision (6)")
                n1027 = property on="T fit" class="DigNum (strict)"() -> ("Value"=w2298:dbl)  [unwired: 2 in, 2 out]
                n1028 = property on="p fit" class="DigNum (strict)"() -> ("Value"=w2299:dbl)  [unwired: 2 in, 2 out]
                n1029 = property on="termopar K" class="DigNum (strict)"() -> ("Value"=w2297:dbl)  [unwired: 2 in, 2 out]
                n1030 = Number To Fractional String(number=w2298, precision (6)=w2296) -> (F-format string=→"T string":string)  [unwired: 2 in]
                n1031 = Number To Fractional String(number=w2299, precision (6)=w2296) -> (F-format string=→"P string":string)  [unwired: 2 in]
                n1032 = Number To Fractional String(number=w2297, precision (6)=w2296) -> (F-format string=→"termopar K":string)  [unwired: 2 in]
              }
              frame #1 {
                n1033 = case shown="True" w2303 {
                  tunnel: [TRUE ("y") FALSE ("y")] -> w2302
                  frame False {
                    n1034 = property on="path" class="Path"() -> ("Value"=w2307:path)  [unwired: 2 in, 2 out]
                    n1035 = property on="P string" class="Str"() -> ("Value"=w2306:string)  [unwired: 2 in, 2 out]
                    n1036 = Concatenate Strings(w2306, "\t") -> (w2304:string)
                    n1037 = Open/Create/Replace File(file path (use dialog)=w2307, operation (0:open)=T3."open") -> (refnum out=w2311:refnum<file>, error out=w2310:errorcluster)  [unwired: 2 in, 3 out]
                    n1038 = Set File Position(refnum=w2311, from (0:start)=enum16{"start", "end", "current"}."end", error in=w2310) -> (refnum out=w2313:refnum<file>, error out=w2314:errorcluster)  [unwired: 1 in]
                    n1039 = Write to Text File(file (use dialog)=w2313, text=w2304, error in=w2314) -> (refnum out=w2309:refnum<file>, error out=w2308:errorcluster)  [unwired: 2 out]
                    n1040 = Close File(refnum=w2309, error in=w2308) -> (error out=w2316:errorcluster)  [unwired: 1 out]
                    n1041 = call <vilib>:"Simple Error Handler.vi"("error in (no error)"=w2316) -> ()  [unwired: 1 in, 8 out]
                  }
                  frame True {
                    w2319 = "\t"
                    n1042 = property on="path" class="Path"() -> ("Value"=w2326:path)  [unwired: 2 in, 2 out]
                    n1043 = property on="Count SET" class="DigNum (strict)"() -> ("Value"=w2322:i32)  [unwired: 2 in, 2 out]
                    n1044 = Open/Create/Replace File(file path (use dialog)=w2326, operation (0:open)=T3."open") -> (refnum out=w2325:refnum<file>, error out=w2324:errorcluster)  [unwired: 2 in, 3 out]
                    n1045 = Increment(x=w2322) -> (x+1=w2323:i32)
                    "Set atual" <- w2323
                    n1046 = Set File Position(refnum=w2325, from (0:start)=enum16{"start", "end", "current"}."end", error in=w2324) -> (refnum out=w2334:refnum<file>, error out=w2335:errorcluster)  [unwired: 1 in]
                    n1047 = Number To Decimal String(number=w2323) -> (decimal integer string=w2327:string)  [unwired: 1 in]
                    n1048 = property on="termopar K" class="Str"() -> ("Value"=w2318:string)  [unwired: 2 in, 2 out]
                    n1049 = property on="T string" class="Str"() -> ("Value"=w2320:string)  [unwired: 2 in, 2 out]
                    n1050 = Concatenate Strings(w2320, w2319, w2318, "\r\n", w2327, w2319) -> (w2329:string)
                    n1051 = Write to Text File(file (use dialog)=w2334, text=w2329, error in=w2335) -> (refnum out=w2332:refnum<file>, error out=w2331:errorcluster)  [unwired: 2 out]
                    n1052 = Close File(refnum=w2332, error in=w2331) -> (error out=w2337:errorcluster)  [unwired: 1 out]
                    n1053 = call <vilib>:"Simple Error Handler.vi"("error in (no error)"=w2337) -> ()  [unwired: 1 in, 8 out]
                    "T" <- TRUE ("T")
                  }
                }
              }
              frame #2 {
                n1054 = property on="path" class="Path"() -> ("Value"=w2339:path)  [unwired: 2 in, 2 out]
                n1055 = property on="Set atual" class="DigNum (strict)"() -> ("Value"=w2338:i32)  [unwired: 2 in, 2 out]
                n1056 = local write "Count SET"(w2338) -> ()
                n1057 = Read from Text File(file (use dialog)=w2339, count=-1 ("Count  3")) -> (refnum out=w2341:refnum<file>, text=w2340:string, error out=w2342:errorcluster)  [unwired: 2 in, 1 out]
                n1058 = property on="String 2" class="Str"("Value"=w2340) -> ()  [unwired: 2 in, 2 out]
                n1059 = Close File(refnum=w2341, error in=w2342) -> (error out=w2344:errorcluster)  [unwired: 1 out]
                n1060 = call <vilib>:"Simple Error Handler.vi"("error in (no error)"=w2344) -> ()  [unwired: 1 in, 8 out]
              }
            }
            n1061 = Implies(1:w2283, 2:w2285) -> (0:w2284:bool)
            n1062 = Select(t=w2281, s=w2284, f=5.0 ("t")) -> (s? t:f=w2282:dbl)
            n1063 = case shown="1" w2282 {
              frame 0, Default {
              }
              frame 1 {
                "ZPf2" <- TRUE ("ZPf2")
              }
              frame 2 {
                "Pf2" <- TRUE ("Pf2")
              }
              frame 3 {
                "Pit" <- TRUE ("Pit")
              }
              frame 4 {
                n1064 = local write "T"(FALSE ("T")) -> ()
                "ZPit" <- TRUE ("ZPit")
              }
              frame 5 {
                w2294 = FALSE
                n1065 = local write "Pit"(w2294) -> ()
                n1066 = local write "ZPf2"(w2294) -> ()
                n1067 = local write "ZPit"(w2294) -> ()
                n1068 = local write "Pf2"(w2294) -> ()
              }
            }
            n1069 = Decrement(x=w2282) -> (x-1=w2288:dbl)
            n1070 = feedback-in #3(w2288) -> ()
          }
        }
        n1071 = case shown="True" w1668 {
          tunnel: [FALSE ("Save manual") w2280] -> w1670
          tunnel: "Save manual" -> [_ w2280]
          frame False {
          }
          frame True {
          }
        }
        n1072 = case shown="True" w1668 {
          tunnel: [FALSE w1688] -> w1671
          tunnel: w1670 -> [_ w1687]
          tunnel: w1669 -> [_ w1686]
          frame False {
          }
          frame True {
            n1073 = flat-sequence {
              tunnel: w1686 -> [w1709]
              tunnel: w1687 -> [w1710]
              tunnel: [w1710] -> w1707
              tunnel: [w1709] -> w1706
              tunnel: [w1717] -> w1705
              tunnel: [w1718] -> w1704
              tunnel: [w1719] -> w1703
              tunnel: [w1720] -> w1702
              tunnel: [w1721] -> w1701
              tunnel: [w1722] -> w1700
              tunnel: [w1723] -> w1699
              tunnel: [w1725] -> w1698
              tunnel: [w1726] -> w1697
              tunnel: [w1727] -> w1696
              tunnel: [w1728] -> w1695
              tunnel: [w1729] -> w1694
              tunnel: [w1724] -> w1693
              tunnel: [w1716] -> w1692
              tunnel: [w1715] -> w1691
              tunnel: [w1714] -> w1690
              tunnel: [w1713] -> w1689
              tunnel: w1707 -> [w1712]
              tunnel: w1706 -> [w1711]
              tunnel: w1705 -> [w2227]
              tunnel: w1704 -> [w2226]
              tunnel: w1703 -> [w2225]
              tunnel: w1702 -> [w2224]
              tunnel: w1701 -> [w2223]
              tunnel: w1700 -> [w2222]
              tunnel: w1699 -> [w2221]
              tunnel: w1698 -> [w2220]
              tunnel: w1697 -> [w2219]
              tunnel: w1696 -> [w2218]
              tunnel: w1695 -> [w2217]
              tunnel: w1694 -> [w2216]
              tunnel: w1693 -> [w2215]
              tunnel: w1692 -> [w2228]
              tunnel: w1691 -> [w2229]
              tunnel: w1690 -> [w2230]
              tunnel: [w2213] -> w1688
              tunnel: w1689 -> [w2213]
              tunnel: [TRUE] -> w1685
              frame #0 {
                n1074 = local write "graph RLC"(FALSE) -> ()
              }
              frame #1 {
                n1075 = case shown="True" w1712 {
                  tunnel: [_ w1764] -> w1713
                  tunnel: w1711 -> [_ w1746]
                  tunnel: [_ w1745] -> w1714
                  tunnel: [_ w1744] -> w1715
                  tunnel: [_ w1743] -> w1716
                  tunnel: [_ w1742] -> w1717
                  tunnel: [_ w1741] -> w1718
                  tunnel: [_ w1740] -> w1719
                  tunnel: [_ w1739] -> w1720
                  tunnel: [_ w1738] -> w1721
                  tunnel: [_ w1737] -> w1722
                  tunnel: [_ w1736] -> w1723
                  tunnel: [_ w1735] -> w1724
                  tunnel: [_ w1734] -> w1725
                  tunnel: [_ w1733] -> w1726
                  tunnel: [_ w1732] -> w1727
                  tunnel: [_ w1731] -> w1728
                  tunnel: [_ w1730] -> w1729
                  frame False {
                  }
                  frame True {
                    n1076 = for {
                      N: 5 -> [_]
                      tunnel: TRUE -> [w1787]
                      tunnel: FALSE -> [w1786]
                      tunnel: [w1785] -> w1764
                      tunnel: [w1784] -> w1762 mode=indexing
                      tunnel: [w1783] -> w1761 mode=indexing
                      tunnel: [w1782] -> w1760 mode=indexing
                      tunnel: [w1781] -> w1759 mode=indexing
                      tunnel: [w1780] -> w1758 mode=indexing
                      tunnel: [w1779] -> w1757 mode=indexing
                      tunnel: [w1778] -> w1756 mode=indexing
                      tunnel: [w1777] -> w1755 mode=indexing
                      tunnel: [w1776] -> w1754 mode=indexing
                      tunnel: [w1775] -> w1753 mode=indexing
                      tunnel: [w1774] -> w1752 mode=indexing
                      tunnel: [w1773] -> w1751 mode=indexing
                      tunnel: [w1772] -> w1750 mode=indexing
                      tunnel: [w1771] -> w1749 mode=indexing
                      tunnel: [w1770] -> w1748 mode=indexing
                      tunnel: [w1769] -> w1747 mode=indexing
                      tunnel: w1746 -> [w1768]
                      n1077 = property on="path RLC_completo" class="Path"() -> ("Value"=w1767:path)  [unwired: 2 in, 2 out]
                      n1078 = stacked-sequence {
                        tunnel: w1787 -> [_ w1812 w1837 w1862 w1887 w1912 w1937 w1962 w1985 w2010 w2037 w2060 w2087 w2112 w2137 w2160 w2187 _]
                        tunnel: w1786 -> [w1788 _ _ _ _ _ _ _ _ _ _ _ _ _ _ _ _ w2211]
                        tunnel: [_ _ _ _ _ _ _ _ _ _ _ _ _ _ _ _ _ TRUE] -> w1785
                        tunnel: [_ w1811 _ _ _ _ _ _ _ _ _ _ _ _ _ _ _ _] -> w1784
                        tunnel: [_ _ w1836 _ _ _ _ _ _ _ _ _ _ _ _ _ _ _] -> w1783
                        tunnel: [_ _ _ w1861 _ _ _ _ _ _ _ _ _ _ _ _ _ _] -> w1782
                        tunnel: [_ _ _ _ w1886 _ _ _ _ _ _ _ _ _ _ _ _ _] -> w1781
                        tunnel: [_ _ _ _ _ w1911 _ _ _ _ _ _ _ _ _ _ _ _] -> w1780
                        tunnel: [_ _ _ _ _ _ w1936 _ _ _ _ _ _ _ _ _ _ _] -> w1779
                        tunnel: [_ _ _ _ _ _ _ w1961 _ _ _ _ _ _ _ _ _ _] -> w1778
                        tunnel: [_ _ _ _ _ _ _ _ w1987 _ _ _ _ _ _ _ _ _] -> w1777
                        tunnel: [_ _ _ _ _ _ _ _ _ w2012 _ _ _ _ _ _ _ _] -> w1776
                        tunnel: [_ _ _ _ _ _ _ _ _ _ w2036 _ _ _ _ _ _ _] -> w1775
                        tunnel: [_ _ _ _ _ _ _ _ _ _ _ w2062 _ _ _ _ _ _] -> w1774
                        tunnel: [_ _ _ _ _ _ _ _ _ _ _ _ w2086 _ _ _ _ _] -> w1773
                        tunnel: [_ _ _ _ _ _ _ _ _ _ _ _ _ w2111 _ _ _ _] -> w1772
                        tunnel: [_ _ _ _ _ _ _ _ _ _ _ _ _ _ w2136 _ _ _] -> w1771
                        tunnel: [_ _ _ _ _ _ _ _ _ _ _ _ _ _ _ w2162 _ _] -> w1770
                        tunnel: [_ _ _ _ _ _ _ _ _ _ _ _ _ _ _ _ w2186 _] -> w1769
                        tunnel: w1768 -> [_ w1814 w1840 w1864 w1889 w1914 w1939 w1964 w1989 w2014 w2039 w2064 w2089 w2114 w2139 w2164 w2189 _]
                        tunnel: w1767 -> [w1790 w1813 w1839 w1863 w1888 w1913 w1938 w1963 w1988 w2013 w2038 w2063 w2088 w2113 w2138 w2163 w2188 _]
                        frame #0 {
                          w1791 = "\t"
                          n1079 = local write "C-50-L"(w1788) -> ()
                          n1080 = local write "C-50-N"(w1788) -> ()
                          n1081 = local write "Z-50-L"(w1788) -> ()
                          n1082 = local write "Z-50-N"(w1788) -> ()
                          n1083 = local write "C-1K-L"(w1788) -> ()
                          n1084 = local write "C-1K-N"(w1788) -> ()
                          n1085 = local write "Z-1K-N"(w1788) -> ()
                          n1086 = local write "Z-1K-L"(w1788) -> ()
                          n1087 = local write "Z-100-L"(w1788) -> ()
                          n1088 = local write "C-10K-L"(w1788) -> ()
                          n1089 = local write "C-100-N"(w1788) -> ()
                          n1090 = local write "C-10K-N"(w1788) -> ()
                          n1091 = local write "Z-10K-N"(w1788) -> ()
                          n1092 = local write "Z-10K-L"(w1788) -> ()
                          n1093 = local write "Z-100-N"(w1788) -> ()
                          n1094 = local write "C-100-L"(w1788) -> ()
                          n1095 = Open/Create/Replace File(file path (use dialog)=w1790, operation (0:open)=T3."open") -> (refnum out=w1804:refnum<file>, error out=w1803:errorcluster)  [unwired: 2 in, 3 out]
                          n1096 = Get Date/Time String(date format (0)=enum16{"short", "long", "abbreviated"}."short", want seconds? (F)=TRUE) -> (date string=w1796:string, time string=w1795:string)  [unwired: 1 in]
                          n1097 = feedback #4() -> (w1789:dbl)  [unwired: 1 in]
                          n1098 = local write "SET 2"(w1789) -> ()
                          n1099 = Set File Position(refnum=w1804, from (0:start)=enum16{"start", "end", "current"}."end", error in=w1803) -> (refnum out=w1806:refnum<file>, error out=w1807:errorcluster)  [unwired: 1 in]
                          n1100 = Number To Fractional String(number=w1789, precision (6)=i16 2) -> (F-format string=w1794:string)  [unwired: 2 in]
                          n1101 = Add(x=w1789, y=0.2) -> (x+y=w1800:dbl)
                          n1102 = feedback-in #4(w1800) -> ()
                          n1103 = Concatenate Strings(w1794, w1791, w1796, w1791, w1795, w1791) -> (w1793:string)
                          n1104 = Write to Text File(file (use dialog)=w1806, text=w1793, error in=w1807) -> (refnum out=w1802:refnum<file>, error out=w1801:errorcluster)  [unwired: 1 in, 1 out]
                          n1105 = Close File(refnum=w1802, error in=w1801) -> (error out=w1809:errorcluster)  [unwired: 1 out]
                          n1106 = call <vilib>:"Simple Error Handler.vi"("error in (no error)"=w1809) -> ()  [unwired: 1 in, 8 out]
                        }
                        frame #1 {
                          w1815 = "\t"
                          w1832 = i16 4 ("width (-)")
                          n1107 = local write "C-50-L"(w1812) -> ()
                          n1108 = Wait (ms)(milliseconds to wait=u32 5000) -> ()  [unwired: 1 out]
                          n1109 = Open/Create/Replace File(file path (use dialog)=w1813, operation (0:open)=T3."open") -> (refnum out=w1824:refnum<file>, error out=w1823:errorcluster)  [unwired: 2 in, 3 out]
                          n1110 = Set File Position(refnum=w1824, from (0:start)=enum16{"start", "end", "current"}."end", error in=w1823) -> (refnum out=w1826:refnum<file>, error out=w1827:errorcluster)  [unwired: 1 in]
                          n1111 = call "RLC_read.vi"("Path"=w1814, "String"="cmd /c rlc_read_cAL.py") -> ("MEASURE A"=w1811:dbl, "MEASURE V [V]"=w1831:dbl, "MEASURE B"=w1810:dbl, "MEASURE I [A]"=w1830:dbl)  [unwired: 2 out]
                          n1112 = Number To Engineering String(2:w1832, 4:w1830) -> (0:w1816:string)  [unwired: 2 in]
                          n1113 = local write "MEASURE A"(w1811) -> ()
                          n1114 = local write "MEASURE B"(w1810) -> ()
                          n1115 = Number To Engineering String(2:w1832, 4:w1831) -> (0:w1817:string)  [unwired: 2 in]
                          n1116 = Number To Engineering String(2:w1832, 4:w1811) -> (0:w1819:string)  [unwired: 2 in]
                          n1117 = Number To Engineering String(2:w1832, 4:w1810) -> (0:w1818:string)  [unwired: 2 in]
                          n1118 = Concatenate Strings(w1819, w1815, w1818, w1815, w1817, w1815, w1816, w1815) -> (w1820:string)
                          n1119 = Write to Text File(file (use dialog)=w1826, text=w1820, error in=w1827) -> (refnum out=w1822:refnum<file>, error out=w1821:errorcluster)  [unwired: 1 in, 1 out]
                          n1120 = Close File(refnum=w1822, error in=w1821) -> (error out=w1829:errorcluster)  [unwired: 1 out]
                          n1121 = call <vilib>:"Simple Error Handler.vi"("error in (no error)"=w1829) -> ()  [unwired: 1 in, 8 out]
                        }
                        frame #2 {
                          w1843 = "\t"
                          w1857 = i16 4 ("width (-)")
                          n1122 = local write "C-50-N"(w1837) -> ()
                          n1123 = Wait (ms)(milliseconds to wait=u32 5000) -> ()  [unwired: 1 out]
                          n1124 = Open/Create/Replace File(file path (use dialog)=w1839, operation (0:open)=T3."open") -> (refnum out=w1851:refnum<file>, error out=w1850:errorcluster)  [unwired: 2 in, 3 out]
                          n1125 = Set File Position(refnum=w1851, from (0:start)=enum16{"start", "end", "current"}."end", error in=w1850) -> (refnum out=w1853:refnum<file>, error out=w1854:errorcluster)  [unwired: 1 in]
                          n1126 = call "RLC_read.vi"("Path"=w1840, "String"="cmd /c rlc_read_cAN.py") -> ("MEASURE A"=w1836:dbl, "MEASURE V [V]"=w1842:dbl, "MEASURE B"=w1835:dbl, "MEASURE I [A]"=w1841:dbl)  [unwired: 2 out]
                          n1127 = Number To Engineering String(2:w1857, 4:w1841) -> (0:w1844:string)  [unwired: 2 in]
                          n1128 = local write "MEASURE A 2"(w1836) -> ()
                          n1129 = local write "MEASURE B 2"(w1835) -> ()
                          n1130 = Number To Engineering String(2:w1857, 4:w1842) -> (0:w1845:string)  [unwired: 2 in]
                          n1131 = Number To Engineering String(2:w1857, 4:w1836) -> (0:w1847:string)  [unwired: 2 in]
                          n1132 = Number To Engineering String(2:w1857, 4:w1835) -> (0:w1846:string)  [unwired: 2 in]
                          n1133 = Concatenate Strings(w1847, w1843, w1846, w1843, w1845, w1843, w1844, w1843) -> (w1838:string)
                          n1134 = Write to Text File(file (use dialog)=w1853, text=w1838, error in=w1854) -> (refnum out=w1849:refnum<file>, error out=w1848:errorcluster)  [unwired: 1 in, 1 out]
                          n1135 = Close File(refnum=w1849, error in=w1848) -> (error out=w1856:errorcluster)  [unwired: 1 out]
                          n1136 = call <vilib>:"Simple Error Handler.vi"("error in (no error)"=w1856) -> ()  [unwired: 1 in, 8 out]
                        }
                        frame #3 {
                          w1867 = "\t"
                          w1882 = i16 4 ("width (-)")
                          n1137 = Wait (ms)(milliseconds to wait=u32 5000) -> ()  [unwired: 1 out]
                          n1138 = local write "C-100-L"(w1862) -> ()
                          n1139 = Open/Create/Replace File(file path (use dialog)=w1863, operation (0:open)=T3."open") -> (refnum out=w1876:refnum<file>, error out=w1875:errorcluster)  [unwired: 2 in, 3 out]
                          n1140 = Set File Position(refnum=w1876, from (0:start)=enum16{"start", "end", "current"}."end", error in=w1875) -> (refnum out=w1878:refnum<file>, error out=w1879:errorcluster)  [unwired: 1 in]
                          n1141 = call "RLC_read.vi"("Path"=w1864, "String"="cmd /c rlc_read_cBL.py") -> ("MEASURE A"=w1861:dbl, "MEASURE V [V]"=w1866:dbl, "MEASURE B"=w1860:dbl, "MEASURE I [A]"=w1865:dbl)  [unwired: 2 out]
                          n1142 = Number To Engineering String(2:w1882, 4:w1865) -> (0:w1868:string)  [unwired: 2 in]
                          n1143 = local write "MEASURE A 3"(w1861) -> ()
                          n1144 = local write "MEASURE B 3"(w1860) -> ()
                          n1145 = Number To Engineering String(2:w1882, 4:w1866) -> (0:w1869:string)  [unwired: 2 in]
                          n1146 = Number To Engineering String(2:w1882, 4:w1861) -> (0:w1871:string)  [unwired: 2 in]
                          n1147 = Number To Engineering String(2:w1882, 4:w1860) -> (0:w1870:string)  [unwired: 2 in]
                          n1148 = Concatenate Strings(w1871, w1867, w1870, w1867, w1869, w1867, w1868, w1867) -> (w1872:string)
                          n1149 = Write to Text File(file (use dialog)=w1878, text=w1872, error in=w1879) -> (refnum out=w1874:refnum<file>, error out=w1873:errorcluster)  [unwired: 1 in, 1 out]
                          n1150 = Close File(refnum=w1874, error in=w1873) -> (error out=w1881:errorcluster)  [unwired: 1 out]
                          n1151 = call <vilib>:"Simple Error Handler.vi"("error in (no error)"=w1881) -> ()  [unwired: 1 in, 8 out]
                        }
                        frame #4 {
                          w1892 = "\t"
                          w1907 = i16 4 ("width (-)")
                          n1152 = Wait (ms)(milliseconds to wait=u32 5000) -> ()  [unwired: 1 out]
                          n1153 = local write "C-100-N"(w1887) -> ()
                          n1154 = Open/Create/Replace File(file path (use dialog)=w1888, operation (0:open)=T3."open") -> (refnum out=w1901:refnum<file>, error out=w1900:errorcluster)  [unwired: 2 in, 3 out]
                          n1155 = Set File Position(refnum=w1901, from (0:start)=enum16{"start", "end", "current"}."end", error in=w1900) -> (refnum out=w1903:refnum<file>, error out=w1904:errorcluster)  [unwired: 1 in]
                          n1156 = call "RLC_read.vi"("Path"=w1889, "String"="cmd /c rlc_read_cBN.py") -> ("MEASURE A"=w1886:dbl, "MEASURE V [V]"=w1891:dbl, "MEASURE B"=w1885:dbl, "MEASURE I [A]"=w1890:dbl)  [unwired: 2 out]
                          n1157 = Number To Engineering String(2:w1907, 4:w1890) -> (0:w1893:string)  [unwired: 2 in]
                          n1158 = local write "MEASURE A 4"(w1886) -> ()
                          n1159 = local write "MEASURE B 4"(w1885) -> ()
                          n1160 = Number To Engineering String(2:w1907, 4:w1891) -> (0:w1894:string)  [unwired: 2 in]
                          n1161 = Number To Engineering String(2:w1907, 4:w1886) -> (0:w1896:string)  [unwired: 2 in]
                          n1162 = Number To Engineering String(2:w1907, 4:w1885) -> (0:w1895:string)  [unwired: 2 in]
                          n1163 = Concatenate Strings(w1896, w1892, w1895, w1892, w1894, w1892, w1893, w1892) -> (w1897:string)
                          n1164 = Write to Text File(file (use dialog)=w1903, text=w1897, error in=w1904) -> (refnum out=w1899:refnum<file>, error out=w1898:errorcluster)  [unwired: 1 in, 1 out]
                          n1165 = Close File(refnum=w1899, error in=w1898) -> (error out=w1906:errorcluster)  [unwired: 1 out]
                          n1166 = call <vilib>:"Simple Error Handler.vi"("error in (no error)"=w1906) -> ()  [unwired: 1 in, 8 out]
                        }
                        frame #5 {
                          w1932 = "\t"
                          w1917 = i16 4 ("width (-)")
                          n1167 = local write "C-1K-L"(w1912) -> ()
                          n1168 = Wait (ms)(milliseconds to wait=u32 5000) -> ()  [unwired: 1 out]
                          n1169 = Open/Create/Replace File(file path (use dialog)=w1913, operation (0:open)=T3."open") -> (refnum out=w1923:refnum<file>, error out=w1924:errorcluster)  [unwired: 2 in, 3 out]
                          n1170 = Set File Position(refnum=w1923, from (0:start)=enum16{"start", "end", "current"}."end", error in=w1924) -> (refnum out=w1921:refnum<file>, error out=w1920:errorcluster)  [unwired: 1 in]
                          n1171 = call "RLC_read.vi"("Path"=w1914, "String"="cmd /c rlc_read_cCL.py") -> ("MEASURE A"=w1911:dbl, "MEASURE V [V]"=w1916:dbl, "MEASURE B"=w1910:dbl, "MEASURE I [A]"=w1915:dbl)  [unwired: 2 out]
                          n1172 = Number To Engineering String(2:w1917, 4:w1915) -> (0:w1931:string)  [unwired: 2 in]
                          n1173 = local write "MEASURE A 5"(w1911) -> ()
                          n1174 = local write "MEASURE B 5"(w1910) -> ()
                          n1175 = Number To Engineering String(2:w1917, 4:w1916) -> (0:w1930:string)  [unwired: 2 in]
                          n1176 = Number To Engineering String(2:w1917, 4:w1911) -> (0:w1928:string)  [unwired: 2 in]
                          n1177 = Number To Engineering String(2:w1917, 4:w1910) -> (0:w1929:string)  [unwired: 2 in]
                          n1178 = Concatenate Strings(w1928, w1932, w1929, w1932, w1930, w1932, w1931, w1932) -> (w1927:string)
                          n1179 = Write to Text File(file (use dialog)=w1921, text=w1927, error in=w1920) -> (refnum out=w1925:refnum<file>, error out=w1926:errorcluster)  [unwired: 1 in, 1 out]
                          n1180 = Close File(refnum=w1925, error in=w1926) -> (error out=w1918:errorcluster)  [unwired: 1 out]
                          n1181 = call <vilib>:"Simple Error Handler.vi"("error in (no error)"=w1918) -> ()  [unwired: 1 in, 8 out]
                        }
                        frame #6 {
                          w1957 = "\t"
                          w1942 = i16 4 ("width (-)")
                          n1182 = local write "C-1K-N"(w1937) -> ()
                          n1183 = Wait (ms)(milliseconds to wait=u32 5000) -> ()  [unwired: 1 out]
                          n1184 = Open/Create/Replace File(file path (use dialog)=w1938, operation (0:open)=T3."open") -> (refnum out=w1948:refnum<file>, error out=w1949:errorcluster)  [unwired: 2 in, 3 out]
                          n1185 = Set File Position(refnum=w1948, from (0:start)=enum16{"start", "end", "current"}."end", error in=w1949) -> (refnum out=w1946:refnum<file>, error out=w1945:errorcluster)  [unwired: 1 in]
                          n1186 = call "RLC_read.vi"("Path"=w1939, "String"="cmd /c rlc_read_cCN.py") -> ("MEASURE A"=w1936:dbl, "MEASURE V [V]"=w1941:dbl, "MEASURE B"=w1935:dbl, "MEASURE I [A]"=w1940:dbl)  [unwired: 2 out]
                          n1187 = Number To Engineering String(2:w1942, 4:w1940) -> (0:w1956:string)  [unwired: 2 in]
                          n1188 = local write "MEASURE A 6"(w1936) -> ()
                          n1189 = local write "MEASURE B 6"(w1935) -> ()
                          n1190 = Number To Engineering String(2:w1942, 4:w1941) -> (0:w1955:string)  [unwired: 2 in]
                          n1191 = Number To Engineering String(2:w1942, 4:w1936) -> (0:w1953:string)  [unwired: 2 in]
                          n1192 = Number To Engineering String(2:w1942, 4:w1935) -> (0:w1954:string)  [unwired: 2 in]
                          n1193 = Concatenate Strings(w1953, w1957, w1954, w1957, w1955, w1957, w1956, w1957) -> (w1952:string)
                          n1194 = Write to Text File(file (use dialog)=w1946, text=w1952, error in=w1945) -> (refnum out=w1950:refnum<file>, error out=w1951:errorcluster)  [unwired: 1 in, 1 out]
                          n1195 = Close File(refnum=w1950, error in=w1951) -> (error out=w1943:errorcluster)  [unwired: 1 out]
                          n1196 = call <vilib>:"Simple Error Handler.vi"("error in (no error)"=w1943) -> ()  [unwired: 1 in, 8 out]
                        }
                        frame #7 {
                          w1967 = "\t"
                          w1982 = i16 4 ("width (-)")
                          n1197 = Wait (ms)(milliseconds to wait=u32 5000) -> ()  [unwired: 1 out]
                          n1198 = local write "C-10K-L"(w1962) -> ()
                          n1199 = Open/Create/Replace File(file path (use dialog)=w1963, operation (0:open)=T3."open") -> (refnum out=w1976:refnum<file>, error out=w1975:errorcluster)  [unwired: 2 in, 3 out]
                          n1200 = Set File Position(refnum=w1976, from (0:start)=enum16{"start", "end", "current"}."end", error in=w1975) -> (refnum out=w1978:refnum<file>, error out=w1979:errorcluster)  [unwired: 1 in]
                          n1201 = call "RLC_read.vi"("Path"=w1964, "String"="cmd /c rlc_read_cDL.py") -> ("MEASURE A"=w1961:dbl, "MEASURE V [V]"=w1966:dbl, "MEASURE B"=w1960:dbl, "MEASURE I [A]"=w1965:dbl)  [unwired: 2 out]
                          n1202 = Number To Engineering String(2:w1982, 4:w1965) -> (0:w1968:string)  [unwired: 2 in]
                          n1203 = local write "MEASURE A 7"(w1961) -> ()
                          n1204 = local write "MEASURE B 7"(w1960) -> ()
                          n1205 = Number To Engineering String(2:w1982, 4:w1966) -> (0:w1969:string)  [unwired: 2 in]
                          n1206 = Number To Engineering String(2:w1982, 4:w1961) -> (0:w1971:string)  [unwired: 2 in]
                          n1207 = Number To Engineering String(2:w1982, 4:w1960) -> (0:w1970:string)  [unwired: 2 in]
                          n1208 = Concatenate Strings(w1971, w1967, w1970, w1967, w1969, w1967, w1968, w1967) -> (w1972:string)
                          n1209 = Write to Text File(file (use dialog)=w1978, text=w1972, error in=w1979) -> (refnum out=w1974:refnum<file>, error out=w1973:errorcluster)  [unwired: 1 in, 1 out]
                          n1210 = Close File(refnum=w1974, error in=w1973) -> (error out=w1981:errorcluster)  [unwired: 1 out]
                          n1211 = call <vilib>:"Simple Error Handler.vi"("error in (no error)"=w1981) -> ()  [unwired: 1 in, 8 out]
                        }
                        frame #8 {
                          w1992 = "\t"
                          w2007 = i16 4 ("width (-)")
                          n1212 = Wait (ms)(milliseconds to wait=u32 5000) -> ()  [unwired: 1 out]
                          n1213 = local write "C-10K-N"(w1985) -> ()
                          n1214 = Open/Create/Replace File(file path (use dialog)=w1988, operation (0:open)=T3."open") -> (refnum out=w2001:refnum<file>, error out=w2000:errorcluster)  [unwired: 2 in, 3 out]
                          n1215 = Set File Position(refnum=w2001, from (0:start)=enum16{"start", "end", "current"}."end", error in=w2000) -> (refnum out=w2003:refnum<file>, error out=w2004:errorcluster)  [unwired: 1 in]
                          n1216 = call "RLC_read.vi"("Path"=w1989, "String"="cmd /c rlc_read_cDN.py") -> ("MEASURE A"=w1987:dbl, "MEASURE V [V]"=w1991:dbl, "MEASURE B"=w1986:dbl, "MEASURE I [A]"=w1990:dbl)  [unwired: 2 out]
                          n1217 = Number To Engineering String(2:w2007, 4:w1990) -> (0:w1993:string)  [unwired: 2 in]
                          n1218 = local write "MEASURE A 8"(w1987) -> ()
                          n1219 = local write "MEASURE B 8"(w1986) -> ()
                          n1220 = Number To Engineering String(2:w2007, 4:w1991) -> (0:w1994:string)  [unwired: 2 in]
                          n1221 = Number To Engineering String(2:w2007, 4:w1987) -> (0:w1996:string)  [unwired: 2 in]
                          n1222 = Number To Engineering String(2:w2007, 4:w1986) -> (0:w1995:string)  [unwired: 2 in]
                          n1223 = Concatenate Strings(w1996, w1992, w1995, w1992, w1994, w1992, w1993, w1992) -> (w1997:string)
                          n1224 = Write to Text File(file (use dialog)=w2003, text=w1997, error in=w2004) -> (refnum out=w1999:refnum<file>, error out=w1998:errorcluster)  [unwired: 1 in, 1 out]
                          n1225 = Close File(refnum=w1999, error in=w1998) -> (error out=w2006:errorcluster)  [unwired: 1 out]
                          n1226 = call <vilib>:"Simple Error Handler.vi"("error in (no error)"=w2006) -> ()  [unwired: 1 in, 8 out]
                        }
                        frame #9 {
                          w2017 = "\t"
                          w2032 = i16 4 ("width (-)")
                          n1227 = local write "Z-50-L"(w2010) -> ()
                          n1228 = Wait (ms)(milliseconds to wait=u32 5000) -> ()  [unwired: 1 out]
                          n1229 = Open/Create/Replace File(file path (use dialog)=w2013, operation (0:open)=T3."open") -> (refnum out=w2026:refnum<file>, error out=w2025:errorcluster)  [unwired: 2 in, 3 out]
                          n1230 = Set File Position(refnum=w2026, from (0:start)=enum16{"start", "end", "current"}."end", error in=w2025) -> (refnum out=w2028:refnum<file>, error out=w2029:errorcluster)  [unwired: 1 in]
                          n1231 = call "RLC_read.vi"("Path"=w2014, "String"="cmd /c rlc_read_ZAL.py") -> ("MEASURE A"=w2012:dbl, "MEASURE V [V]"=w2016:dbl, "MEASURE B"=w2011:dbl, "MEASURE I [A]"=w2015:dbl)  [unwired: 2 out]
                          n1232 = Number To Engineering String(2:w2032, 4:w2015) -> (0:w2018:string)  [unwired: 2 in]
                          n1233 = local write "MEASURE A 9"(w2012) -> ()
                          n1234 = local write "MEASURE B 9"(w2011) -> ()
                          n1235 = Number To Engineering String(2:w2032, 4:w2016) -> (0:w2019:string)  [unwired: 2 in]
                          n1236 = Number To Engineering String(2:w2032, 4:w2012) -> (0:w2021:string)  [unwired: 2 in]
                          n1237 = Number To Engineering String(2:w2032, 4:w2011) -> (0:w2020:string)  [unwired: 2 in]
                          n1238 = Concatenate Strings(w2021, w2017, w2020, w2017, w2019, w2017, w2018, w2017) -> (w2022:string)
                          n1239 = Write to Text File(file (use dialog)=w2028, text=w2022, error in=w2029) -> (refnum out=w2024:refnum<file>, error out=w2023:errorcluster)  [unwired: 1 in, 1 out]
                          n1240 = Close File(refnum=w2024, error in=w2023) -> (error out=w2031:errorcluster)  [unwired: 1 out]
                          n1241 = call <vilib>:"Simple Error Handler.vi"("error in (no error)"=w2031) -> ()  [unwired: 1 in, 8 out]
                        }
                        frame #10 {
                          w2042 = "\t"
                          w2057 = i16 4 ("width (-)")
                          n1242 = local write "Z-50-N"(w2037) -> ()
                          n1243 = Wait (ms)(milliseconds to wait=u32 5000) -> ()  [unwired: 1 out]
                          n1244 = Open/Create/Replace File(file path (use dialog)=w2038, operation (0:open)=T3."open") -> (refnum out=w2051:refnum<file>, error out=w2050:errorcluster)  [unwired: 2 in, 3 out]
                          n1245 = Set File Position(refnum=w2051, from (0:start)=enum16{"start", "end", "current"}."end", error in=w2050) -> (refnum out=w2053:refnum<file>, error out=w2054:errorcluster)  [unwired: 1 in]
                          n1246 = call "RLC_read.vi"("Path"=w2039, "String"="cmd /c rlc_read_ZAN.py") -> ("MEASURE A"=w2036:dbl, "MEASURE V [V]"=w2041:dbl, "MEASURE B"=w2035:dbl, "MEASURE I [A]"=w2040:dbl)  [unwired: 2 out]
                          n1247 = Number To Engineering String(2:w2057, 4:w2040) -> (0:w2043:string)  [unwired: 2 in]
                          n1248 = local write "MEASURE A 10"(w2036) -> ()
                          n1249 = local write "MEASURE B 10"(w2035) -> ()
                          n1250 = Number To Engineering String(2:w2057, 4:w2041) -> (0:w2044:string)  [unwired: 2 in]
                          n1251 = Number To Engineering String(2:w2057, 4:w2036) -> (0:w2046:string)  [unwired: 2 in]
                          n1252 = Number To Engineering String(2:w2057, 4:w2035) -> (0:w2045:string)  [unwired: 2 in]
                          n1253 = Concatenate Strings(w2046, w2042, w2045, w2042, w2044, w2042, w2043, w2042) -> (w2047:string)
                          n1254 = Write to Text File(file (use dialog)=w2053, text=w2047, error in=w2054) -> (refnum out=w2049:refnum<file>, error out=w2048:errorcluster)  [unwired: 1 in, 1 out]
                          n1255 = Close File(refnum=w2049, error in=w2048) -> (error out=w2056:errorcluster)  [unwired: 1 out]
                          n1256 = call <vilib>:"Simple Error Handler.vi"("error in (no error)"=w2056) -> ()  [unwired: 1 in, 8 out]
                        }
                        frame #11 {
                          w2067 = "\t"
                          w2082 = i16 4 ("width (-)")
                          n1257 = Wait (ms)(milliseconds to wait=u32 5000) -> ()  [unwired: 1 out]
                          n1258 = local write "Z-100-L"(w2060) -> ()
                          n1259 = Open/Create/Replace File(file path (use dialog)=w2063, operation (0:open)=T3."open") -> (refnum out=w2076:refnum<file>, error out=w2075:errorcluster)  [unwired: 2 in, 3 out]
                          n1260 = Set File Position(refnum=w2076, from (0:start)=enum16{"start", "end", "current"}."end", error in=w2075) -> (refnum out=w2078:refnum<file>, error out=w2079:errorcluster)  [unwired: 1 in]
                          n1261 = call "RLC_read.vi"("Path"=w2064, "String"="cmd /c rlc_read_ZBL.py") -> ("MEASURE A"=w2062:dbl, "MEASURE V [V]"=w2066:dbl, "MEASURE B"=w2061:dbl, "MEASURE I [A]"=w2065:dbl)  [unwired: 2 out]
                          n1262 = Number To Engineering String(2:w2082, 4:w2065) -> (0:w2068:string)  [unwired: 2 in]
                          n1263 = local write "MEASURE A 11"(w2062) -> ()
                          n1264 = local write "MEASURE B 11"(w2061) -> ()
                          n1265 = Number To Engineering String(2:w2082, 4:w2066) -> (0:w2069:string)  [unwired: 2 in]
                          n1266 = Number To Engineering String(2:w2082, 4:w2062) -> (0:w2071:string)  [unwired: 2 in]
                          n1267 = Number To Engineering String(2:w2082, 4:w2061) -> (0:w2070:string)  [unwired: 2 in]
                          n1268 = Concatenate Strings(w2071, w2067, w2070, w2067, w2069, w2067, w2068, w2067) -> (w2072:string)
                          n1269 = Write to Text File(file (use dialog)=w2078, text=w2072, error in=w2079) -> (refnum out=w2074:refnum<file>, error out=w2073:errorcluster)  [unwired: 1 in, 1 out]
                          n1270 = Close File(refnum=w2074, error in=w2073) -> (error out=w2081:errorcluster)  [unwired: 1 out]
                          n1271 = call <vilib>:"Simple Error Handler.vi"("error in (no error)"=w2081) -> ()  [unwired: 1 in, 8 out]
                        }
                        frame #12 {
                          w2092 = "\t"
                          w2107 = i16 4 ("width (-)")
                          n1272 = Wait (ms)(milliseconds to wait=u32 5000) -> ()  [unwired: 1 out]
                          n1273 = local write "Z-100-N"(w2087) -> ()
                          n1274 = Open/Create/Replace File(file path (use dialog)=w2088, operation (0:open)=T3."open") -> (refnum out=w2101:refnum<file>, error out=w2100:errorcluster)  [unwired: 2 in, 3 out]
                          n1275 = Set File Position(refnum=w2101, from (0:start)=enum16{"start", "end", "current"}."end", error in=w2100) -> (refnum out=w2103:refnum<file>, error out=w2104:errorcluster)  [unwired: 1 in]
                          n1276 = call "RLC_read.vi"("Path"=w2089, "String"="cmd /c rlc_read_ZBN.py") -> ("MEASURE A"=w2086:dbl, "MEASURE V [V]"=w2091:dbl, "MEASURE B"=w2085:dbl, "MEASURE I [A]"=w2090:dbl)  [unwired: 2 out]
                          n1277 = Number To Engineering String(2:w2107, 4:w2090) -> (0:w2093:string)  [unwired: 2 in]
                          n1278 = local write "MEASURE A 12"(w2086) -> ()
                          n1279 = local write "MEASURE B 12"(w2085) -> ()
                          n1280 = Number To Engineering String(2:w2107, 4:w2091) -> (0:w2094:string)  [unwired: 2 in]
                          n1281 = Number To Engineering String(2:w2107, 4:w2086) -> (0:w2096:string)  [unwired: 2 in]
                          n1282 = Number To Engineering String(2:w2107, 4:w2085) -> (0:w2095:string)  [unwired: 2 in]
                          n1283 = Concatenate Strings(w2096, w2092, w2095, w2092, w2094, w2092, w2093, w2092) -> (w2097:string)
                          n1284 = Write to Text File(file (use dialog)=w2103, text=w2097, error in=w2104) -> (refnum out=w2099:refnum<file>, error out=w2098:errorcluster)  [unwired: 1 in, 1 out]
                          n1285 = Close File(refnum=w2099, error in=w2098) -> (error out=w2106:errorcluster)  [unwired: 1 out]
                          n1286 = call <vilib>:"Simple Error Handler.vi"("error in (no error)"=w2106) -> ()  [unwired: 1 in, 8 out]
                        }
                        frame #13 {
                          w2117 = "\t"
                          w2132 = i16 4 ("width (-)")
                          n1287 = local write "Z-1K-L"(w2112) -> ()
                          n1288 = Wait (ms)(milliseconds to wait=u32 5000) -> ()  [unwired: 1 out]
                          n1289 = Open/Create/Replace File(file path (use dialog)=w2113, operation (0:open)=T3."open") -> (refnum out=w2126:refnum<file>, error out=w2125:errorcluster)  [unwired: 2 in, 3 out]
                          n1290 = Set File Position(refnum=w2126, from (0:start)=enum16{"start", "end", "current"}."end", error in=w2125) -> (refnum out=w2128:refnum<file>, error out=w2129:errorcluster)  [unwired: 1 in]
                          n1291 = call "RLC_read.vi"("Path"=w2114, "String"="cmd /c rlc_read_ZCL.py") -> ("MEASURE A"=w2111:dbl, "MEASURE V [V]"=w2116:dbl, "MEASURE B"=w2110:dbl, "MEASURE I [A]"=w2115:dbl)  [unwired: 2 out]
                          n1292 = Number To Engineering String(2:w2132, 4:w2115) -> (0:w2118:string)  [unwired: 2 in]
                          n1293 = local write "MEASURE A 13"(w2111) -> ()
                          n1294 = local write "MEASURE B 13"(w2110) -> ()
                          n1295 = Number To Engineering String(2:w2132, 4:w2116) -> (0:w2119:string)  [unwired: 2 in]
                          n1296 = Number To Engineering String(2:w2132, 4:w2111) -> (0:w2121:string)  [unwired: 2 in]
                          n1297 = Number To Engineering String(2:w2132, 4:w2110) -> (0:w2120:string)  [unwired: 2 in]
                          n1298 = Concatenate Strings(w2121, w2117, w2120, w2117, w2119, w2117, w2118, w2117) -> (w2122:string)
                          n1299 = Write to Text File(file (use dialog)=w2128, text=w2122, error in=w2129) -> (refnum out=w2124:refnum<file>, error out=w2123:errorcluster)  [unwired: 1 in, 1 out]
                          n1300 = Close File(refnum=w2124, error in=w2123) -> (error out=w2131:errorcluster)  [unwired: 1 out]
                          n1301 = call <vilib>:"Simple Error Handler.vi"("error in (no error)"=w2131) -> ()  [unwired: 1 in, 8 out]
                        }
                        frame #14 {
                          w2142 = "\t"
                          w2157 = i16 4 ("width (-)")
                          n1302 = local write "Z-1K-N"(w2137) -> ()
                          n1303 = Wait (ms)(milliseconds to wait=u32 5000) -> ()  [unwired: 1 out]
                          n1304 = Open/Create/Replace File(file path (use dialog)=w2138, operation (0:open)=T3."open") -> (refnum out=w2151:refnum<file>, error out=w2150:errorcluster)  [unwired: 2 in, 3 out]
                          n1305 = Set File Position(refnum=w2151, from (0:start)=enum16{"start", "end", "current"}."end", error in=w2150) -> (refnum out=w2153:refnum<file>, error out=w2154:errorcluster)  [unwired: 1 in]
                          n1306 = call "RLC_read.vi"("Path"=w2139, "String"="cmd /c rlc_read_ZCN.py") -> ("MEASURE A"=w2136:dbl, "MEASURE V [V]"=w2141:dbl, "MEASURE B"=w2135:dbl, "MEASURE I [A]"=w2140:dbl)  [unwired: 2 out]
                          n1307 = Number To Engineering String(2:w2157, 4:w2140) -> (0:w2143:string)  [unwired: 2 in]
                          n1308 = local write "MEASURE A 14"(w2136) -> ()
                          n1309 = local write "MEASURE B 14"(w2135) -> ()
                          n1310 = Number To Engineering String(2:w2157, 4:w2141) -> (0:w2144:string)  [unwired: 2 in]
                          n1311 = Number To Engineering String(2:w2157, 4:w2136) -> (0:w2146:string)  [unwired: 2 in]
                          n1312 = Number To Engineering String(2:w2157, 4:w2135) -> (0:w2145:string)  [unwired: 2 in]
                          n1313 = Concatenate Strings(w2146, w2142, w2145, w2142, w2144, w2142, w2143, w2142) -> (w2147:string)
                          n1314 = Write to Text File(file (use dialog)=w2153, text=w2147, error in=w2154) -> (refnum out=w2149:refnum<file>, error out=w2148:errorcluster)  [unwired: 1 in, 1 out]
                          n1315 = Close File(refnum=w2149, error in=w2148) -> (error out=w2156:errorcluster)  [unwired: 1 out]
                          n1316 = call <vilib>:"Simple Error Handler.vi"("error in (no error)"=w2156) -> ()  [unwired: 1 in, 8 out]
                        }
                        frame #15 {
                          w2167 = "\t"
                          w2182 = i16 4 ("width (-)")
                          n1317 = Wait (ms)(milliseconds to wait=u32 5000) -> ()  [unwired: 1 out]
                          n1318 = local write "Z-10K-L"(w2160) -> ()
                          n1319 = Open/Create/Replace File(file path (use dialog)=w2163, operation (0:open)=T3."open") -> (refnum out=w2176:refnum<file>, error out=w2175:errorcluster)  [unwired: 2 in, 3 out]
                          n1320 = Set File Position(refnum=w2176, from (0:start)=enum16{"start", "end", "current"}."end", error in=w2175) -> (refnum out=w2178:refnum<file>, error out=w2179:errorcluster)  [unwired: 1 in]
                          n1321 = call "RLC_read.vi"("Path"=w2164, "String"="cmd /c rlc_read_ZDL.py") -> ("MEASURE A"=w2162:dbl, "MEASURE V [V]"=w2166:dbl, "MEASURE B"=w2161:dbl, "MEASURE I [A]"=w2165:dbl)  [unwired: 2 out]
                          n1322 = Number To Engineering String(2:w2182, 4:w2165) -> (0:w2168:string)  [unwired: 2 in]
                          n1323 = local write "MEASURE A 15"(w2162) -> ()
                          n1324 = local write "MEASURE B 15"(w2161) -> ()
                          n1325 = Number To Engineering String(2:w2182, 4:w2166) -> (0:w2169:string)  [unwired: 2 in]
                          n1326 = Number To Engineering String(2:w2182, 4:w2162) -> (0:w2171:string)  [unwired: 2 in]
                          n1327 = Number To Engineering String(2:w2182, 4:w2161) -> (0:w2170:string)  [unwired: 2 in]
                          n1328 = Concatenate Strings(w2171, w2167, w2170, w2167, w2169, w2167, w2168, w2167) -> (w2172:string)
                          n1329 = Write to Text File(file (use dialog)=w2178, text=w2172, error in=w2179) -> (refnum out=w2174:refnum<file>, error out=w2173:errorcluster)  [unwired: 1 in, 1 out]
                          n1330 = Close File(refnum=w2174, error in=w2173) -> (error out=w2181:errorcluster)  [unwired: 1 out]
                          n1331 = call <vilib>:"Simple Error Handler.vi"("error in (no error)"=w2181) -> ()  [unwired: 1 in, 8 out]
                        }
                        frame #16 {
                          w2193 = "\t"
                          w2208 = i16 4 ("width (-)")
                          n1332 = Wait (ms)(milliseconds to wait=u32 5000) -> ()  [unwired: 1 out]
                          n1333 = local write "Z-10K-N"(w2187) -> ()
                          n1334 = Open/Create/Replace File(file path (use dialog)=w2188, operation (0:open)=T3."open") -> (refnum out=w2202:refnum<file>, error out=w2201:errorcluster)  [unwired: 2 in, 3 out]
                          n1335 = Set File Position(refnum=w2202, from (0:start)=enum16{"start", "end", "current"}."end", error in=w2201) -> (refnum out=w2204:refnum<file>, error out=w2205:errorcluster)  [unwired: 1 in]
                          n1336 = call "RLC_read.vi"("Path"=w2189, "String"="cmd /c rlc_read_ZDN.py") -> ("MEASURE A"=w2186:dbl, "MEASURE V [V]"=w2192:dbl, "MEASURE B"=w2185:dbl, "MEASURE I [A]"=w2191:dbl)  [unwired: 2 out]
                          n1337 = Number To Engineering String(2:w2208, 4:w2191) -> (0:w2194:string)  [unwired: 2 in]
                          n1338 = local write "MEASURE A 16"(w2186) -> ()
                          n1339 = local write "MEASURE B 16"(w2185) -> ()
                          n1340 = Number To Engineering String(2:w2208, 4:w2192) -> (0:w2195:string)  [unwired: 2 in]
                          n1341 = Number To Engineering String(2:w2208, 4:w2186) -> (0:w2197:string)  [unwired: 2 in]
                          n1342 = Number To Engineering String(2:w2208, 4:w2185) -> (0:w2196:string)  [unwired: 2 in]
                          n1343 = Concatenate Strings(w2197, w2193, w2196, w2193, w2195, w2193, w2194, w2193, "\r\n") -> (w2198:string)
                          n1344 = Write to Text File(file (use dialog)=w2204, text=w2198, error in=w2205) -> (refnum out=w2200:refnum<file>, error out=w2199:errorcluster)  [unwired: 1 in, 1 out]
                          n1345 = Close File(refnum=w2200, error in=w2199) -> (error out=w2207:errorcluster)  [unwired: 1 out]
                          n1346 = call <vilib>:"Simple Error Handler.vi"("error in (no error)"=w2207) -> ()  [unwired: 1 in, 8 out]
                        }
                        frame #17 {
                          n1347 = local write "Z-50-N"(w2211) -> ()
                          n1348 = local write "Z-50-L"(w2211) -> ()
                          n1349 = local write "C-1K-N"(w2211) -> ()
                          n1350 = local write "C-50-N"(w2211) -> ()
                          n1351 = local write "C-50-L"(w2211) -> ()
                          n1352 = local write "Z-1K-N"(w2211) -> ()
                          n1353 = local write "C-1K-L"(w2211) -> ()
                          n1354 = local write "Z-1K-L"(w2211) -> ()
                          n1355 = local write "Z-100-L"(w2211) -> ()
                          n1356 = local write "C-10K-L"(w2211) -> ()
                          n1357 = local write "Z-10K-L"(w2211) -> ()
                          n1358 = local write "C-10K-N"(w2211) -> ()
                          n1359 = local write "Z-10K-N"(w2211) -> ()
                          n1360 = local write "C-100-N"(w2211) -> ()
                          n1361 = local write "C-100-L"(w2211) -> ()
                          n1362 = local write "Z-100-N"(w2211) -> ()
                        }
                      }
                    }
                    n1363 = call <vilib>:"Mean.vi"("X"=w1762) -> ("mean"=w1745:dbl)  [unwired: 1 out]
                    n1364 = call <vilib>:"Mean.vi"("X"=w1761) -> ("mean"=w1744:dbl)  [unwired: 1 out]
                    n1365 = call <vilib>:"Mean.vi"("X"=w1760) -> ("mean"=w1743:dbl)  [unwired: 1 out]
                    n1366 = call <vilib>:"Mean.vi"("X"=w1759) -> ("mean"=w1742:dbl)  [unwired: 1 out]
                    n1367 = call <vilib>:"Mean.vi"("X"=w1758) -> ("mean"=w1741:dbl)  [unwired: 1 out]
                    n1368 = call <vilib>:"Mean.vi"("X"=w1757) -> ("mean"=w1740:dbl)  [unwired: 1 out]
                    n1369 = call <vilib>:"Mean.vi"("X"=w1756) -> ("mean"=w1739:dbl)  [unwired: 1 out]
                    n1370 = call <vilib>:"Mean.vi"("X"=w1755) -> ("mean"=w1738:dbl)  [unwired: 1 out]
                    n1371 = call <vilib>:"Mean.vi"("X"=w1754) -> ("mean"=w1737:dbl)  [unwired: 1 out]
                    n1372 = call <vilib>:"Mean.vi"("X"=w1753) -> ("mean"=w1736:dbl)  [unwired: 1 out]
                    n1373 = call <vilib>:"Mean.vi"("X"=w1752) -> ("mean"=w1735:dbl)  [unwired: 1 out]
                    n1374 = call <vilib>:"Mean.vi"("X"=w1751) -> ("mean"=w1734:dbl)  [unwired: 1 out]
                    n1375 = call <vilib>:"Mean.vi"("X"=w1750) -> ("mean"=w1733:dbl)  [unwired: 1 out]
                    n1376 = call <vilib>:"Mean.vi"("X"=w1749) -> ("mean"=w1732:dbl)  [unwired: 1 out]
                    n1377 = call <vilib>:"Mean.vi"("X"=w1748) -> ("mean"=w1731:dbl)  [unwired: 1 out]
                    n1378 = call <vilib>:"Mean.vi"("X"=w1747) -> ("mean"=w1730:dbl)  [unwired: 1 out]
                    n1379 = local write "mean"(w1745) -> ()
                    n1380 = local write "mean 2"(w1744) -> ()
                    n1381 = local write "mean 3"(w1743) -> ()
                    n1382 = local write "mean 4"(w1742) -> ()
                    n1383 = local write "mean 5"(w1741) -> ()
                    n1384 = local write "mean 6"(w1740) -> ()
                    n1385 = local write "mean 7"(w1739) -> ()
                    n1386 = local write "mean 8"(w1738) -> ()
                    n1387 = local write "mean 9"(w1737) -> ()
                    n1388 = local write "mean 10"(w1736) -> ()
                    n1389 = local write "mean 11"(w1735) -> ()
                    n1390 = local write "mean 12"(w1734) -> ()
                    n1391 = local write "mean 13"(w1733) -> ()
                    n1392 = local write "mean 14"(w1732) -> ()
                    n1393 = local write "mean 15"(w1731) -> ()
                    n1394 = local write "mean 16"(w1730) -> ()
                  }
                }
              }
              frame #2 {
                n1395 = case shown="True" w2213 {
                  tunnel: w2230 -> [_ w2246]
                  tunnel: w2229 -> [_ w2245]
                  tunnel: w2228 -> [_ w2244]
                  tunnel: w2227 -> [_ w2243]
                  tunnel: w2226 -> [_ w2242]
                  tunnel: w2225 -> [_ w2241]
                  tunnel: w2224 -> [_ w2240]
                  tunnel: w2223 -> [_ w2239]
                  tunnel: w2222 -> [_ w2238]
                  tunnel: w2221 -> [_ w2237]
                  tunnel: w2220 -> [_ w2236]
                  tunnel: w2219 -> [_ w2235]
                  tunnel: w2218 -> [_ w2234]
                  tunnel: w2217 -> [_ w2233]
                  tunnel: w2216 -> [_ w2232]
                  tunnel: w2215 -> [_ w2231]
                  frame False {
                  }
                  frame True {
                    w2261 = "\t"
                    w2278 = i16 4 ("precision (6)")
                    n1396 = property on="SET" class="DigNum (strict)"() -> ("Value"=w2247:i32)  [unwired: 2 in, 2 out]
                    n1397 = Number To Engineering String(2:w2278, 4:w2246) -> (0:w2276:string)  [unwired: 2 in]
                    n1398 = Number To Engineering String(2:w2278, 4:w2245) -> (0:w2275:string)  [unwired: 2 in]
                    n1399 = Number To Engineering String(2:w2278, 4:w2244) -> (0:w2274:string)  [unwired: 2 in]
                    n1400 = Number To Engineering String(2:w2278, 4:w2243) -> (0:w2273:string)  [unwired: 2 in]
                    n1401 = Number To Engineering String(2:w2278, 4:w2242) -> (0:w2272:string)  [unwired: 2 in]
                    n1402 = Number To Engineering String(2:w2278, 4:w2241) -> (0:w2271:string)  [unwired: 2 in]
                    n1403 = Number To Engineering String(2:w2278, 4:w2240) -> (0:w2270:string)  [unwired: 2 in]
                    n1404 = Number To Engineering String(2:w2278, 4:w2239) -> (0:w2269:string)  [unwired: 2 in]
                    n1405 = Number To Engineering String(2:w2278, 4:w2238) -> (0:w2268:string)  [unwired: 2 in]
                    n1406 = Number To Engineering String(2:w2278, 4:w2237) -> (0:w2267:string)  [unwired: 2 in]
                    n1407 = Number To Engineering String(2:w2278, 4:w2231) -> (0:w2266:string)  [unwired: 2 in]
                    n1408 = Number To Engineering String(2:w2278, 4:w2236) -> (0:w2265:string)  [unwired: 2 in]
                    n1409 = Number To Engineering String(2:w2278, 4:w2235) -> (0:w2264:string)  [unwired: 2 in]
                    n1410 = Number To Engineering String(2:w2278, 4:w2234) -> (0:w2263:string)  [unwired: 2 in]
                    n1411 = Number To Engineering String(2:w2278, 4:w2233) -> (0:w2262:string)  [unwired: 2 in]
                    n1412 = Number To Engineering String(2:w2278, 4:w2232) -> (0:w2260:string)  [unwired: 2 in]
                    n1413 = Number To Decimal String(number=w2247) -> (decimal integer string=w2277:string)  [unwired: 1 in]
                    n1414 = property on="path RLC_mean" class="Path"() -> ("Value"=w2248:path)  [unwired: 2 in, 2 out]
                    n1415 = Open/Create/Replace File(file path (use dialog)=w2248, operation (0:open)=T3."open") -> (refnum out=w2253:refnum<file>, error out=w2252:errorcluster)  [unwired: 2 in, 3 out]
                    n1416 = Concatenate Strings(w2277, w2261, w2276, w2261, w2275, w2261, w2274, w2261, w2273, w2261, w2272, w2261, w2271, w2261, w2270, w2261, w2269, w2261, w2268, w2261, w2267, w2261, w2266, w2261, w2265, w2261, w2264, w2261, w2263, w2261, w2262, w2261, w2260, "\r\n") -> (w2249:string)
                    n1417 = Set File Position(refnum=w2253, from (0:start)=enum16{"start", "end", "current"}."end", error in=w2252) -> (refnum out=w2255:refnum<file>, error out=w2256:errorcluster)  [unwired: 1 in]
                    n1418 = Write to Text File(file (use dialog)=w2255, text=w2249, error in=w2256) -> (refnum out=w2251:refnum<file>, error out=w2250:errorcluster)  [unwired: 1 in, 1 out]
                    n1419 = Close File(refnum=w2251, error in=w2250) -> (error out=w2258:errorcluster)  [unwired: 1 out]
                    n1420 = call <vilib>:"Simple Error Handler.vi"("error in (no error)"=w2258) -> ()  [unwired: 1 in, 8 out]
                  }
                }
              }
            }
            n1421 = local write "graph RLC"(w1685) -> ()
          }
        }
        n1422 = call <vilib>:"Linear Fit.vi"("Y"=w1658, "X"=w1662) -> ("Best Linear Fit"=w1660:dbl[], "slope"=→"bar/N":dbl)  [unwired: 9 in, 3 out]
        n1423 = Bundle(w1662, w1658) -> (w1665:cluster{i32[], dbl[]})  [unwired: 1 in]
        n1424 = call <vilib>:"General Polynomial Fit.vi"("Y"=w1667, "polynomial order"=w1683, "X"=w1662) -> ("Best Polynomial Fit"=w1679:dbl[], "Polynomial Coefficients"=w1680:dbl[])  [unwired: 9 in, 2 out]
        "Polynomial Coefficients 2" <- w1680
        n1425 = call <vilib>:"General Polynomial Fit.vi"("Y"=w1658, "polynomial order"=w1683, "X"=w1676) -> ("Best Polynomial Fit"=w1661:dbl[], "Polynomial Coefficients"=w1674:dbl[])  [unwired: 9 in, 2 out]
        "Polynomial Coefficients" <- w1674
        n1426 = Bundle(w1662, "Best Polynomial Fit"=w1661) -> (w1664:cluster{i32[], "Best Polynomial Fit":dbl[]})  [unwired: 1 in]
        n1427 = Build Array(w1667, w1679) -> (→"Linear Model Graph 2":dbl[][])
        n1428 = Index Array(array=w1674, index=0) -> (element=→"p fit":dbl)
        n1429 = Index Array(array=w1680, index=0) -> (element=→"T fit":dbl)
        n1430 = Build Array(w1658, w1661, w1660) -> (→"Linear Model Graph":dbl[][])
        n1431 = Bundle(w1662, "Best Linear Fit"=w1660) -> (w1663:cluster{i32[], "Best Linear Fit":dbl[]})  [unwired: 1 in]
        n1432 = Build Array(w1665, w1664, w1663) -> ()  [unwired: 1 out]
      }
    }
    n1433 = case shown="True" "Close RLC 2" {
      tunnel: w36 -> [_ w166]
      frame False {
      }
      frame True {
        n1434 = call "RLC_close.vi"("Path"=w166) -> ("String"=w167:string)  [unwired: 10 in]
        n1435 = local write "RLC300 - digimess"(w167) -> ()
      }
    }
    n1436 = case shown="True" "Open Button 2" {
      frame False {
      }
      frame True {
        n1437 = property on="Sample name" class="Str"() -> ("Value"=w1637:string)  [unwired: 2 in, 2 out]
        n1438 = property on="File name" class="Str"() -> ("Value"=w1638:string)  [unwired: 2 in, 2 out]
        n1439 = property on="Nota" class="Str"() -> ("Value"=w1636:string)  [unwired: 2 in, 2 out]
        n1440 = call "Open file.vi"("Nota 01"=w1636, "Sample name"=w1637, "File name"=w1638) -> ("path open old"=w1635:path)  [unwired: 8 in]
        n1441 = local write "path"(w1635) -> ()
      }
    }
    n1442 = case shown="True" "Refresh Button 2" {
      frame False {
      }
      frame True {
        n1443 = property on="Waveform Chart" class="WFChart (strict)"("History Data"=dynamicdata[] []) -> ()  [unwired: 2 in, 2 out]
      }
    }
    n1444 = case shown="True" "Open Button" {
      frame False {
      }
      frame True {
        n1445 = flat-sequence {
          tunnel: ["Sample name"] -> w1641
          tunnel: ["Nota"] -> w1640
          tunnel: [w1643] -> w1639
          tunnel: w1641 -> [w1656]
          tunnel: w1640 -> [w1655]
          tunnel: w1639 -> [w1650]
          frame #0 {
            n1446 = local write "Count SET"(0 ("Count SET")) -> ()
            n1447 = local write "Set atual"(0 ("Count  3")) -> ()
            n1448 = call "File_data_new.vi"("Nota 01"="Nota", "Sample name"="Sample name", "File name"="File name") -> ("path"=w1643:path)  [unwired: 8 in]
            "path" <- w1643
          }
          frame #1 {
            w1651 = FALSE
            n1449 = Strip Path(path=w1650) -> (stripped path=w1649:path, name=w1648:string)
            n1450 = local write "Pf2"(w1651) -> ()
            n1451 = local write "ZPit"(w1651) -> ()
            n1452 = local write "Pit"(w1651) -> ()
            n1453 = local write "ZPf2"(w1651) -> ()
            n1454 = local write "T"(w1651) -> ()
            n1455 = Concatenate Strings(w1648, "_cinetica" ("string")) -> (w1653:string)
            n1456 = call "File_data_cinetica.vi"("path in"=w1649, "Nota 01"=w1655, "Sample name"=w1656, "File name"=w1653) -> ("path"=→"path 2_cinetica":path)  [unwired: 7 in]
          }
        }
      }
    }
    n1457 = local write "Manual Ctrl"(w49) -> ()
    n1458 = Or(x=w39, y=w38) -> (x .or. y?=w40:bool)
    n1459 = Or(x=w40, y="Refresh Button") -> (x .or. y?=w42:bool)
    n1460 = case shown="True" w42 {
      frame False {
      }
      frame True {
        n1461 = stacked-sequence {
          frame #0 {
            n1462 = property on="Waveform Chart P 2" class="WFChart (strict)"("History Data"=dbl[][] []) -> ()  [unwired: 2 in, 2 out]
          }
          frame #1 {
            n1463 = property on="path RLC_mean" class="Path"() -> ("Value"=w72:path)  [unwired: 2 in, 2 out]
            n1464 = Open/Create/Replace File(file path (use dialog)=w72, operation (0:open)=T3."open", access (0:read/write)=enum16{"read/write", "read-only", "write-only"}."read-only") -> (refnum out=w76:refnum<file>, error out=w75:errorcluster)  [unwired: 3 in, 1 out]
            n1465 = Read from Text File(file (use dialog)=w76, error in=w75) -> (refnum out=w81:refnum<file>, text=w77:string, error out=w80:errorcluster)  [unwired: 2 in, 1 out]
            n1466 = Close File(refnum=w81, error in=w80) -> ()  [unwired: 2 out]
            n1467 = Search/Split String(string=w77, search string/char (-)="SET\tDATE\tTIME\t\tP (BAR)\tT (ºC)\tC-50-L\tC-50-N\tC-100-L\tC-100-N\tC-1K-L\tC-1K-N\tC-10K-L\tC-10K-N\tZ-50-L\tZ-50-N\tZ-100-L\tZ-100-N\tZ-1K-L\tZ-1K-N\tZ-10K-L\tZ-10K-N") -> (match + rest of string=w82:string)  [unwired: 1 in, 2 out]
            n1468 = String Subset(string=w82, offset (0)=150) -> (substring=w89:string)  [unwired: 1 in]
            n1469 = Spreadsheet String To Array(format string="%#g", spreadsheet string=w89) -> (array=w88:dbl[][])  [unwired: 2 in]
            n1470 = Transpose Matrix(1:w88) -> (0:w102:dbl[][])
            n1471 = Index Array(array=w102, index (row)=1 ("index (row) 4")) -> (element=w103:dbl[])  [unwired: 1 in]
            n1472 = Index Array(array=w102, index (row)=2 ("index (row) 5")) -> (element=w104:dbl[])  [unwired: 1 in]
            n1473 = Index Array(array=w102, index (row)=3 ("index (row) 2")) -> (element=w105:dbl[])  [unwired: 1 in]
            n1474 = Index Array(array=w102, index (row)=4 ("index (row) 3")) -> (element=w106:dbl[])  [unwired: 1 in]
            n1475 = Index Array(array=w102, index (row)=5 ("index (row) 4")) -> (element=w107:dbl[])  [unwired: 1 in]
            n1476 = Index Array(array=w102, index (row)=6 ("index (row) 5")) -> (element=w108:dbl[])  [unwired: 1 in]
            n1477 = Index Array(array=w102, index (row)=7 ("index (row) 2")) -> (element=w109:dbl[])  [unwired: 1 in]
            n1478 = Index Array(array=w102, index (row)=8 ("index (row) 3")) -> (element=w110:dbl[])  [unwired: 1 in]
            n1479 = Index Array(array=w102, index (row)=9 ("index (row) 4")) -> (element=w71:dbl[])  [unwired: 1 in]
            n1480 = Index Array(array=w102, index (row)=10 ("index (row) 5")) -> (element=w70:dbl[])  [unwired: 1 in]
            n1481 = Index Array(array=w102, index (row)=11 ("index (row) 2")) -> (element=w69:dbl[])  [unwired: 1 in]
            n1482 = Index Array(array=w102, index (row)=12 ("index (row) 3")) -> (element=w68:dbl[])  [unwired: 1 in]
            n1483 = Index Array(array=w102, index (row)=13 ("index (row) 4")) -> (element=w67:dbl[])  [unwired: 1 in]
            n1484 = Index Array(array=w102, index (row)=14 ("index (row) 5")) -> (element=w66:dbl[])  [unwired: 1 in]
            n1485 = Index Array(array=w102, index (row)=15 ("index (row) 2")) -> (element=w65:dbl[])  [unwired: 1 in]
            n1486 = Index Array(array=w102, index (row)=16 ("index (row) 3")) -> (element=w64:dbl[])  [unwired: 1 in]
            n1487 = Build Array(w103, w104, w105, w106, w107, w108, w109, w110, w71, w70, w69, w68, w67, w66, w65, w64) -> (w63:dbl[][])
            n1488 = Transpose Matrix(1:w63) -> (0:→"Waveform Chart P 2":dbl[][])
          }
        }
      }
    }
  }
  n1489 = local write "path 2_cinetica"(path "C:/H2_Painel/painel_auto/cinetica.txt" ("path")) -> ()
  n1490 = local write "path RLC_completo"(path "C:/H2_Painel/painel_auto/RLC_full.txt" ("path RLC_mean")) -> ()
  n1491 = local write "path RLC_mean"(path "C:/H2_Painel/painel_auto/RLC_mean.txt" ("path RLC_mean")) -> ()
  n1492 = local write "path"(path "C:/H2_Painel/painel_auto/Arquivo_Padrao.txt" ("path")) -> ()
  n1493 = local write "Array"(dbl[] [0.5, 1.0, 2.0, 3.0, 4.0, 4.0, 4.0, 4.0, 4.0, 4.0, 4.0, 5.0, 5.0, 5.0, 7.0, 10.0, 15.0, 20.0, 25.0, 25.0, 25.0, 30.0, 40.0, 50.0, 60.0, 70.0] ("Array")) -> ()
